vi "MAIN - PECT - Autonics - Pulses - encoder - Multi-sensor - Huy.vi"() -> ()   [LabVIEW 2018]
uses:
  Pulsed Eddy Current - DATN Huy/Control 1.ctl
  <vilib>/DAQmx/read.llb/DAQmx Read (Counter U32 1Chan 1Samp).vi
  <vilib>/DAQmx/write.llb/DAQmx Write (Analog 1D Wfm NChan NSamp).vi
  <vilib>/DAQmx/read.llb/DAQmx Read (Analog 1D Wfm NChan NSamp).vi
  <vilib>/DAQmx/create/channels.llb/DAQmx Create Channel (AI-Voltage-Basic).vi
  <vilib>/NI/Modbus Library/API/Wrapper/Create Serial Master.vi
  <vilib>/DAQmx/create/channels.llb/DAQmx Create Channel (CI-Count Edges).vi
  <vilib>/DAQmx/miscellaneous.llb/DAQmx Fill In Error Info.vi
  <vilib>/DAQmx/configure/timing.llb/DAQmx Timing (Sample Clock).vi
  <vilib>/DAQmx/configure/trigger.llb/DAQmx Start Trigger (Digital Edge).vi
  <vilib>/DAQmx/create/channels.llb/DAQmx Create Channel (AO-Voltage-Basic).vi
  Pulsed Eddy Current - DATN Huy/Global_data.vi
  <vilib>/measure/maspectr.llb/FFT Power Spectrum and PSD for 1 Chan.vi
  <vilib>/NI/Modbus Library/API/Master/Modbus Master.lvclass
  <resource>/objmgr/daqmx.rc
  <vilib>/Platform/NI_3dgraph.lvlib
  <vilib>/measure/NI_MAPro.lvlib
  <vilib>/NI/Modbus Library/API/Wrapper/API Main.lvlib
panel:
  out "Init pulses":i32
  out "Z complete":bool
  out "X complete":bool
  out "Y complete":bool=TRUE
  out "exception status":u8=1
  out "Limit Sensor":bool[](array[boolean])
  out "Y Back Limit":bool
  out "X L Limit":bool
  out "Z UP Limit":bool
  out "Numeric  4":i32=3413
  out "Enum 2":T1(ring)=enum."Wait Y"
  in  "Stop Scan":bool
  out "Step Y Number":i16=20
  out "Count Y step":i32=6
  out "No. Y 2":i32=7
  in  "Open tdms 2":bool
  in  "Backdata 3":bool
  in  "low cutoff freq: fl 4":dbl=40.0 format="%0.2f"
  in  "Filter 4":bool
  out "dy 2":dbl[][](array[numeric])
  in  "DiffX 2":bool caption="Scan"
  in  "DiffY 2":bool caption="Scan"
  in  "Odd 2":bool caption="Scan"
  in  "Abs 2":bool caption="Scan"
  in  "Backdata 2":bool caption="Scan"
  in  "Backindex 2":i32
  in  "low cutoff freq: fl 3":dbl=40.0 format="%0.2f"
  in  "Filter 3":bool caption="Scan"
  in  "Line Row 2":dbl
  in  "Line Col 2":dbl=167.0
  in  "Repair Line Row 2":bool
  in  "Repair Line Col 2":bool
  in  "Trim data 2":bool caption="Scan"
  in  "X-min 2":dbl
  in  "X-max 2":dbl=319.0
  in  "Y-min 2":dbl
  in  "Y-max 2":dbl=55.0
  in  "Inverse  2":bool caption="Scan"
  in  "Return 2":bool caption="Scan"
  in  "ColorMapAutoScale 2":bool=TRUE
  in  "Min 2":dbl=-0.004
  in  "Max 2":dbl=0.004
  in  "Cursor 2":bool=TRUE
  out "Out Hall":dbl[][](array[numeric])=[[0.17776170515535383, 0.1724938890045491, 0.17567422492724655, 0.17281948891164128, 0.17750249452676287, 0.17174255590976084, 0.17689848816282988, 0.0, 0.0, 0.0, 0.0, 0.0, 0.0, 0.0, 0.0, 0.0, 0.0, 0.0, 0.0, 0.0, 0.0], [0.181110419736364, 0.17834435597274723, 0.17901593566948365, 0.17843396121396082, 0.18082391275549609, 0.17677177439859865, 0.1805733450890007, 0.0, 0.0, 0.0, 0.0, 0.0, 0.0, 0.0, 0.0, 0.0, 0.0, 0.0, 0.0, 0.0, 0.0], [0.1901443502075802, 0.1807788163690286, 0.18389219629241077, 0.18292101264388094, 0.18584253413825647, 0.18424340027016872, 0.1844692257000472, 0.0, 0.0, 0.0, 0.0, 0.0, 0.0, 0.0, 0.0, 0.0, 0.0, 0.0, 0.0, 0.0, 0.0], [0.19675174630430725, 0.19133976157012406, 0.19610529224489537, 0.18647717964306243, 0.19791131101721843, 0.19044015693607824, 0.19720754713146932, 0.0, 0.0, 0.0, 0.0, 0.0, 0.0, 0.0, 0.0, 0.0, 0.0, 0.0, 0.0, 0.0, 0.0], [0.20248230005231593, 0.1980001562954143, 0.2026130769874166, 0.19908381606183906, 0.20400329640988507, 0.19691764965481123, 0.2026434189867065, 0.0, 0.0, 0.0, 0.0, 0.0, 0.0, 0.0, 0.0, 0.0, 0.0, 0.0, 0.0, 0.0, 0.0], [0.20756282207197274, 0.20355937318454292, 0.2074345242175782, 0.20456099056442495, 0.2083181459314682, 0.202307939377475, 0.20759286833282414, 0.0, 0.0, 0.0, 0.0, 0.0, 0.0, 0.0, 0.0, 0.0, 0.0, 0.0, 0.0, 0.0, 0.0], [0.2161886923639197, 0.21253974725757924, 0.21125259878099184, 0.20908024033946615, 0.2168660930291072, 0.21166435694559893, 0.21165270992196006, 0.0, 0.0, 0.0, 0.0, 0.0, 0.0, 0.0, 0.0, 0.0, 0.0, 0.0, 0.0, 0.0, 0.0], [0.2201899331796135, 0.21690643861065811, 0.2201028334105652, 0.2176118553302127, 0.2208123356772303, 0.21536349521145187, 0.21956557074351502, 0.0, 0.0, 0.0, 0.0, 0.0, 0.0, 0.0, 0.0, 0.0, 0.0, 0.0, 0.0, 0.0, 0.0], [0.22206492093457092, 0.22076373224143442, 0.22107829951788738, 0.221511549643648, 0.22260408488962002, 0.21964691546696985, 0.22123030620827921, 0.0, 0.0, 0.0, 0.0, 0.0, 0.0, 0.0, 0.0, 0.0, 0.0, 0.0, 0.0, 0.0, 0.0], [0.2236337254628875, 0.22214151901015816, 0.22332887383646616, 0.22254736085515114, 0.2241084117751464, 0.22218723394057438, 0.22207453511184994, 0.0, 0.0, 0.0, 0.0, 0.0, 0.0, 0.0, 0.0, 0.0, 0.0, 0.0, 0.0, 0.0, 0.0], [0.22318899958521138, 0.22380028818012027, 0.22211272800173293, 0.22360354843226388, 0.22304326181333678, 0.22145899165729238, 0.21932588351591875, 0.0, 0.0, 0.0, 0.0, 0.0, 0.0, 0.0, 0.0, 0.0, 0.0, 0.0, 0.0, 0.0, 0.0], [0.22290047278312458, 0.2235340533472822, 0.2222785786896101, 0.22290675514178815, 0.22322972419052123, 0.22156789245679248, 0.22010562695733926, 0.0, 0.0, 0.0, 0.0, 0.0, 0.0, 0.0, 0.0, 0.0, 0.0, 0.0, 0.0, 0.0, 0.0], [0.22356747769441365, 0.2241092575777761, 0.2223606596149607, 0.2229985011040989, 0.2225818108464972, 0.22200716436702206, 0.21966538751675208, 0.0, 0.0, 0.0, 0.0, 0.0, 0.0, 0.0, 0.0, 0.0, 0.0, 0.0, 0.0, 0.0, 0.0], [0.22053633383678345, 0.2227234349622484, 0.22003048978407946, 0.22234284825731204, 0.21996511082210407, 0.22033336393759062, 0.21762783729986052, 0.0, 0.0, 0.0, 0.0, 0.0, 0.0, 0.0, 0.0, 0.0, 0.0, 0.0, 0.0, 0.0, 0.0], [0.21927133576270147, 0.21955591604432806, 0.21646450772183934, 0.21896512302724214, 0.21808932704173967, 0.21754658610019562, 0.21354951646025394, 0.0, 0.0, 0.0, 0.0, 0.0, 0.0, 0.0, 0.0, 0.0, 0.0, 0.0, 0.0, 0.0, 0.0], [0.2185139029939545, 0.21825674506426196, 0.21672810294608302, 0.21719225251047203, 0.2163638216728313, 0.2157054295509772, 0.21285135223872376, 0.0, 0.0, 0.0, 0.0, 0.0, 0.0, 0.0, 0.0, 0.0, 0.0, 0.0, 0.0, 0.0, 0.0], [0.21491616995167662, 0.21811390913005718, 0.21464911868266495, 0.21696465474188015, 0.21574170384074837, 0.21470166777781502, 0.21233935567094664, 0.0, 0.0, 0.0, 0.0, 0.0, 0.0, 0.0, 0.0, 0.0, 0.0, 0.0, 0.0, 0.0, 0.0], [0.2134545034639892, 0.2143867692168009, 0.21070345133335106, 0.21436238496967602, 0.2114824144487502, 0.21274445669186648, 0.20671707318008187, 0.0, 0.0, 0.0, 0.0, 0.0, 0.0, 0.0, 0.0, 0.0, 0.0, 0.0, 0.0, 0.0, 0.0], [0.21091214938658065, 0.21277905859725532, 0.20836885096431412, 0.21055566864121245, 0.20950337819485593, 0.20888585192838677, 0.20574571324326885, 0.0, 0.0, 0.0, 0.0, 0.0, 0.0, 0.0, 0.0, 0.0, 0.0, 0.0, 0.0, 0.0, 0.0], [0.21109980585640742, 0.21000105081453663, 0.2080156676992811, 0.20958712361967385, 0.20811188508169193, 0.20736163569155075, 0.2047283842510788, 0.0, 0.0, 0.0, 0.0, 0.0, 0.0, 0.0, 0.0, 0.0, 0.0, 0.0, 0.0, 0.0, 0.0]]
  in  "Save Scan mode 2":bool caption="Save Process"
  in  "Filter 2":bool
  in  "low cutoff freq: fl 2":dbl=40.0 format="%0.2f"
  in  "Backdata":bool
  out "Init pulses":i32
  out "dy":dbl[][](array[numeric])
  in  "2D Array In":dbl[][](array[numeric])
  out "Output Coil":dbl[][](array[numeric])=[[0.18553710534904855, 0.17973457254507935, 0.18427423395187004, 0.18042918126533436, 0.18645887887248153, 0.1801573678387421, 0.18645082000465146, 0.0, 0.0, 0.0, 0.0, 0.0, 0.0, 0.0, 0.0, 0.0, 0.0, 0.0, 0.0, 0.0, 0.0], [0.18987014602319247, 0.18653261167773033, 0.18990582291953773, 0.18740225957772644, 0.1914559394951999, 0.18644683758905045, 0.191481439134582, 0.0, 0.0, 0.0, 0.0, 0.0, 0.0, 0.0, 0.0, 0.0, 0.0, 0.0, 0.0, 0.0, 0.0], [0.20219420650083397, 0.19081774860606898, 0.1952789240855507, 0.1921933722869305, 0.19679175738266869, 0.19602858652538785, 0.19738356640856358, 0.0, 0.0, 0.0, 0.0, 0.0, 0.0, 0.0, 0.0, 0.0, 0.0, 0.0, 0.0, 0.0, 0.0], [0.20939136336324898, 0.20337450420146508, 0.20975638146138104, 0.19793745902051413, 0.21076173268511106, 0.2028610093026868, 0.21149030184929252, 0.0, 0.0, 0.0, 0.0, 0.0, 0.0, 0.0, 0.0, 0.0, 0.0, 0.0, 0.0, 0.0, 0.0], [0.21622055514910743, 0.2109998977268851, 0.21654153178439584, 0.21186750773282248, 0.21747992176888825, 0.21001144013201994, 0.2178259938557714, 0.0, 0.0, 0.0, 0.0, 0.0, 0.0, 0.0, 0.0, 0.0, 0.0, 0.0, 0.0, 0.0, 0.0], [0.22096639968031884, 0.21613883575961468, 0.22106121776896787, 0.21769696957735463, 0.2229345689672355, 0.2160350775631949, 0.22254631882683024, 0.0, 0.0, 0.0, 0.0, 0.0, 0.0, 0.0, 0.0, 0.0, 0.0, 0.0, 0.0, 0.0, 0.0], [0.22918239447852007, 0.22482125577754608, 0.2251534307015154, 0.22210101570727897, 0.2301739477211303, 0.22526210600970953, 0.22650893519159931, 0.0, 0.0, 0.0, 0.0, 0.0, 0.0, 0.0, 0.0, 0.0, 0.0, 0.0, 0.0, 0.0, 0.0], [0.23072867440456596, 0.2279499722265652, 0.23049599246595942, 0.22892309217776513, 0.23257180417432533, 0.22825736261999474, 0.2320123360222584, 0.0, 0.0, 0.0, 0.0, 0.0, 0.0, 0.0, 0.0, 0.0, 0.0, 0.0, 0.0, 0.0, 0.0], [0.23185337710758436, 0.22989669056911782, 0.2307016748936201, 0.23044598289982565, 0.23299357137415944, 0.23058981164836756, 0.2319131657399408, 0.0, 0.0, 0.0, 0.0, 0.0, 0.0, 0.0, 0.0, 0.0, 0.0, 0.0, 0.0, 0.0, 0.0], [0.22630211132749595, 0.2303770249129905, 0.2282483576289565, 0.23086049593072017, 0.23095666864614767, 0.23114931892992713, 0.22934701981393596, 0.0, 0.0, 0.0, 0.0, 0.0, 0.0, 0.0, 0.0, 0.0, 0.0, 0.0, 0.0, 0.0, 0.0], [0.2215102649364752, 0.22374474076562317, 0.2191382524314066, 0.22801369409819444, 0.22283327835507083, 0.22548194556609513, 0.22129294280866907, 0.0, 0.0, 0.0, 0.0, 0.0, 0.0, 0.0, 0.0, 0.0, 0.0, 0.0, 0.0, 0.0, 0.0], [0.21763039136450935, 0.21929122157454478, 0.21572879699955255, 0.2193674469881774, 0.21916521798106897, 0.22116497510888178, 0.21738430074877346, 0.0, 0.0, 0.0, 0.0, 0.0, 0.0, 0.0, 0.0, 0.0, 0.0, 0.0, 0.0, 0.0, 0.0], [0.21335832760298545, 0.215211494733674, 0.21125095473051608, 0.2160083891793727, 0.21476909785799747, 0.21737423005943346, 0.21311533591657172, 0.0, 0.0, 0.0, 0.0, 0.0, 0.0, 0.0, 0.0, 0.0, 0.0, 0.0, 0.0, 0.0, 0.0], [0.20135894511959307, 0.21145853750149302, 0.2048206322299499, 0.21082245427422058, 0.20181948963267182, 0.20702943348605823, 0.2070025081380047, 0.0, 0.0, 0.0, 0.0, 0.0, 0.0, 0.0, 0.0, 0.0, 0.0, 0.0, 0.0, 0.0, 0.0], [0.19432880055987894, 0.19771187558020858, 0.19098523549555563, 0.1977787364919263, 0.19570997510151694, 0.20082611415153734, 0.19373654419199682, 0.0, 0.0, 0.0, 0.0, 0.0, 0.0, 0.0, 0.0, 0.0, 0.0, 0.0, 0.0, 0.0, 0.0], [0.18896822798166024, 0.19168506258678636, 0.18632412497380157, 0.19159648646157518, 0.1906377348289004, 0.19408935512459574, 0.18912258943210353, 0.0, 0.0, 0.0, 0.0, 0.0, 0.0, 0.0, 0.0, 0.0, 0.0, 0.0, 0.0, 0.0, 0.0], [0.18009702280244988, 0.18712015799094445, 0.1825546829225686, 0.1875327275883079, 0.18680820041773105, 0.18988062347566131, 0.18488384150052983, 0.0, 0.0, 0.0, 0.0, 0.0, 0.0, 0.0, 0.0, 0.0, 0.0, 0.0, 0.0, 0.0, 0.0], [0.17377109719426687, 0.17674354692231936, 0.1701534372729802, 0.18307701834693768, 0.17476744955718027, 0.17999467046652273, 0.17298889884516222, 0.0, 0.0, 0.0, 0.0, 0.0, 0.0, 0.0, 0.0, 0.0, 0.0, 0.0, 0.0, 0.0, 0.0], [0.16752395847442747, 0.17063904093338916, 0.16462749541368465, 0.17056002142642612, 0.16910895941204906, 0.17404342521037897, 0.16819677725831522, 0.0, 0.0, 0.0, 0.0, 0.0, 0.0, 0.0, 0.0, 0.0, 0.0, 0.0, 0.0, 0.0, 0.0], [0.16324428563434706, 0.16559024570855152, 0.16156797333915018, 0.16574386859680224, 0.16542079327972803, 0.1678753304123673, 0.16521948417362342, 0.0, 0.0, 0.0, 0.0, 0.0, 0.0, 0.0, 0.0, 0.0, 0.0, 0.0, 0.0, 0.0, 0.0]]
  in  "Tab Control 3":enum32{"Control", "Data Processing"}(tab)
  in  "Pulser Trigger":tag="/Dev1/PFI0"
  in  "Edge":i32(ring)=10280 items=["Rising"=10280, "Falling"=10171]
  in  "2 Plots":bool
  in  "Offset":bool
  in  "Gate 1":dbl
  in  "Gate 2":dbl=20.0
  in  "Tab Control 4":enum32{"Basic", "Gaussian", "Chirp"}(tab)
  in  "Pulse Basic":T3={"Basic amp"=1.0, "Duty cycle %"=50.0, "Basic freq (Hz)"=50, "Basic Type"=2} {"Basic Type" items=["Sine Wave", "Triangle Wave", "Square Wave", "Sawtooth Wave"]; "Duty cycle %" format="%#.2f"; "Basic amp" format="%0.2p"}
  in  "Pulse Gaussian":T4={"Gauss amp"=2.5, "Gauss Nor. Band"=0.5, "Gauss atten (dB)"=6.0, "Gauss freq (Hz)"=1000.0}
  in  "Pulse chirp":T5={"Chirp amp"=2.1, "Chirp f2"=1500.0, "Chirp f1"=500.0} {"Chirp f1" format="%0.2f"; "Chirp f2" format="%0.2f"; "Chirp amp" format="%0.2f"}
  in  "Gate 3":dbl
  in  "Gate 4":dbl=20.0
  in  "Stop Button":bool
  in  "X Distance":u32=100
  in  "X RIGHT":bool
  in  "X LEFT":bool
  in  "Y Distance":u32=100
  in  "Y FW":bool
  in  "Y BW":bool
  in  "Z Distance":i16=1
  in  "Up Z":bool
  in  "Down Z":bool
  in  "Home 2":bool
  in  "Speed (mm/s) 2":i16=6
  in  "Scan":bool
  in  "Open tdms":bool
  in  "Save Scan mode":bool caption="Save Process"
  in  "Open csv":bool
  in  "Exit":bool
  in  "Cursor":bool=TRUE
  in  "Repair Line Col":bool
  in  "Repair Line Row":bool
  in  "Line Col":dbl=167.0
  in  "Line Row":dbl
  in  "Y-max":dbl=55.0
  in  "Y-min":dbl
  in  "X-max":dbl=319.0
  in  "X-min":dbl
  in  "Inverse":bool caption="Scan"
  in  "ViewMode":i32(ring) items=["cwViewXYPlane", "cwViewXZPlane", "cwViewYZPlane", "cwViewUserDefined"]
  in  "Plot style":i32(ring)=4 items=["cwLine"=1, "cwPoint"=2, "cwLinePoint"=3, "cwHiddenLine"=4, "cwSurface"=5, "cwSurfaceLine"=6, "cwSurfaceNormal"=7, "cwContourLine"=8, "cwSurfaceContour"=9]
  in  "ColorMapAutoScale":bool=TRUE
  in  "Max":dbl=0.029
  in  "Min":dbl=-0.030999999999999996
  in  "low cutoff freq: fl":dbl=40.0 format="%0.2f"
  in  "Filter":bool caption="Scan"
  in  "Backindex":i32
  in  "Backdata":bool caption="Scan"
  in  "Odd":bool caption="Scan"
  in  "DiffX":bool caption="Scan"
  in  "DiffY":bool caption="Scan"
  in  "Abs":bool caption="Scan"
  in  "Trim data":bool caption="Scan"
  in  "Return":bool caption="Scan"
  in  "Tab Control 2":T6(tab)
  in  "Tab plot":enum32{"Raw Signal Plot", "Phase Plot"}(tab)
  out "Hall sensors signal":waveform(dbl)[](graph)=[{"t0"=timestamp(3844381406.018446 s since 1904-01-01), "dt"=3.9999999999999996e-05, "Y"=array[500 elements], "attributes"=variant("NI_ChannelName"=variant(string "Acquisition Task0"), "NI_UnitDescription"=variant(string "Volts"))}, {"t0"=timestamp(3844381406.018446 s since 1904-01-01), "dt"=3.9999999999999996e-05, "Y"=array[500 elements], "attributes"=variant("NI_ChannelName"=variant(string "Acquisition Task0"), "NI_UnitDescription"=variant(string "Volts"))}]
  out "Coil signal":waveform(dbl)[](graph)=[{"t0"=timestamp(3844381406.0184684 s since 1904-01-01), "dt"=3.9999999999999996e-05, "Y"=array[500 elements], "attributes"=variant("NI_ChannelName"=variant(string "Acquisition Task2"), "NI_UnitDescription"=variant(string "Volts"))}, {"t0"=timestamp(3844381406.0184684 s since 1904-01-01), "dt"=3.9999999999999996e-05, "Y"=array[500 elements], "attributes"=variant("NI_ChannelName"=variant(string "Acquisition Task2"), "NI_UnitDescription"=variant(string "Volts"))}]
  out "Phase - Single Hall (0)":cluster{dbl[], "Signal out":dbl[]}[](graph)
  out "Phase - Differential Hall (2)":cluster{dbl[], "Signal out":dbl[]}[](graph)
  out "Feature Extraction Hall":dbl(graph)=0.07041561460174023
  out "Power spectral density Hall":cluster{"f0":dbl, "df":dbl, "magnitude":dbl[]}[](graph)=[{"f0"=0.0, "df"=50.00000000000001, "magnitude"=[0.05344226538018011, 0.49428645675976, 0.17848329749409506, 0.030177691736389706, 0.015779343521924998, 0.006320257971197771, 0.0038168470703960067, 0.0019964659184224885, 0.0013194607149625986, 0.0007909208207930289, 0.0005535851326366026, 0.000358756224441028, 0.0002600365059727909, 0.00017878857903978157, 0.0001359454988281132, 9.993266647353149e-05, 7.753702165794456e-05, 5.8386048558759755e-05, 4.549840057742934e-05, 3.3454980244959085e-05, 2.6622987044468742e-05, 1.9250486167782837e-05, 1.4534022978169584e-05, 1.3228498606348696e-05, 1.2150027857478272e-05, 9.502579643267317e-06, 7.855867434071126e-06, 7.01638103886502e-06, 6.372515227454497e-06, 4.999969117815732e-06, 3.84393580456763e-06, 3.0917208279441807e-06, 2.4082253245390505e-06, 2.0891651026755156e-06, 2.1987810684143896e-06, 1.7457276008966685e-06, 1.3664085555342715e-06, 1.3673912753577668e-06, 1.2138009817051083e-06, 8.606682950932153e-07, 8.041900765492353e-07, 8.749099163659475e-07, 8.132829202518184e-07, 6.822494594419114e-07, 6.049051591521565e-07, 6.132992125073271e-07, 5.773547451807314e-07, 5.506540953194728e-07, 4.3351203976864175e-07, 1.8527694293227517e-07, 1.0481643805680082e-07, 1.195257630817566e-07, 1.1577574640733723e-07, 1.3401572515625924e-07, 1.6216287991758492e-07, 1.186876125279046e-07, 9.060456692020551e-08, 1.3456818799714813e-07, 1.0510266739217573e-07, 3.142357380666471e-08, 1.4252605291150848e-08, 4.94727416899243e-08, 9.493752501187421e-08, 7.628840934796899e-08, 8.59941417276983e-08, 2.117415858805495e-07, 1.81493780415358e-07, 4.825218961205501e-08, 4.191163413423024e-08, 6.441735733140098e-08, 3.4493211155460755e-08, 1.4815146399129527e-08, 2.7635500338646048e-08, 3.31043326742198e-08, 1.2413938930169236e-08, 1.457617162360193e-08, 3.7426355027452554e-08, 8.043740401609367e-08, 1.2269684347819443e-07, 1.246734981592159e-07, 5.2624356236721426e-08, 4.463962736770971e-08, 6.268161110233025e-08, 2.646498245870502e-08, 9.27204135176441e-09, 5.687475791202217e-09, 4.3602539744288816e-08, 5.527470937058986e-08, 1.727347402766435e-08, 2.5880201919013012e-08, 3.474778084083779e-08, 9.148097678816275e-09, 1.3421076340763538e-08, 8.00016733276709e-09, 2.2985544027964692e-08, 2.5069409405287202e-08, 3.0328634642511167e-08, 1.0224838076248899e-08, 9.378180566466623e-10, 2.873099772018073e-08, 1.334279919522608e-07, 1.8727262848664548e-07, 1.3332056211683505e-07, 8.726903720317449e-08, 1.03971846440294e-07, 6.718232618882674e-08, 1.3880802636736537e-08, 3.9650360677896445e-08, 1.2859794341213376e-07, 1.0679933330923813e-07, 5.107625956135357e-08, 5.343601180982578e-08, 5.5313249665534265e-08, 5.1826870346456046e-08, 7.183493774751532e-08, 6.437520957424805e-08, 4.280825959178591e-08, 2.543086465599578e-08, 1.6763998967314607e-08, 3.5619661064757844e-08, 4.890137024737889e-08, 6.082773646809916e-08, 5.888222718893705e-08, 4.1628475463044077e-08, 4.42698534942595e-08, 6.214635675712085e-08, 8.99759237288563e-08, 1.3448108318958237e-07, 6.113750683434083e-08, 2.103047358584125e-08, 2.8362017906722262e-08, 5.481610867729404e-08, 1.0688808193659075e-07, 1.7274313715049422e-07, 1.914756881569332e-07, 1.1306438838635857e-07, 5.2813427257792266e-08, 3.996199556144808e-08, 2.2697571013294733e-08, 5.734483892419069e-10, 2.8081260393893844e-08, 2.8880224924120155e-08, 4.898407391043184e-08, 5.664197632494949e-08, 2.8532162294421515e-08, 2.8853144610438315e-08, 5.559791052549845e-08, 4.446329519051906e-08, 1.6680834898830503e-08, 3.5650802925485585e-08, 3.848002231692065e-08, 1.9680536607976463e-08, 2.7851839333979786e-08, 3.8933105523131193e-08, 2.87184748099256e-08, 2.0485065158311178e-08, 4.136069598939249e-08, 7.319940383893738e-08, 8.004455591882947e-08, 9.602410245361758e-08, 6.666789751788917e-08, 4.995816124195714e-08, 6.683357512271323e-08, 1.0087542956994011e-07, 6.827798428718567e-08, 5.4876548151163396e-08, 5.744632982652637e-08, 4.929962484905926e-08, 2.9032444367342632e-08, 1.522487958403537e-08, 2.026435224314862e-08, 5.0457006209631696e-08, 8.373272899679024e-08, 1.0790271945291921e-07, 7.018845544482759e-08, 2.411772863403995e-08, 2.360453514128649e-08, 4.077274184419568e-08, 7.648209134497276e-08, 1.2781018650491652e-07, 1.6002774083664143e-07, 2.0770049365059966e-07, 1.303222414400018e-07, 4.1368308120012236e-08, 6.4160316739485e-08, 1.0099067934493672e-07, 5.38019209498868e-08, 4.4635898377098715e-08, 5.9315721166343063e-08, 7.226181891616877e-08, 7.063800286754404e-08, 8.760300104088728e-08, 6.872173578943062e-08, 5.8742115186723415e-08, 7.553788068378707e-08, 8.671207764860681e-08, 9.022251590094401e-08, 5.9593987724185115e-08, 3.582920024686291e-08, 5.798093672933093e-08, 9.499750095191987e-08, 6.926474282663654e-08, 3.293710896704422e-08, 2.8245758802593293e-08, 2.47091803072218e-08, 1.2647196881118485e-08, 6.454242521098473e-08, 2.056831730517149e-07, 3.485617433452981e-07, 1.440427212693921e-07, 8.937883626262774e-08, 6.045562377904082e-08, 7.760808515413506e-08, 7.78449152515259e-08, 1.330054212144905e-07, 8.371828606658445e-08, 8.561279979854768e-08, 5.4805119006428505e-08, 1.9338255465860983e-08, 3.683299630853313e-08, 1.2478751634611085e-07, 1.16562391672607e-07, 6.171400516822817e-08, 3.763791730789338e-08, 5.177315424560907e-08, 1.0221161051269428e-08, 1.6685563679185154e-08, 7.024939423457463e-08, 3.8696218795106824e-08, 4.90292594838444e-08, 7.457546634166207e-08, 3.9335458612916186e-08, 4.519700704403511e-08, 5.1748360032004634e-08, 4.5665543598436463e-08, 4.248858006809279e-08, 1.6997037841459297e-08, 3.430110823042511e-08, 1.0024033470712759e-07, 2.5382392312075055e-07, 2.3195388950002645e-07, 9.90307775433233e-08, 4.93160412832673e-08, 5.42909961897056e-08, 8.79319646977936e-08, 1.1705999824246691e-07, 9.089424254070586e-08, 8.65613061805912e-08, 4.3020212897029436e-08, 2.947213234013073e-08]}, ...(2 in all)]
  in  "Add LF":bool
  in  "Save LF":bool caption="Save Process"
  out "Save Status":bool
  out "Power spectral density Coil":cluster{"f0":dbl, "df":dbl, "magnitude":dbl[]}[](graph)=[{"f0"=0.0, "df"=50.00000000000001, "magnitude"=[0.06471500798999083, 0.10490788754209399, 0.024608636483418194, 0.00438296652656786, 0.002353975865329042, 0.0009930276997905318, 0.0006133065242780386, 0.00033234531696222833, 0.00022234291389610391, 0.00013599912790488415, 9.635500158173878e-05, 6.385727017592712e-05, 4.6859522684514546e-05, 3.264012477373104e-05, 2.494329649951874e-05, 1.8795482156107153e-05, 1.4930372858996385e-05, 1.1087730773346793e-05, 8.699885164366403e-06, 6.843723008639812e-06, 5.317177853272812e-06, 3.41854349089057e-06, 2.36216089696049e-06, 2.1094327824092687e-06, 2.0368607532845296e-06, 1.6593921378545388e-06, 1.4388189907875578e-06, 1.2481486541694899e-06, 1.0642889452659768e-06, 8.613808389720096e-07, 7.482731111154614e-07, 6.136253742461639e-07, 4.81930548536851e-07, 3.954701004182598e-07, 3.513657300513881e-07, 3.238765422331869e-07, 3.0808559066308883e-07, 2.574714929256103e-07, 2.006304851630887e-07, 1.7232288780124035e-07, 1.74089583300975e-07, 2.0239764287870447e-07, 1.5608094005219732e-07, 9.48375551237609e-08, 6.48312719107151e-08, 6.950179885773663e-08, 7.350122180875951e-08, 5.508849073841518e-08, 5.071471481648698e-08, 4.917024594063803e-08, 3.927019581297804e-08, 2.865493472218875e-08, 3.042033750079982e-08, 6.356484151502967e-08, 1.131628012005958e-07, 8.770917166116928e-08, 3.849460559005413e-08, 2.2406249338970256e-08, 2.937327972394305e-08, 3.310271947962208e-08, 1.1549285476783957e-08, 1.7582027257628245e-09, 1.4746810230328445e-08, 2.807809650305719e-08, 1.6582601363499622e-08, 9.220284715723395e-09, 7.0570358343042344e-09, 6.103347806248802e-09, 4.221061890242989e-09, 3.29155017051343e-09, 7.897537312045454e-09, 1.4800804144644369e-08, 4.440147699567223e-09, 1.0836774053742844e-09, 5.201310588053047e-09, 5.118692316685894e-09, 3.876120411759733e-09, 8.967137960534486e-09, 9.553480760753523e-09, 1.1845491620801643e-08, 2.3465172488569197e-08, 9.095409630592785e-09, 8.058804655606744e-11, 1.240856877775084e-09, 1.7554291563382184e-09, 1.622786769483243e-09, 4.420811206107678e-09, 1.373011919379434e-09, 9.06932764250493e-10, 6.434932109627647e-09, 5.347572186368814e-09, 5.105133310237453e-10, 1.5238772528762543e-09, 3.293426245111752e-10, 1.9485625928318283e-09, 6.049833707988641e-10, 1.718304607563343e-10, 2.6250789895257948e-09, 5.5550450795021446e-09, 2.7634365616250577e-08, 9.411828662332091e-09, 3.4355126362302166e-09, 1.6483930375292411e-09, 3.867637310330051e-10, 8.189858566467442e-10, 4.2588387800610776e-10, 1.61835031977466e-10, 2.626872780519488e-10, 8.581641561567351e-11, 7.80504543979124e-12, 3.2469404845402755e-10, 1.7766378925106262e-09, 6.077120737227311e-09, 2.821313239672745e-09, 5.32267129177698e-10, 6.266532314362268e-10, 1.3521566313179728e-09, 5.191683970545212e-09, 1.163702854741034e-08, 2.0866295709393846e-09, 1.2920350149377133e-09, 6.107268669825776e-09, 1.6234830727552773e-10, 1.7218304307096456e-09, 8.998944730098978e-10, 5.603077667795519e-10, 2.0224103608600164e-11, 8.075749738337876e-10, 8.721436588670355e-10, 3.719772495742986e-09, 1.0053169486957145e-08, 5.732860604673989e-09, 6.783660147802078e-09, 7.387782843284888e-09, 1.993319164824313e-09, 1.6871109342383448e-09, 3.851787498335101e-09, 7.602739813531432e-09, 2.6373743491907912e-09, 5.2367883185127045e-09, 1.570231387120171e-08, 1.09351649028092e-08, 4.232403685987372e-10, 1.4075809200037895e-09, 2.787101906083711e-09, 1.0243605792229125e-09, 1.5243819649117444e-09, 3.2668878550539542e-09, 7.165093854380813e-10, 7.178026024792953e-10, 7.163021793593579e-10, 4.871253272759402e-10, 3.3689325374539587e-10, 9.053388742882745e-11, 8.47060497268097e-11, 2.1652333307865178e-09, 5.191374000359224e-09, 3.3378619778986655e-09, 9.376805315277407e-10, 6.08880694148336e-09, 1.799287902931768e-08, 1.2384703881624945e-08, 5.638582625124952e-09, 6.089830350784959e-09, 4.625327984411809e-09, 4.797001785380629e-10, 3.671051025949149e-10, 8.53389739031635e-11, 1.5881648376439475e-09, 3.4395750302534926e-09, 2.0484015898175548e-10, 1.0876714876357938e-09, 1.6779654532955758e-09, 5.983518496933457e-10, 1.3703546979604813e-09, 3.2035261954833246e-09, 7.810457738849178e-09, 7.2786525235643386e-09, 1.831757381309426e-09, 6.583986610268209e-09, 4.140399669972484e-10, 9.225786631998565e-09, 1.3840054204595343e-09, 1.3087651452104364e-09, 5.772885567196273e-11, 6.238654484291674e-10, 8.446631955649547e-10, 9.60692639300278e-10, 2.2946669800416606e-09, 4.706636927790736e-09, 1.7195422401010414e-09, 6.01554636790235e-11, 1.642314657027999e-10, 2.8796861842033897e-10, 3.2576579035771345e-09, 1.8622191268493826e-09, 1.9406625842261643e-10, 1.3260249218513399e-11, 2.159251486310598e-09, 1.6170719715144243e-10, 1.1601067375548019e-08, 3.5900131143046976e-09, 9.364895039775729e-09, 3.445950995939315e-09, 3.0458082145416376e-09, 7.482201199742227e-09, 1.1097609412351321e-08, 1.3446550609020134e-08, 1.489395795604217e-08, 1.0079340393933278e-08, 6.315023670817954e-09, 4.357683135105497e-09, 1.49205808331129e-09, 7.839934048851647e-11, 2.4283097582485266e-09, 1.345921525360762e-09, 1.959664996621814e-09, 2.205548803551967e-09, 2.101968548459717e-09, 6.37233042080121e-11, 4.613313544458869e-09, 3.1937453382577165e-09, 2.458251239608534e-10, 6.862155147694832e-10, 2.5231468014641028e-09, 1.1876874679348104e-09, 2.242941481809397e-10, 1.7173319537765193e-09, 1.7737522349175943e-09, 6.66562449000842e-10, 4.2473960553661253e-11, 1.937616215730229e-10, 1.8322341333968375e-10, 1.0073689561157657e-09, 8.497702108980565e-10, 7.862843619019232e-10, 4.355940466970832e-09, 9.144546500898896e-10, 2.5311893509022874e-09, 1.604116612745175e-08, 1.2890611449264356e-08, 3.7170575844336277e-09, 2.0417543694612313e-09, 3.639916957099234e-09, 5.6594996184529875e-09, 2.903222776721938e-09, 3.3605212419772653e-09, 2.0340648284100022e-08, 1.408153004705747e-08, 5.873974395123851e-09]}, ...(2 in all)]
  out "Feature Extraction Coil":dbl(graph)=0.1511557759031275
  out "Save Status 2":bool
  in  "3D Surface(0) (coil)":refnum<k7>(container)
  out "Record path":path=path "C:/Users/ADMIN/Downloads/PECT_default.tdms" caption="selected path"
  out "Feature extraction scan Coil":dbl[](graph)
  in  "3D Surface (2)(Hall)":refnum<k7>(container)
  out "Feature extraction scan Hall":dbl[](graph)
  out "Record path 2":path=path "C:/Users/ADMIN/Downloads/PECT2_default.tdms" caption="selected path"
  in  "View Mode":bool caption="Scan"
  out "Hall sensors signal lf":dbl[][](graph)=[[-0.70660846198, -0.716567731313, -0.71772803455, -0.717921418426, -0.720596562008, -0.722079171705, -0.724657623384, -0.723561781416, -0.729298836376, -0.728847607304, -0.733553281611, -0.731232675116, -0.734068971955, -0.734230125187, -0.734649123582, -0.735197044564, -0.737292036575, -0.735906118769, -0.738162264033, -0.736454039766, -0.735454889741, -0.737968880154, -0.735422659102, -0.737292036581, -0.734552431644, -0.735809426849, -0.731909518652, -0.731264905752, -0.726591462081, -0.727171613726, -0.72340062815, -0.721080021693, -0.715278505501, -0.71253890069, -0.707188613582, -0.701870557272, -0.697068191179, -0.692362517146, -0.687946918849, -0.677826496722, -0.674571201711, -0.663773936246, -0.660776486438, -0.651622983945, -0.644113244288, -0.636120045089, -0.629867300614, -0.618425422989, -0.610399993434, -0.59950603696, -0.59218968167, -0.58322956384, -0.571207535404, -0.564471331877, -0.553126147145, -0.546615558225, -0.534915836753, -0.528792015616, -0.520315358066, -0.514803919133, -0.504103347861, -0.497753912499, -0.490534250062, -0.48415258421, -0.4781254554, -0.472839631231, -0.469197569495, -0.467811652195, -0.46571666097, -0.462429136198, -0.467457115235, -0.467231500771, -0.474354471106, -0.474741238726, -0.482927820085, -0.490469788806, -0.499204291135, -0.509066865834, -0.523216115386, -0.534432377128, -0.554350911396, -0.569177005115, -0.58816085171, -0.612366062487, -0.634250667901, -0.66187232831, -0.688269225307, -0.719081721676, -0.746928999864, -0.781093486223, -0.813130751347, -0.851227380515, -0.888357092222, -0.928000797226, -0.965807357181, -1.008351826422, -1.048994689492, -1.09189370194, -1.13485717869, -1.180109036257, -1.2251352826, -1.266293851833, -1.314639865003, -1.35380013893, -1.401147008934, -1.441370901989, -1.48307740981, -1.522592234217, -1.561881446939, -1.594208832793, -1.628276678402, -1.656575231322, -1.685228323683, -1.708627813295, -1.726709237842, -1.745338585167, -1.754749951221, -1.765386084343, -1.766481928394, -1.766578620469, -1.759068865834, -1.749141808352, -1.726870391409, -1.702697363978, -1.672142659225, -1.635496354594, -1.591855992024, -1.542736415895, -1.486816169566, -1.426544787201, -1.357119898907, -1.281152192711, -1.205055574576, -1.115615471107, -1.027496838527, -0.924487655795, -0.823476790057, -0.71266782326, -0.598377964549, -0.477738687781, -0.356454816131, -0.226146385508, -0.096933813379, 0.039691785785, 0.177477671952, 0.315553620416, 0.456562543074, 0.59605661768, 0.738386978448, 0.878138885599, 1.019921318004, 1.154935322631, 1.292076548544, 1.418613908244, 1.546504957955, 1.665822671713, 1.781143796386, 1.887472587349, 1.990352709737, 2.080759590593, 2.164752584475, 2.235692182322, 2.298122899903, 2.352689348501, 2.387788500997, 2.419503438832, 2.429204857999, 2.432524612792, 2.418181983039, 2.390753718718, 2.346694452024, 2.29477091497, 2.222380935278, 2.137904477937, 2.035346650361, 1.920347813654, 1.791425361517, 1.644195932762, 1.485299034053, 1.310738069287, 1.125154243505, 0.921650202866, 0.71092650171, 0.483765177519, 0.253445229601, 0.008105779367, -0.246129373952, -0.508261099919, -0.779449723152, -1.058244889529, -1.341584711586, -1.635528585329, -1.928441259944, -2.223868134907, -2.526772774422, -2.823650514512, -3.124106146674, -3.41405481644, -3.706227714753, -3.987442417835, -4.263822791101, -4.527407776882, -4.786577416573, -5.02840704592, -5.262275871216, -5.475098028081, -5.677574208879, -5.860454027961, -6.026509320014, -6.174450790588, -6.300217254762, -6.406645020668, -6.487352250666, -6.552781862445, -6.587011551361, -6.605834660103, -6.593973522799, -6.560743004097, -6.502017506172, -6.420568948967, -6.309918874295, -6.178350774499, -6.019772990024, -5.841921080871, -5.636479455639, -5.407702708707, -5.163100759281, -4.889329996495, -4.60340849308, -4.29102572782, -3.966589007543, -3.624329025262, -3.267791211866, -2.894429352616, -2.512784620922, -2.118957082525, -1.720230866355, -1.310095339563, -0.893610688781, -0.473226398891, -0.047749885035, 0.377081857903, 0.806651402224, 1.226326113266, 1.646645459066, 2.057327931374, 2.465367624173, 2.856937640696, 3.240772514315, 3.608041067282, 3.955230157274, 4.293975068757, 4.609804197942, 4.90271751193, 5.177098363499, 5.426887322034, 5.649860408204, 5.851142279943, 6.021772700426, 6.172194436626, 6.288354759714, 6.38169561436, 6.443353457295, 6.479452149573, 6.483029788153, 6.46127387881, 6.407834927929, 6.330674003129, 6.221217696105, 6.086943623705, 5.925176659162, 5.736206928573, 5.524965806055, 5.286167477957, 5.029771319924, 4.744593282131, 4.446168641795, 4.123506733751, 3.788113950506, 3.432351621052, 3.06650133258, 2.685180548865, 2.296898136162, 1.899107838935, 1.494871524426, 1.086445286821, 0.675762909712, 0.265467248353, -0.150952337452, -0.55870204758, -0.972221258056, -1.373654237756, -1.777923829368, -2.168979184481, -2.552460698049, -2.920729689806, -3.280071163481, -3.622008401497, -3.950860315772, -4.258117910152, -4.550936409787, -4.823256343074, -5.072595856712, -5.304498634402, -5.509682053404, -5.698202166799, -5.859132548236, -6.000240858013, -6.111889905191, -6.206424214181, -6.27008099717, -6.315365963394, -6.333898960157, -6.329676659853, -6.305148642671, -6.25857442753, -6.185216035338, -6.09506518857, -5.986381425725, -5.856360663809, -5.709708700472, -5.54117189352, -5.365641079165, -5.166356100054, -4.957401996174, -4.734878834588, -4.502332058483, -4.25769890765, -4.007715673153, -3.745098175872, -3.482835479658, -3.212193012196, -2.937618633024, -2.664784953904, -2.386601188071, -2.116185239442, -1.843835631437, -1.575257184583, -1.307226809354, -1.048865766862, -0.789924683906, -0.543553647601, -0.298858680926, -0.065186650983, 0.160975596988, 0.377855392589, 0.583937909112, 0.777321550784, 0.961906228802, 1.129988834268, 1.286113886493, 1.434406905534, 1.559977352138, 1.681841284773, 1.782239637185, 1.87196966226, 1.947711605492, 2.009916693762, 2.057166778279, 2.095037754511, 2.114505048262, 2.126913836672, 2.123561852274, 2.106834160961, 2.083724807448, 2.04517698859, 1.999828510872, 1.941362174369, 1.876127411384, 1.800417702224, 1.720518017024, 1.626759173182, 1.53477301667, 1.432666452766, 1.3256930704, 1.216753623473, 1.100658983649, 0.982533816097, 0.864892106737, 0.741448886061, 0.618489120633, 0.497011957912, 0.371215886709, 0.252865078568, 0.127455756566, 0.00929831228, -0.108053378055, -0.221569636608, -0.333216531681, -0.440351151746, -0.547066787125, -0.643984321714, -0.742481170629, -0.834016212751, -0.919943133402, -1.004129610016, -1.078743591058, -1.154131117554, -1.220526296559, -1.28176457554, -1.335299729295, -1.389318348703, -1.430928160202, -1.472151206875, -1.504381894686, -1.533711822363, -1.557723687612, -1.576417489536, -1.58798830868, -1.597464132915, -1.601750815379, -1.601621892616, -1.59852774587, -1.588246154234, -1.580027327232, -1.560882295453, -1.54560494743, -1.52268892626, -1.50177120885, -1.474117278751, -1.447236886611, -1.415296278632, -1.385869665753, -1.349996918726, -1.315800169399, -1.280926577982, -1.245472836775, -1.210728172549, -1.170472066246, -1.137048863988, -1.097276222791, -1.065400096546, -1.027077839927, -0.994814949512, -0.958942227201, -0.927646259992, -0.892128078709, -0.861283343899, -0.830664225057, -0.801817793355, -0.772777978979, -0.746928999873, -0.722723784605, -0.697132652466, -0.677504190288, -0.654072512801, -0.640019952773, -0.620713798494, -0.607112468066, -0.589804614323, -0.577589201926, -0.565986171871, -0.555930212629, -0.54590648416, -0.539105819592, -0.533239843546, -0.528050710938, -0.523635113662, -0.51996082103, -0.521346738438, -0.518703826188, -0.521314507795, -0.519896359761, -0.525472259972, -0.524408648935, -0.530177933006, -0.532079540602, -0.538815743842, -0.541813193149, -0.548871702871, -0.55319060837, -0.559572274784, -0.565953941223, -0.570885229012, -0.57865281302, -0.584647711969, -0.594349134521, -0.597120969574, -0.607305851908, -0.611399143265, -0.6213584113, -0.626902081599, -0.634282898507, -0.640019952747, -0.647046232714, -0.651300677507, -0.657295577056, -0.662162404096, -0.668737455294, -0.674216664635, -0.675602582331, -0.683531320648, -0.684949468998, -0.693136052559, -0.694167433224, -0.700516870141, -0.703095321724, -0.708961299059, -0.708219994242, -0.711443058732], [-0.711700903907, -0.720274255531, -0.721080021681, -0.724464239466, -0.722433708801, -0.725141083016, -0.72559231207, -0.726204694336, -0.729202144406, -0.727848457275, -0.731039291205, -0.729975679907, -0.73139382833, -0.73123267509, -0.734165663872, -0.732392978358, -0.735648273607, -0.732908668699, -0.73590611877, -0.734810276807, -0.73352105101, -0.733843357422, -0.732844207425, -0.733230975136, -0.731007060611, -0.73062029283, -0.728106302452, -0.729427758908, -0.724174163692, -0.726043541112, -0.72166017329, -0.721208944256, -0.715181813577, -0.712248824884, -0.70754315068, -0.704739084581, -0.697809495981, -0.693361667074, -0.688849376879, -0.681694173927, -0.676311656471, -0.666481310252, -0.663677244331, -0.654942740122, -0.649270147063, -0.638827419012, -0.632703597094, -0.62161625644, -0.613816441327, -0.601891104324, -0.593382215333, -0.583906407255, -0.574301676729, -0.564729176965, -0.553480684115, -0.54616432927, -0.535624910724, -0.527373867557, -0.517382370077, -0.511258549117, -0.498881984754, -0.493789544277, -0.484603813104, -0.479898140329, -0.472710708686, -0.46910087758, -0.464072898546, -0.462042368558, -0.459721762867, -0.45836807625, -0.458948227649, -0.460366375577, -0.465104278851, -0.467167039506, -0.476352770465, -0.481703055936, -0.495368845435, -0.504619038035, -0.520702125685, -0.534819144789, -0.554447603261, -0.570530691961, -0.592511988075, -0.615621357208, -0.640535643041, -0.667319306976, -0.694973199311, -0.727912918571, -0.7584675715, -0.795017126404, -0.828988231267, -0.870404618505, -0.908050021807, -0.951432484146, -0.989754736086, -1.033685125354, -1.077228749861, -1.121674836208, -1.166572155322, -1.211276093955, -1.257140340429, -1.302521130597, -1.347934155322, -1.389930731637, -1.437535450536, -1.478565113577, -1.521947620419, -1.557949302468, -1.598431053803, -1.629565906268, -1.663762677273, -1.691223234113, -1.718941638241, -1.740310595099, -1.759874633465, -1.772831377568, -1.782081590668, -1.788237655914, -1.788173194541, -1.784176586682, -1.7728636083, -1.758134175287, -1.733090917251, -1.706693971085, -1.669886510205, -1.632917898781, -1.584314009521, -1.53206805716, -1.471442131748, -1.407141915873, -1.333398119264, -1.254561886613, -1.168796071461, -1.07871136044, -0.983147451101, -0.877076363675, -0.77200444347, -0.655490661079, -0.541426425506, -0.414760028952, -0.290317564379, -0.158687687189, -0.026832212351, 0.113370977212, 0.253509690839, 0.395968995891, 0.538202675996, 0.682209031094, 0.82640876359, 0.965999515658, 1.107943100394, 1.2432149505, 1.379195876537, 1.506635696159, 1.632560682823, 1.748236342269, 1.865201233481, 1.969338348306, 2.067416114716, 2.15692054372, 2.236530178481, 2.30560040478, 2.364485757723, 2.409930942223, 2.44470779056, 2.468332842109, 2.474327739345, 2.470137757407, 2.448124237269, 2.417408447956, 2.366355134083, 2.304955792292, 2.22576515062, 2.134197956683, 2.022454403625, 1.899978065497, 1.759420364327, 1.606872887466, 1.438564653815, 1.256074962083, 1.059951729476, 0.851161868759, 0.630478906609, 0.399030903911, 0.159009529445, -0.095741280337, -0.355101129604, -0.628997073303, -0.906148413194, -1.193065765257, -1.484979020361, -1.782984050494, -2.083052046727, -2.385956572993, -2.689473733606, -2.994473784422, -3.295767585382, -3.589680826897, -3.885270392832, -4.167097682705, -4.447442674322, -4.711382413403, -4.969939881134, -5.21305896681, -5.445155293591, -5.65475453306, -5.853298698642, -6.032053093797, -6.193563935177, -6.333222102904, -6.451672172544, -6.551138064005, -6.625721405834, -6.678709764359, -6.705397338156, -6.7118436127, -6.689732892102, -6.647219721964, -6.571991743565, -6.476812606234, -6.354849306761, -6.207552308847, -6.03563076211, -5.840825219647, -5.620911798473, -5.380693017663, -5.114625193963, -4.828993469243, -4.526666463854, -4.200843492433, -3.861516208625, -3.502302924475, -3.13216385381, -2.744427224852, -2.350406050506, -1.943944235937, -1.534034129331, -1.111328792601, -0.688108072092, -0.254348183817, 0.180185043615, 0.614653678333, 1.048574325895, 1.479626447166, 1.903394510606, 2.321264488474, 2.731753822843, 3.124806592014, 3.511768013492, 3.874782309212, 4.221391454251, 4.556655670645, 4.868101642753, 5.155503714809, 5.423470852265, 5.66481553335, 5.882245096744, 6.070795930585, 6.233626609533, 6.371091627426, 6.475326584487, 6.555807348401, 6.601285277357, 6.622976737884, 6.609955415071, 6.570891451368, 6.499628742443, 6.407544849292, 6.28052263845, 6.128070288235, 5.948608528303, 5.743491108137, 5.514426315553, 5.258964657354, 4.982101962969, 4.683548195569, 4.366655388863, 4.026975726542, 3.675113132109, 3.302687625615, 2.924912076204, 2.52876527563, 2.127365065353, 1.717166033533, 1.303228338131, 0.883199090654, 0.465587113791, 0.041722314718, -0.374858506392, -0.792632058415, -1.209664560433, -1.619703313065, -2.022973968836, -2.416640254231, -2.801153418931, -3.170164003204, -3.529376856542, -3.867414465728, -4.195654308351, -4.499141189584, -4.786964188961, -5.051871271029, -5.297149939141, -5.518352233991, -5.717154105289, -5.893104251006, -6.046299304766, -6.173645008773, -6.275238003521, -6.35791128069, -6.408675593623, -6.444194505839, -6.448062264612, -6.433687095446, -6.394268196495, -6.335252674733, -6.248389341404, -6.145345955566, -6.020353152397, -5.879180364564, -5.71757311064, -5.538109933487, -5.346721406584, -5.136058870085, -4.916694164197, -4.681472020658, -4.438804768894, -4.185340402521, -3.926783816261, -3.653465746224, -3.381437188134, -3.103252801735, -2.823908360859, -2.542275774546, -2.258999645662, -1.980912873448, -1.705791511432, -1.431605004604, -1.161544171119, -0.901281584442, -0.641986021923, -0.394615883648, -0.147374738228, 0.083364272888, 0.312008253063, 0.526470734451, 0.730973938979, 0.921811355892, 1.10391427476, 1.267806902505, 1.422997270747, 1.563135951752, 1.687868408833, 1.801094545084, 1.89701284902, 1.981811596561, 2.050430579225, 2.106834160953, 2.147799278231, 2.17816052264, 2.190633772981, 2.194823753727, 2.183317421989, 2.162238596067, 2.128299753321, 2.084208266714, 2.0311889008, 1.967017743996, 1.893370789696, 1.81256864297, 1.725739375948, 1.627307093536, 1.528359125728, 1.41655114942, 1.30799846779, 1.188100615371, 1.068557301022, 0.944695085629, 0.822992319382, 0.695069043221, 0.570272131299, 0.442284382926, 0.317616379586, 0.194624359058, 0.068441497018, -0.050553949051, -0.171128708146, -0.285160663856, -0.399676092901, -0.508132177389, -0.615073436322, -0.712184363585, -0.810874605876, -0.899960127607, -0.986692823527, -1.067462858994, -1.142721461342, -1.214112393046, -1.278251431973, -1.337298031367, -1.389382810045, -1.440339520092, -1.481240260618, -1.520884007654, -1.548602401773, -1.57802902429, -1.595723675412, -1.612902636098, -1.621959461795, -1.628502293261, -1.629275830005, -1.627986602099, -1.618188470277, -1.608358107981, -1.59524021497, -1.575482799408, -1.556627844048, -1.531455674043, -1.507895039751, -1.477243655394, -1.44794596169, -1.414168204733, -1.38277552038, -1.345710238439, -1.31270602436, -1.274061444278, -1.238059782054, -1.200704434038, -1.16164086315, -1.124865672142, -1.086188874377, -1.050283915983, -1.013218656049, -0.978731850936, -0.941376519413, -0.91175654708, -0.874530142074, -0.846586166678, -0.814258824097, -0.786379312543, -0.757500652045, -0.731554981564, -0.705641542641, -0.684433778674, -0.659003801079, -0.639955491476, -0.622712098238, -0.603212560587, -0.590352535192, -0.573463680108, -0.562601954829, -0.551933613494, -0.542554497827, -0.532853075905, -0.529694473448, -0.52025089677, -0.519058363199, -0.513837000046, -0.511451932947, -0.512870080968, -0.511838700566, -0.511677547393, -0.514352690234, -0.517285678205, -0.520508741861, -0.526568101624, -0.527825096497, -0.538493437484, -0.540427275726, -0.547389093516, -0.553061685838, -0.559540044149, -0.566147325069, -0.57620328444, -0.578652813016, -0.588676541915, -0.596540818049, -0.602116718805, -0.61207598672, -0.616749429656, -0.626450852631, -0.6339605921, -0.639955491487, -0.645563623199, -0.654459280486, -0.657263346399, -0.666739155394, -0.66922091493, -0.67573150487, -0.681823096537, -0.68501393027, -0.690783215552, -0.69532773638, -0.698035110534, -0.70357878138, -0.706382847481, -0.706995229747, -0.714827276494, -0.711829826488, -0.717115652296], [-0.710927368415, -0.721563481368, -0.721595712031, -0.723303936229, -0.725108852432, -0.725527850816, -0.729427758978, -0.727300536363, -0.732876438089, -0.733166513892, -0.737034191399, -0.735003660722, -0.738549031766, -0.738452339841, -0.737968880135, -0.738903568875, -0.741095252863, -0.738645723707, -0.741030791566, -0.739677104411, -0.739354797941, -0.742094402897, -0.73774326562, -0.742932399702, -0.737743265618, -0.738968030203, -0.735519351038, -0.735035891386, -0.730845907349, -0.72978229604, -0.724464239482, -0.723819626589, -0.716019810351, -0.714408278121, -0.708574531326, -0.703063091172, -0.698679723421, -0.692878207473, -0.688398147883, -0.678213264461, -0.674829046864, -0.664257395879, -0.659519491377, -0.650656064667, -0.642179405778, -0.633799438886, -0.625226088263, -0.614525515429, -0.606081087604, -0.593478907265, -0.587516238926, -0.577041281088, -0.564471331913, -0.558605355655, -0.545197410173, -0.540781812775, -0.528276325465, -0.521250046516, -0.512773389061, -0.505295881372, -0.496013458178, -0.490598711337, -0.480768367493, -0.477255228246, -0.470325641713, -0.466393504254, -0.46226798305, -0.458819305132, -0.460559759439, -0.456659852641, -0.462429136215, -0.463879514767, -0.471389252665, -0.472517324904, -0.483153434512, -0.490502019438, -0.50084805357, -0.513160156676, -0.528147402851, -0.542361113995, -0.561699496934, -0.579780885408, -0.602664639692, -0.627611155718, -0.650108143758, -0.682467709413, -0.707704303918, -0.742610093227, -0.773390361308, -0.810391146154, -0.844877942157, -0.884070415338, -0.922714969748, -0.965130513384, -1.004194071312, -1.050251685316, -1.092699468449, -1.135695176079, -1.183235411066, -1.227133584269, -1.276382052832, -1.317637317973, -1.366466795995, -1.408012144306, -1.454714405619, -1.494777149486, -1.537934042904, -1.57635302815, -1.614095171865, -1.647905173327, -1.679620181747, -1.706984047416, -1.734025607719, -1.755845795159, -1.771058688734, -1.787077350425, -1.793910260671, -1.803063782041, -1.796939947333, -1.794844951197, -1.782500589886, -1.765353853546, -1.740826286392, -1.711657499304, -1.673367425821, -1.633207975063, -1.581703323307, -1.527845836705, -1.464705918282, -1.396151253222, -1.324856989698, -1.238930010223, -1.155291421567, -1.061242341096, -0.964228054985, -0.855095058719, -0.747960380555, -0.628481383047, -0.509260249656, -0.382271551645, -0.252317654314, -0.117787026094, 0.01909642047, 0.16013760098, 0.300663077532, 0.445829750017, 0.592833556893, 0.73248877748, 0.882199941889, 1.021210542207, 1.165829267176, 1.303453952372, 1.438274578348, 1.570484530423, 1.696796287823, 1.813857867449, 1.930307073514, 2.031124439534, 2.130330282341, 2.219673563048, 2.293578381865, 2.362261844503, 2.416119222821, 2.462434636828, 2.491828971774, 2.511876424447, 2.513326802871, 2.507525289189, 2.480902787945, 2.44390202482, 2.389980183652, 2.321103335349, 2.237626019648, 2.138613551575, 2.020552797226, 1.892371640636, 1.746141352558, 1.583860232908, 1.41087856266, 1.216528009233, 1.019792395584, 0.801139968617, 0.572592735082, 0.334891987588, 0.086426181539, -0.174448462454, -0.439416463364, -0.719307336175, -1.001099928024, -1.292304006338, -1.591630377162, -1.893019701465, -2.201209923647, -2.506660775153, -2.815625046101, -3.122430143612, -3.429364475269, -3.72505055753, -4.023057597177, -4.307076750992, -4.584972354295, -4.851974206402, -5.106148417387, -5.347559415797, -5.576948483823, -5.784839614889, -5.981159965478, -6.156111198496, -6.30959656147, -6.45041515099, -6.55987275788, -6.655793263995, -6.722995668099, -6.76869976497, -6.787490663209, -6.783590665282, -6.752519610718, -6.698564287283, -6.615794148269, -6.511880294189, -6.378281466584, -6.220025813415, -6.041238998862, -5.833121960323, -5.605054062077, -5.350234599383, -5.079590001991, -4.780034515432, -4.468360588381, -4.130322168267, -3.780036472621, -3.411089577322, -3.030185528628, -2.634907020607, -2.231700205315, -1.816117219547, -1.398761938448, -0.967870119262, -0.533948917579, -0.10031802868, 0.342014952778, 0.778997542299, 1.221878289721, 1.653542809478, 2.083595884971, 2.502368388148, 2.912342123176, 3.308199069955, 3.69280778213, 4.05759490835, 4.402173670004, 4.736986818805, 5.045499953056, 5.330420413114, 5.590007684748, 5.831030201483, 6.037340233968, 6.223796171648, 6.375088266782, 6.505817090897, 6.600028268508, 6.67061415748, 6.707615353626, 6.71873505223, 6.697236968676, 6.649148309384, 6.567990662195, 6.460919338063, 6.323744347412, 6.159398755148, 5.970042083259, 5.748390202495, 5.509785072288, 5.239207160015, 4.951933935452, 4.638650733591, 4.311863128522, 3.962482067337, 3.598823090781, 3.219435814265, 2.828187905105, 2.423532267353, 2.013268677874, 1.593787260336, 1.170857241583, 0.745058713974, 0.317455226524, -0.10628069381, -0.536559599228, -0.956170390698, -1.37877891595, -1.790010344895, -2.197890157421, -2.592974779821, -2.979196378686, -3.349786489195, -3.70845164637, -4.045715944667, -4.3717965508, -4.673607650656, -4.956273909006, -5.2199564235, -5.459272535097, -5.679089074392, -5.868286213282, -6.041658005013, -6.18408794079, -6.30775937747, -6.402938419599, -6.474846495158, -6.520550523301, -6.54420832557, -6.539824863307, -6.514362106984, -6.463887844289, -6.3946872037, -6.301667662811, -6.18431355981, -6.054260422905, -5.897584390787, -5.732012684015, -5.54088181332, -5.340758648073, -5.123682130552, -4.894293578911, -4.649466615545, -4.398161494277, -4.134189881976, -3.865738458211, -3.588165975379, -3.308531000887, -3.0243839815, -2.736756297111, -2.452932090653, -2.16456357347, -1.884962022521, -1.602911120461, -1.331432047928, -1.056794509731, -0.793631208497, -0.533046459727, -0.280068224611, -0.036372475961, 0.196300351006, 0.424912084094, 0.636344877161, 0.841073689194, 1.031073107354, 1.206472060374, 1.373845595888, 1.519656861632, 1.659795547723, 1.778468655645, 1.889341962949, 1.981070292399, 2.061356758571, 2.12433538713, 2.176226685399, 2.211293601344, 2.236240102863, 2.244781217885, 2.243040764236, 2.228472522925, 2.201495492363, 2.160498142613, 2.110605143374, 2.055104018764, 1.981038061762, 1.907165492431, 1.816758622552, 1.72515922494, 1.623342728618, 1.517207335446, 1.405012592267, 1.290142712201, 1.168246562564, 1.047156179274, 0.919039523837, 0.792727780462, 0.665803652141, 0.534979615125, 0.407733168748, 0.276586809842, 0.152950173688, 0.024575625662, -0.097675117694, -0.219539107163, -0.33276530288, -0.44750635248, -0.555833520716, -0.659648413935, -0.759434490888, -0.85722228175, -0.945888811272, -1.032557052242, -1.113939476566, -1.187393167446, -1.260202254478, -1.321988459376, -1.383935824916, -1.431895080745, -1.481530336808, -1.52059393143, -1.554532849089, -1.584926392742, -1.610227488406, -1.62624614447, -1.64239372398, -1.647872942625, -1.65280423958, -1.652836470222, -1.645584563108, -1.639911960213, -1.625472607776, -1.610549795346, -1.5874726176, -1.567940817251, -1.540705882338, -1.514212254869, -1.483045179111, -1.452554949714, -1.416521044576, -1.38277552039, -1.345001163501, -1.307291270799, -1.268163230894, -1.23274172125, -1.193581455997, -1.150585744158, -1.117291465704, -1.074875911501, -1.041484945369, -1.003001536946, -0.967515582024, -0.932223013107, -0.898219672272, -0.863507258885, -0.833178215835, -0.799142649494, -0.772745748364, -0.743351398115, -0.716471039411, -0.693587281637, -0.668092842444, -0.650688295345, -0.627256618724, -0.612881752772, -0.595863974652, -0.583519639569, -0.56724316682, -0.556800439871, -0.545551947147, -0.535721602628, -0.528276325388, -0.523796266856, -0.516060913979, -0.514094845139, -0.511065165314, -0.508841251385, -0.512032084435, -0.509002404553, -0.516350989715, -0.514513843417, -0.520831048233, -0.522764886451, -0.526729254832, -0.53195061806, -0.538590129407, -0.541652039967, -0.550966694366, -0.553802990491, -0.563053183779, -0.569853848527, -0.575590902357, -0.584905557093, -0.590932686735, -0.601020877055, -0.60350263635, -0.614944513774, -0.618908882582, -0.629125995866, -0.634927511342, -0.643146325024, -0.647884229412, -0.655651814247, -0.659551722015, -0.665675544213, -0.668963069777, -0.677633112898, -0.681629712678, -0.682854477157, -0.691717904228, -0.692169133285, -0.701097021755, -0.701580481458, -0.70715638295, -0.710379447476, -0.713634742606, -0.714279355512, -0.718340416815], [-0.711765365224, -0.724560931444, -0.722369247503, -0.726784845983, -0.72494769918, -0.728621992799, -0.727880687945, -0.730072371842, -0.730169063782, -0.730845907354, -0.730104602467, -0.732618592899, -0.730749215401, -0.73229628649, -0.731135983188, -0.734230125256, -0.735744965582, -0.730781446088, -0.737066422059, -0.732747515477, -0.736228425243, -0.735197044577, -0.734326817112, -0.734584662293, -0.73342435903, -0.730555831519, -0.730684754112, -0.725270005612, -0.726108002436, -0.721885787838, -0.717824726532, -0.717147883005, -0.710476139452, -0.711249674934, -0.703578781432, -0.702676323345, -0.696004579975, -0.692813746133, -0.684240394829, -0.67934133696, -0.672121672803, -0.663354937875, -0.655812967451, -0.650043682499, -0.638440651315, -0.632123445558, -0.622744328924, -0.611689219083, -0.607595927736, -0.593865674939, -0.589933536879, -0.575333057211, -0.567501011901, -0.558411971797, -0.547131248426, -0.538364514917, -0.530081241095, -0.517382370075, -0.51100070404, -0.498624139668, -0.492371396341, -0.485183964551, -0.476449462421, -0.473194168256, -0.465555507761, -0.464234051759, -0.457014389609, -0.457755694206, -0.454371477587, -0.456530930071, -0.456982158954, -0.458819305118, -0.462396905535, -0.46897195505, -0.47374208902, -0.483926969825, -0.492210243146, -0.508003254901, -0.522893809026, -0.535270373741, -0.558895431386, -0.574559521866, -0.601278722161, -0.624001323916, -0.650913909799, -0.679824796629, -0.710411678102, -0.740547331832, -0.775582045369, -0.808135000648, -0.848326621873, -0.884908412339, -0.925744651385, -0.968127964584, -1.008577441074, -1.056762279125, -1.097276222847, -1.147588292081, -1.191615385176, -1.241476233341, -1.284697567014, -1.33227004555, -1.378778915937, -1.420968878904, -1.465318301289, -1.510505725619, -1.547055328546, -1.589825458321, -1.625085839421, -1.659056995213, -1.6933182298, -1.717781332923, -1.748690578516, -1.765740622068, -1.785755891413, -1.798164714248, -1.806254622338, -1.809703308258, -1.809252078319, -1.799163866215, -1.788269886665, -1.76541831494, -1.743694819196, -1.711302961563, -1.672851734771, -1.630113828191, -1.577964562881, -1.525267381534, -1.456487093395, -1.391864572571, -1.311513489345, -1.230872342166, -1.140529775998, -1.045288163425, -0.943826049219, -0.836916971325, -0.721821326526, -0.606467855284, -0.479189066374, -0.355326744083, -0.223052245422, -0.083783719617, 0.049554354938, 0.196719348996, 0.334666373306, 0.48295941228, 0.627545921343, 0.774259643201, 0.919458521707, 1.065463162938, 1.206891058243, 1.34793218853, 1.481882589672, 1.615349537597, 1.739276232442, 1.860205488455, 1.972754793568, 2.073636624006, 2.174131695086, 2.255288400978, 2.334833581771, 2.396265156012, 2.453506752411, 2.495084265497, 2.524027372682, 2.541045146617, 2.543430213434, 2.529861117134, 2.506655062122, 2.462015638659, 2.408770639614, 2.335897192413, 2.24555475284, 2.146123286002, 2.021197409573, 1.891179107926, 1.737793624341, 1.575093507418, 1.394763259411, 1.202088698055, 0.994652523619, 0.776225710175, 0.544100877349, 0.304208444897, 0.047813901563, -0.211159144441, -0.483798047303, -0.7653326994, -1.052572293041, -1.351124992534, -1.647808481302, -1.959221597519, -2.263576411537, -2.577342854314, -2.887370806551, -3.196786672335, -3.502560771377, -3.804693114694, -4.097801143999, -4.386429416404, -4.661940020556, -4.932841925659, -5.185952608819, -5.425397603927, -5.655914855497, -5.862258976218, -6.060545516593, -6.229662966251, -6.387080614154, -6.520099284844, -6.631684206844, -6.718579969795, -6.784170830334, -6.823106351241, -6.840704694108, -6.828811308327, -6.796128675609, -6.733793179361, -6.64683294574, -6.537890983214, -6.395138442166, -6.238010868241, -6.046911698304, -5.838214491566, -5.598736752886, -5.34024295002, -5.058736491301, -4.756151316888, -4.432584187887, -4.093063195321, -3.731174427893, -3.358005356716, -2.96743213227, -2.568350468634, -2.160405808323, -1.73857013707, -1.318604238285, -0.881105195248, -0.447989812003, -0.002143557587, 0.439770395346, 0.884520545481, 1.326466604942, 1.764770645786, 2.195178290564, 2.620235815048, 3.02843692896, 3.430288857773, 3.814124125672, 4.179072505695, 4.52316791251, 4.853211018603, 5.164689498048, 5.44345397781, 5.704814050875, 5.9364897071, 6.144959296661, 6.322745187771, 6.475552201279, 6.596772938093, 6.691693235321, 6.755704025392, 6.790030060846, 6.791222608696, 6.766114644038, 6.710580606664, 6.62197757689, 6.508234414488, 6.359295095206, 6.193789165152, 5.98938063049, 5.765923803883, 5.515522164724, 5.241753395342, 4.94510100651, 4.628981503492, 4.290397456829, 3.93847018769, 3.564207334467, 3.179985482758, 2.78126008812, 2.368385663559, 1.953803191747, 1.525587293446, 1.098338380085, 0.665416884865, 0.236459696272, -0.197138822371, -0.624291399669, -1.052507831657, -1.472989204735, -1.890312321264, -2.296774081073, -2.696242198286, -3.081722610934, -3.457050786674, -3.813749999477, -4.153560682818, -4.479544743602, -4.778809735956, -5.065569480639, -5.322515831455, -5.562960158558, -5.776523965273, -5.966945991103, -6.133227000213, -6.275431391187, -6.390561595666, -6.484773744206, -6.547657079024, -6.589880141444, -6.607413996422, -6.599259464388, -6.570734721027, -6.512073682302, -6.438199480229, -6.338024566655, -6.220122507215, -6.078304936196, -5.921564420508, -5.743229139087, -5.550132156053, -5.341113190445, -5.117300374375, -4.880176376789, -4.633899033522, -4.373504792794, -4.106825808411, -3.833475315589, -3.551261620261, -3.269950678431, -2.976327836394, -2.691053042014, -2.398881106403, -2.110996091378, -1.823433590916, -1.540995958539, -1.262200556184, -0.990302657263, -0.720725484573, -0.461558909037, -0.206614626238, 0.037919101747, 0.272267907717, 0.499590406638, 0.709766199878, 0.914688392123, 1.100852367279, 1.279925610207, 1.440724104466, 1.590016279132, 1.724740227003, 1.845605020756, 1.949516519928, 2.042534077976, 2.117470265228, 2.181157970384, 2.227731218564, 2.261766756197, 2.283038967805, 2.28664879767, 2.282748892171, 2.259220536969, 2.232630273161, 2.185960332916, 2.134133495452, 2.069672257958, 1.998023596367, 1.916286756241, 1.827588108294, 1.729381434927, 1.628402934234, 1.516723876331, 1.403529984368, 1.285275890746, 1.159995527641, 1.038131609861, 0.904245675988, 0.777353781392, 0.643338918953, 0.515641249901, 0.383495749512, 0.254637762314, 0.12616653192, 0.001015043127, -0.123491846328, -0.242132776215, -0.360709259352, -0.471582636471, -0.580715573951, -0.687463459203, -0.785315701171, -0.884682797774, -0.971737798179, -1.062015877006, -1.138015783997, -1.214273546373, -1.282054651605, -1.345678007751, -1.402500697588, -1.453940869169, -1.497774603487, -1.539384423977, -1.570196965704, -1.599140129151, -1.621701616217, -1.638977270006, -1.65506038846, -1.657896689984, -1.66540644294, -1.659475994245, -1.6561884629, -1.644843256998, -1.631628670883, -1.614481940201, -1.594917908013, -1.569326736977, -1.543928951467, -1.513599871748, -1.483303024612, -1.44929965047, -1.4141037433800001, -1.380390449999, -1.340682252615, -1.307678038826, -1.264521164743, -1.230131036731, -1.189617083625, -1.151584894783, -1.112360173922, -1.07342553161, -1.034780967818, -0.998328091321, -0.959328995068, -0.926228111175, -0.88954962641, -0.857383435016, -0.825056091908, -0.790665988836, -0.767621075384, -0.735583812304, -0.713473589391, -0.685658543145, -0.665159853888, -0.642662865403, -0.622808790165, -0.604050557231, -0.587870775927, -0.571852148146, -0.55921773777, -0.545165179484, -0.536269523486, -0.526535870989, -0.517736907139, -0.515287378725, -0.507165258283, -0.507906562927, -0.501395974404, -0.503748810838, -0.50236289347, -0.504393423551, -0.505682649001, -0.508293330553, -0.510388321916, -0.515867530145, -0.518059213454, -0.524569802165, -0.52875978496, -0.535786063969, -0.544327182925, -0.5475180161, -0.558959892661, -0.561989572689, -0.574462829917, -0.58013542245, -0.588805464462, -0.597636659824, -0.605597627963, -0.612591676972, -0.619392342204, -0.625580625296, -0.63495974198, -0.639891030191, -0.646466081183, -0.654330357939, -0.658165804432, -0.668737455312, -0.669672143973, -0.680662793387, -0.683982549693, -0.691427828421, -0.694360817091, -0.698679723403, -0.703030860409, -0.706511770053, -0.708606761965, -0.712861207147, -0.712990129697, -0.717695803943, -0.718082571675], [-0.71427935551, -0.722143632976, -0.72404524108, -0.724464239483, -0.726011310473, -0.728170763755, -0.726236924985, -0.730974829944, -0.729911218611, -0.734423509066, -0.732006210595, -0.73532596716, -0.734326817122, -0.73645403979, -0.734487970348, -0.737324267224, -0.735809426843, -0.737130883336, -0.735616042946, -0.735841657505, -0.735809426825, -0.734004510669, -0.735325967138, -0.73245743967, -0.733005360631, -0.72833191696, -0.728944299233, -0.724367547531, -0.724883237855, -0.721015560384, -0.718179263577, -0.713151282924, -0.711636442602, -0.704996929745, -0.70048463953, -0.69590788798, -0.690009680114, -0.685787465724, -0.676247195206, -0.67276628568, -0.662742555697, -0.659003801098, -0.648496611662, -0.643371939515, -0.635346509704, -0.629125995852, -0.617587426319, -0.609626458033, -0.598313503252, -0.590062459426, -0.5810056497, -0.569982771092, -0.560764808435, -0.550934463727, -0.54278011233, -0.530435778128, -0.525568951902, -0.515126225547, -0.509163557759, -0.49820514143, -0.491275554701, -0.483862508508, -0.476868460633, -0.470647948067, -0.466232351115, -0.461107680184, -0.458625921328, -0.455628472316, -0.453501250461, -0.455789625498, -0.455499549774, -0.462267983033, -0.463879514753, -0.471679328402, -0.477351920158, -0.487569031621, -0.495787843706, -0.511451932955, -0.524118573203, -0.541361964245, -0.557606205819, -0.579490809668, -0.601020877026, -0.62522608831, -0.651203985583, -0.68021156439, -0.710701753907, -0.739967180224, -0.77648450352, -0.809585379893, -0.849261310757, -0.886810020881, -0.928903255565, -0.969288268192, -1.013669885247, -1.056182127116, -1.102239745154, -1.14662137207, -1.194193838741, -1.239993622437, -1.283891800131, -1.333108043207, -1.377167381948, -1.425126637116, -1.467606680147, -1.512761873853, -1.55398492737, -1.595369137754, -1.630146058852, -1.665793211348, -1.697089221818, -1.725935700923, -1.7511078814, -1.771961148467, -1.789784729985, -1.802322475745, -1.811443766655, -1.812088380825, -1.814022223456, -1.80486870181, -1.794780489812, -1.772154532753, -1.749109577661, -1.716040874956, -1.677847493227, -1.632305515562, -1.582380167971, -1.52243108076, -1.459226701699, -1.386159741905, -1.308967265931, -1.22658566283, -1.13463156401, -1.040292410915, -0.936348537068, -0.829181615174, -0.712764515191, -0.595606129522, -0.467747190914, -0.342724567549, -0.20651793436, -0.070891470967, 0.071600097559, 0.213414807264, 0.359129407496, 0.506584448778, 0.654297325408, 0.800882123762, 0.94737022586, 1.096952464068, 1.236027525487, 1.379518182597, 1.512469436124, 1.645259542865, 1.769379623202, 1.890341111973, 2.001085504894, 2.107930002, 2.202365719158, 2.290387550084, 2.363937837082, 2.429043704874, 2.484931616791, 2.523350529433, 2.553260556559, 2.564992507132, 2.567732111023, 2.551584563608, 2.522383610465, 2.476454960925, 2.420470357663, 2.343825926324, 2.255417323432, 2.149281886744, 2.02712784304, 1.88930973233, 1.737761393734, 1.570162224343, 1.387124605696, 1.192451747079, 0.979407447398, 0.758434415577, 0.519895690267, 0.278069418051, 0.018709653029, -0.244840148886, -0.519219516403, -0.800979796488, -1.094955614997, -1.389286118006, -1.694833072763, -2.000702537671, -2.312986148011, -2.625850171815, -2.93652278559, -3.249355170025, -3.556031789992, -3.859840201111, -4.153141680389, -4.444058420266, -4.719923636027, -4.989923143988, -5.243775212777, -5.485573151627, -5.709837625206, -5.920081784168, -6.110826273553, -6.282651200402, -6.433461476219, -6.566415720895, -6.675067619843, -6.758450185193, -6.824588995507, -6.859173286962, -6.875772460093, -6.859624526589, -6.824137755937, -6.759191506871, -6.670909773554, -6.553490951991, -6.413091283668, -6.242394322554, -6.052036466714, -5.835281451458, -5.593354147693, -5.330863692688, -5.043555652639, -4.739294486152, -4.410602654685, -4.067600751817, -3.704519477413, -3.328385203867, -2.933009627492, -2.530962774319, -2.115669547686, -1.693124845495, -1.263489783148, -0.828827078002, -0.386300380611, 0.058256621803, 0.505617530523, 0.952494892089, 1.394537645167, 1.835839145116, 2.264699742945, 2.692754748947, 3.102277361797, 3.50377480462, 3.887610130214, 4.256039492337, 4.596750738449, 4.933014458055, 5.236660924787, 5.523160877875, 5.777881462885, 6.010846419604, 6.2183169114, 6.393878919235, 6.543752959125, 6.662072941399, 6.755220560184, 6.813171935692, 6.845145114857, 6.842824480732, 6.813043011561, 6.751642917357, 6.662395251416, 6.541206711077, 6.393330992815, 6.217124366535, 6.015197593409, 5.783360713855, 5.527576505504, 5.25171272113, 4.94664808477, 4.627563349858, 4.28085715874, 3.924030829939, 3.544707770738, 3.153072880645, 2.747514606141, 2.33567157803, 1.91096870489, 1.484364346433, 1.050250317358, 0.616329669921, 0.182570109135, -0.253639110055, -0.683982549674, -1.11674354445, -1.538546426072, -1.960156288454, -2.37003457972, -2.77282255144, -3.157593978725, -3.533856947913, -3.889943875657, -4.232300908653, -4.554030586337, -4.856518784492, -5.137799349038, -5.398001136619, -5.634513353977, -5.846497912768, -6.037081168104, -6.199268870824, -6.342891493272, -6.452542418278, -6.544337250969, -6.604609868697, -6.644834601269, -6.655342024898, -6.646123855617, -6.609670191078, -6.552620705694, -6.468625849124, -6.367838522832, -6.242458785089, -6.09641890151, -5.935520541452, -5.752995191112, -5.558125484081, -5.340597492477, -5.116043361895, -4.87360124189, -4.623746263204, -4.360483476925, -4.091000415003, -3.811332681458, -3.529409087399, -3.23955699438, -2.947416799028, -2.655115719545, -2.362782659945, -2.072834905165, -1.782017129298, -1.498902677582, -1.216852000067, -0.94714580684, -0.674474509818, -0.416436021814, -0.161008292115, 0.081430435869, 0.318454375505, 0.544294261008, 0.759046797099, 0.958908782521, 1.150551960331, 1.3256930704, 1.486878333803, 1.635815974349, 1.76644663758, 1.890308881358, 1.990932860833, 2.080437284391, 2.153504097989, 2.215451351557, 2.258769308244, 2.293352767506, 2.308662314137, 2.315462975972, 2.305793788522, 2.284328192747, 2.252226491756, 2.205878856903, 2.151119032095, 2.086722254951, 2.012656296172, 1.924892330287, 1.837353983908, 1.733055724553, 1.631819378809, 1.517948639422, 1.40256306617, 1.282407366842, 1.158480689198, 1.028752503791, 0.90166722756, 0.766975526221, 0.637891946316, 0.507035677319, 0.372086113208, 0.24358266189, 0.112178444411, -0.013037507026, -0.137544398039, -0.257474554668, -0.376889036173, -0.487536800959, -0.600956415756, -0.703159783003, -0.806040008442, -0.902216273391, -0.990496041248, -1.076519675291, -1.157612029636, -1.230034344694, -1.299201370965, -1.362437961015, -1.417391273061, -1.472054514814, -1.511633799747, -1.553630389705, -1.586860234387, -1.614417478835, -1.637397965769, -1.654061236775, -1.663472600955, -1.673560810025, -1.673045118824, -1.670337740007, -1.664310599148, -1.651837318588, -1.640621035564, -1.618220700996, -1.597947593358, -1.574483647939, -1.548860247294, -1.515694866593, -1.488202089125, -1.451394645029, -1.4187771924249999, -1.379552452264, -1.342003710407, -1.304745047244, -1.26558477698, -1.224361746464, -1.185652711274, -1.144719762673, -1.105301658294, -1.069815697357, -1.028044759736, -0.99458933488, -0.955622469533, -0.920974514364, -0.885778639949, -0.851807532229, -0.818900037683, -0.789795761301, -0.758145264994, -0.731458289609, -0.704674623302, -0.678825646667, -0.658520341464, -0.634411821073, -0.617297350552, -0.598152350062, -0.584067560455, -0.566953091032, -0.556284749658, -0.54139419487, -0.533626611202, -0.523312807272, -0.517317908815, -0.510646167026, -0.506133877904, -0.501943895193, -0.500235671484, -0.499494366853, -0.498591909034, -0.50139597438, -0.500976976118, -0.506456184285, -0.50623056982, -0.513804769405, -0.516931141161, -0.524021881292, -0.529114321967, -0.535786063895, -0.540975196562, -0.549806391361, -0.55557567561, -0.562118495244, -0.571110843455, -0.578523890504, -0.588128621042, -0.591673991433, -0.603309252486, -0.608208309861, -0.619456803495, -0.623614556202, -0.634895280692, -0.639504262485, -0.648754456759, -0.653363438624, -0.659712875235, -0.664805316804, -0.671477059967, -0.676956269335, -0.68040494819, -0.686593231814, -0.690654292999, -0.697777265362, -0.699163183093, -0.706028310381, -0.708445608764, -0.714053740998, -0.714376047447, -0.717309036158, -0.71921064424], [-0.710024910386, -0.716793345845, -0.719113952322, -0.719951949094, -0.719790795876, -0.722401478154, -0.721176713661, -0.722304786221, -0.722079171739, -0.725366697573, -0.723755165329, -0.727171613748, -0.725914618561, -0.729556681513, -0.729653373454, -0.733424359014, -0.730878137988, -0.732457439676, -0.733649973565, -0.732876438082, -0.73352105098, -0.731683904154, -0.733230975168, -0.731554981578, -0.731232675104, -0.729621142786, -0.729878987971, -0.727171613711, -0.728202994377, -0.722240324934, -0.722111402363, -0.716471039402, -0.713538050689, -0.709219144247, -0.704191163629, -0.700291255632, -0.695811196034, -0.689042760769, -0.681533020716, -0.677826496737, -0.670155603587, -0.663999550742, -0.655007201422, -0.648077613287, -0.636410120856, -0.629448302266, -0.617232889248, -0.61023884021, -0.598990346709, -0.591126070533, -0.580328806276, -0.569015851931, -0.560635885853, -0.550225389661, -0.54010496934, -0.529082091324, -0.5206376644, -0.509904862377, -0.501331513109, -0.490469788818, -0.485377348365, -0.475321390163, -0.471195868845, -0.464266282357, -0.459753993514, -0.455177243418, -0.45137402858, -0.450632723992, -0.448312118361, -0.44860219404, -0.449698035625, -0.454371477572, -0.456917697711, -0.464653049979, -0.471131407592, -0.483282357051, -0.492693702657, -0.508035485456, -0.522088043056, -0.539911585558, -0.558025204138, -0.578266045382, -0.601858873674, -0.626483083273, -0.654362588553, -0.681565251366, -0.71224882486, -0.744092702944, -0.780448873256, -0.816418277644, -0.855481826546, -0.892966075707, -0.936284075784, -0.975573246475, -1.019503634723, -1.062531567617, -1.107880111461, -1.154646808241, -1.200317665994, -1.247277754457, -1.292368467699, -1.34100455941, -1.386707663505, -1.432475233028, -1.474568508417, -1.519852625568, -1.559464144987, -1.598946744905, -1.634271588084, -1.669725356739, -1.700763521852, -1.729900077529, -1.753138415857, -1.775119757793, -1.792524340144, -1.80361170409, -1.81241068786, -1.814731299025, -1.812475149306, -1.804320779705, -1.791235111838, -1.769543845466, -1.745403046532, -1.71143188441, -1.674688884542, -1.627180834679, -1.577126564795, -1.518047706938, -1.453070640671, -1.38135737042, -1.30219882384, -1.218366841609, -1.127992046752, -1.030462059294, -0.926485956427, -0.819544650698, -0.701709403981, -0.584067560439, -0.458142461785, -0.329703393025, -0.19533390736, -0.059546292283, 0.082784121787, 0.226564897832, 0.371989421375, 0.519605614793, 0.666512725505, 0.816094969741, 0.962421918486, 1.109973628512, 1.251949444581, 1.393183959693, 1.527488899303, 1.660311237483, 1.784528010615, 1.906166343397, 2.016201663976, 2.121337939531, 2.217481880751, 2.303376491683, 2.379182923551, 2.442870644673, 2.496792488978, 2.535984937287, 2.564380125067, 2.57672445783, 2.578207067045, 2.561189292331, 2.532246183905, 2.485157231178, 2.427528865298, 2.350014206541, 2.259156075714, 2.150990109623, 2.029126141282, 1.8904055732, 1.734570563254, 1.566971394115, 1.382322245342, 1.184426326374, 0.970608492196, 0.747250395204, 0.509066205683, 0.264049101386, 0.004528180618, -0.260375311122, -0.538171131096, -0.820576031503, -1.115260933764, -1.414200435406, -1.71903833033, -2.028453192339, -2.340478978614, -2.655502488952, -2.968205671777, -3.281134781401, -3.587940359215, -3.891748806981, -4.186242869138, -4.475709255059, -4.752992675415, -5.02395915739, -5.276296406007, -5.519641480332, -5.744002687703, -5.952603092839, -6.14325092322, -6.315011419137, -6.465531641869, -6.595907403787, -6.7039791576, -6.785750168332, -6.847183205524, -6.8814774191, -6.895981552919, -6.878512129785, -6.840446842986, -6.77298653917, -6.683028767301, -6.562547959387, -6.417603667947, -6.247873640808, -6.051714154371, -5.832767417038, -5.588068236284, -5.322451369195, -5.03250039276, -4.723984745866, -4.39335907776, -4.046972951256, -3.68041076967, -3.302245985531, -2.904259747987, -2.499151006579, -2.082471893594, -1.657896690003, -1.226972430874, -0.788248690179, -0.34659224316, 0.101574571531, 0.549128852274, 0.99794004534, 1.440691873864, 1.883089223901, 2.315688590355, 2.742357703593, 3.153814185862, 3.556665354349, 3.938824725544, 4.307802055414, 4.648771194708, 4.982230886135, 5.286554247973, 5.568638621824, 5.826260029219, 6.055357318603, 6.260217140354, 6.435875871716, 6.582752456123, 6.700492300534, 6.79202838416, 6.848400448848, 6.877279453822, 6.870994402281, 6.840890618981, 6.775010405327, 6.682636322387, 6.559062678139, 6.407061384714, 6.228050656109, 6.020709080125, 5.788163116111, 5.529671511214, 5.249134254804, 4.943296081938, 4.619827965986, 4.270704476852, 3.909623703226, 3.527496586161, 3.134572481773, 2.724792004513, 2.311595300989, 1.885699903608, 1.453745269663, 1.018728785616, 0.581842919588, 0.146955279198, -0.290897715685, -0.723207244305, -1.155549266911, -1.581928938196, -2.002571919715, -2.413965101174, -2.817139893542, -3.202717146175, -3.57859340424, -3.93616301468, -4.277714337744, -4.599701926599, -4.90177118411, -5.183180734068, -5.440900782798, -5.678218832441, -5.889429891994, -6.078433861212, -6.241459615534, -6.379570719093, -6.490027451168, -6.577728923312, -6.635326350273, -6.672746961474, -6.681320504889, -6.670265146349, -6.631200736434, -6.571862818298, -6.486739855383, -6.380505427068, -6.254932292263, -6.10769984155, -5.942031249561, -5.758281107182, -5.558351102183, -5.339018167199, -5.109693837164, -4.865027781983, -4.613367876412, -4.346785311362, -4.07462709678, -3.794346993999, -3.510038333336, -3.217672254619, -2.925467618447, -2.630136865355, -2.335579904363, -2.043440480452, -1.75117234287, -1.467348834592, -1.185137020595, -0.912046622996, -0.642050483247, -0.38243270481, -0.12684383114, 0.114821354973, 0.354552660666, 0.579490085203, 0.792888933492, 0.993685605466, 1.181880108564, 1.358729441583, 1.517690794561, 1.66604828599, 1.79745248593, 1.91548099088, 2.016201663979, 2.103965635885, 2.175485381126, 2.236465717242, 2.279106831693, 2.310370537258, 2.325615622902, 2.329870065433, 2.319749649111, 2.297059289292, 2.261508911229, 2.215483582179, 2.159885760796, 2.090622159789, 2.014847978107, 1.928631081568, 1.837128369633, 1.73650439991, 1.632560682816, 1.518238714889, 1.402144068285, 1.277379392366, 1.154741939, 1.024562525132, 0.895253337089, 0.763333467718, 0.630382214794, 0.498140029227, 0.366220141981, 0.235944006455, 0.106634778363, -0.017582024409, -0.142443452805, -0.262051303755, -0.38333516252, -0.494305234496, -0.607112468088, -0.710218294224, -0.814581130586, -0.906986410225, -0.997683478167, -1.082933577324, -1.162446629846, -1.237157323255, -1.303036821458, -1.367562639148, -1.422934950654, -1.475503198335, -1.519562549385, -1.56052775785, -1.593177450511, -1.624086687772, -1.641459033707, -1.659766070563, -1.670950123395, -1.677976416022, -1.679749104576, -1.675945881909, -1.670273278632, -1.657606613718, -1.643715182568, -1.624344533351, -1.60468380868, -1.580091788639, -1.554403926346, -1.522463311488, -1.491167312477, -1.45545571143, -1.420968878936, -1.38248544425, -1.345903622526, -1.305615275514, -1.267679770787, -1.227520352303, -1.186426247372, -1.148136213419, -1.10778341951, -1.068171933565, -1.029688523456, -0.991205115721, -0.951239100204, -0.917203527712, -0.879010202787, -0.848133237989, -0.812679522248, -0.784026475241, -0.752343748533, -0.724947699177, -0.697519420203, -0.672411748598, -0.648980071258, -0.626805389693, -0.606790161664, -0.585743553728, -0.570885229008, -0.554640987151, -0.544262721671, -0.530758084501, -0.52411857322, -0.513837000056, -0.510388321919, -0.501105898678, -0.497657220622, -0.495175461647, -0.492758163962, -0.492790394595, -0.491340015991, -0.494530848929, -0.496110150111, -0.500461285963, -0.503974425287, -0.511032934651, -0.516125375253, -0.524537571479, -0.527309406293, -0.536205062214, -0.543360263805, -0.551353462011, -0.558379741184, -0.565631634866, -0.574204984823, -0.582230413998, -0.589450077279, -0.597894504944, -0.608272771146, -0.615846971723, -0.625032704438, -0.63031852964, -0.638956341598, -0.642888479894, -0.652074212929, -0.65616750453, -0.664354087814, -0.669253145555, -0.676279425834, -0.680243794981, -0.684788315789, -0.691041060696, -0.694844276739, -0.698196263731, -0.702128402385, -0.704610162007, -0.704384547489, -0.707962149067, -0.709509220038, -0.7142471249, -0.713699203924]]
  in  "Open":bool
  in  "Filter lf":bool caption="Scan"
  in  "Low cutoff freq: fl":dbl=40.0
  in  "Tab Control":T7(tab)=enum."          DAQ        "
  out "No. data scan":i32=140
  out "No. X":i32=19
  out "No. Y":i32=7
  in  "Motor counter Y":tag="Dev1/ctr1"
  in  "Motor Counter Y":tag="/Dev1/PFI10"
  in  "Motor Counter X":tag="/Dev1/PFI8"
  in  "Motor counter X":tag="Dev1/ctr0"
  out "Motor Pulses Y":u32=35
  out "Motor Pulses X":i32=700
  out "PLC Connceted":bool=TRUE
  in  "COM":refnum<visa-resource-name>="COM12"
  in  "Encoder":bool=TRUE
  out "Completed":bool
  in  "X Auto Distance":u16=20
  in  "Y Auto Distance":i16=20
  out "Get data":bool
  in  "X Step":dbl=1.0
  in  "Y Step":dbl=1.0
  out "Get data Count":u32=140
  in  "DAQ Pulser":bool=TRUE
  in  "No. Samples":dbl=500.0
  out "Sample per Channel AO":dbl=40000.0
  in  "Pulser Cycles":i32=5
  out "Actual Sample Rate":dbl=25000.0 format="%0.2f"
  in  "Sensor Physical Channel":tag="Dev1/ai1:3"
  in  "Min Voltage":dbl=-10.0
  in  "Max Voltage":dbl=10.0
  in  "Terminal Configuration":i32(ring)=10083 items=["default"=-1, "RSE"=10083, "NRSE"=10078, "Differential"=10106, "Pseudodifferential"=12529]
  in  "Sample Clock Source 2":tag="OnboardClock"
  in  "Sample Rate (Hz)":dbl=25000.0
  out "Actual Sample Rate 2":dbl=400000.0 format="%0.2f"
  in  "Physical Channel(s)":tag="Dev1/ao0:1"
  in  "Min Voltage 2":dbl=-10.0
  in  "Max Voltage 2":dbl=10.0
  in  "Sample Clock Source":tag="OnboardClock"
  in  "Sample Rate 2":dbl=400000.0 format="%#_6p"
  # "Process(Hall)"
  # "Pulse Shape"
  # "Trigger Settings"
  # "Data Processing"
  # "Time gate = %T/2"
  # "3D Surface"
  # "Process(coil)"
  # "Repair line"
  # "Single Hall (0)"
  # "Feature Differential Hall (2)"
  # "PSD Single Hall (0)"
  # "PSD Differential Hall (2)"
  # "Single Hall (0)"
  # "Differential Hall (2)"
  # "Step > S*P/f"
  # "Pulser Channel"
  # "Pulser Timming"
  # "Sensor Channel"
  # "DAQ Timming"
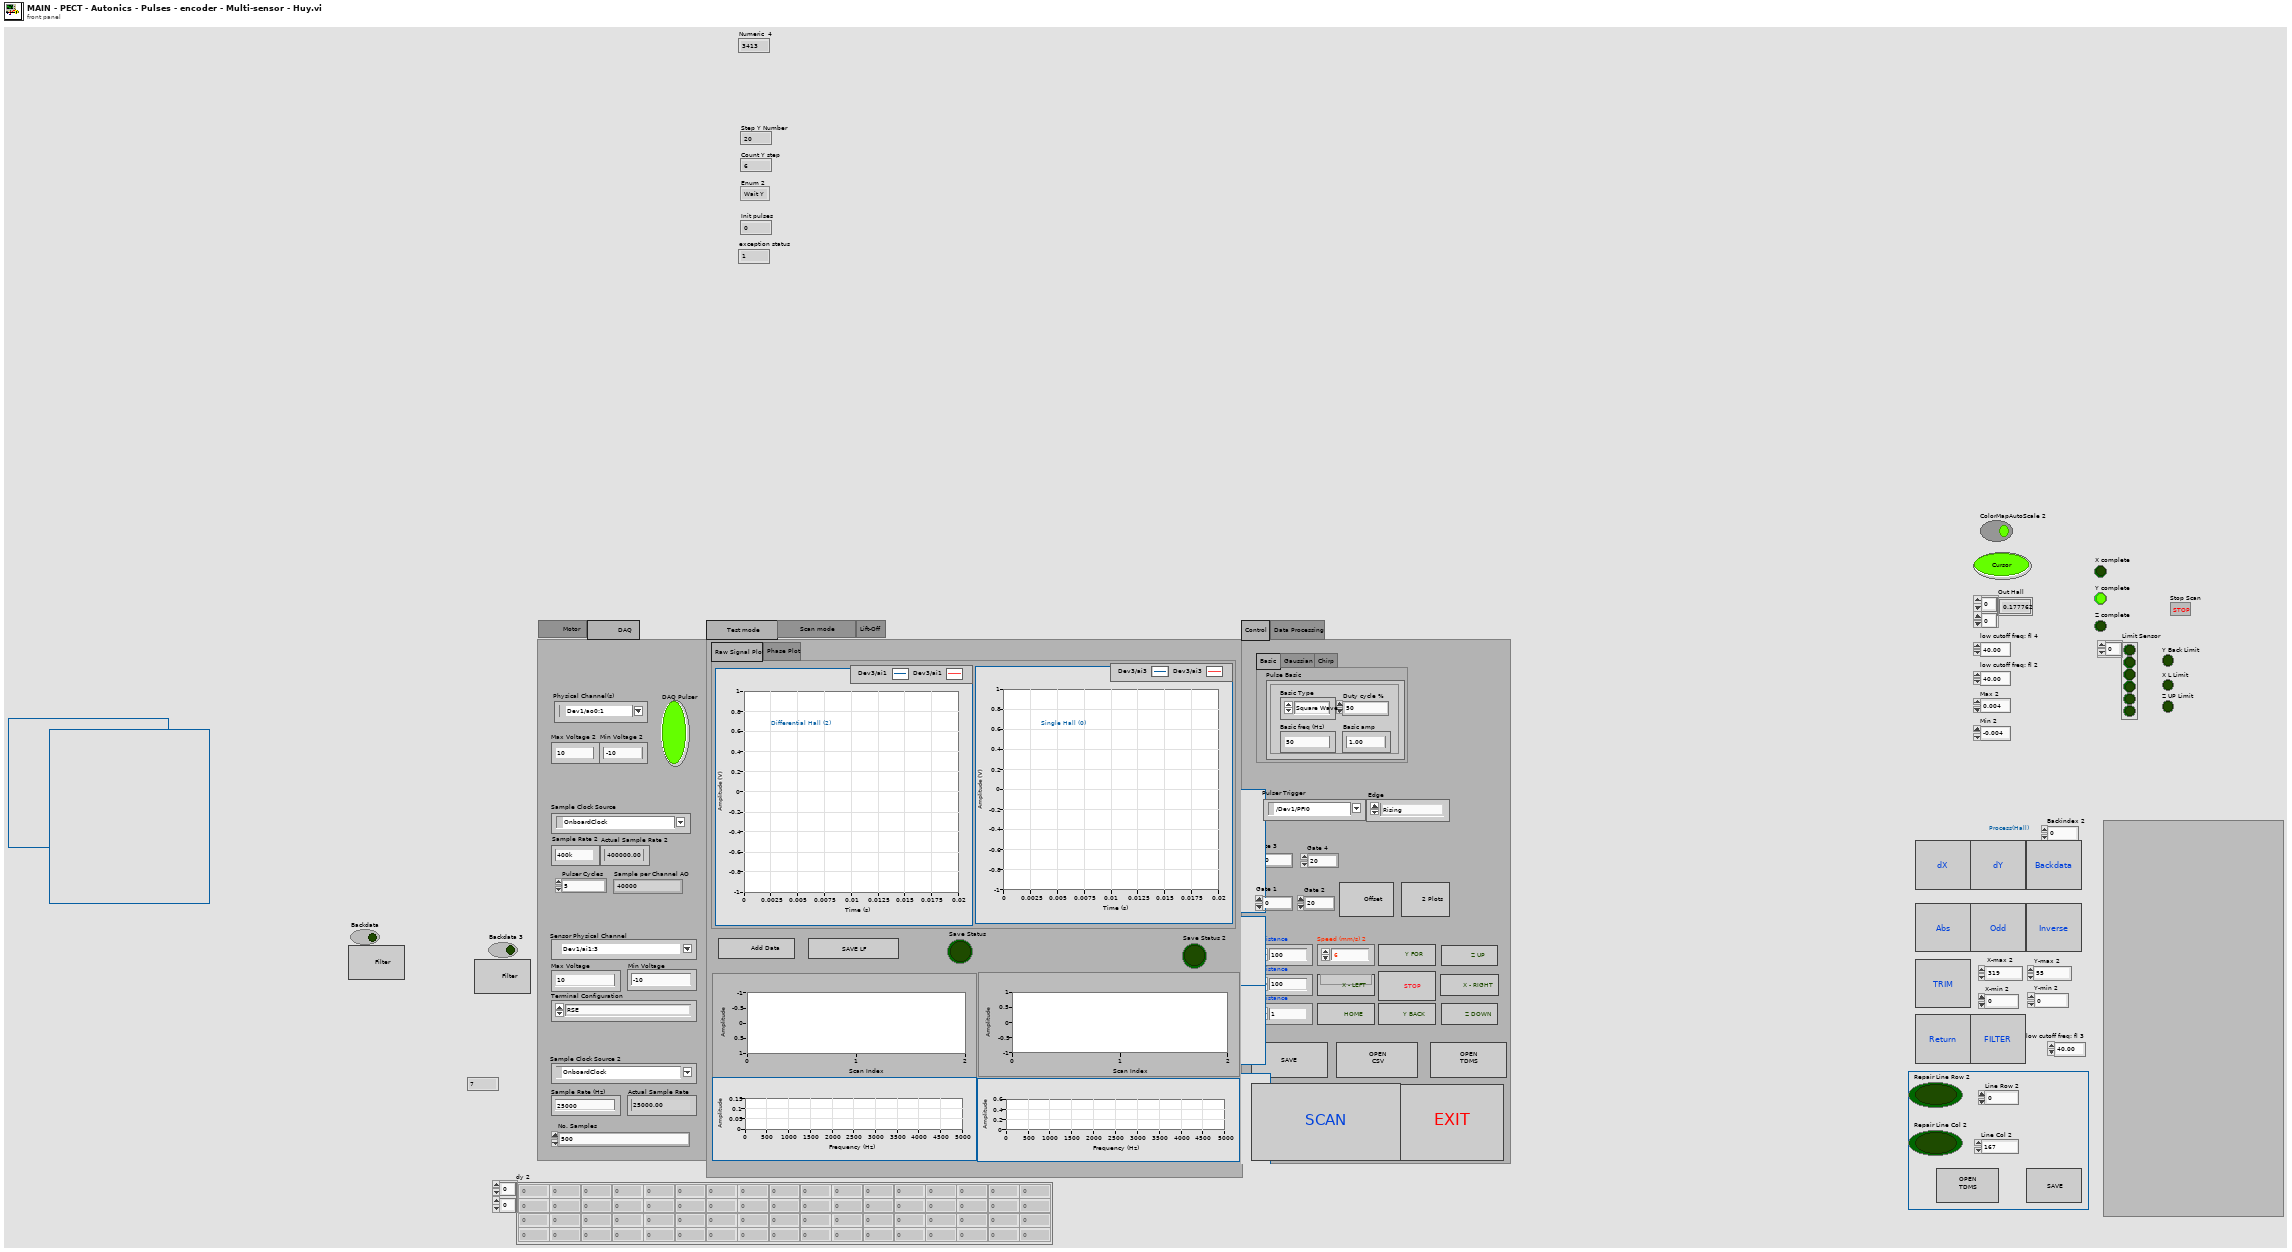
[diagram p1: front panel]
types:
  T1 = enum16{"No Scan", "Move X", "Wait X", "Move Y", "Wait Y"}
  T2 = typedef "Control 1.ctl" = dbl
  T3 = cluster{"Basic amp":T2, "Duty cycle %":dbl, "Basic freq (Hz)":u16, "Basic Type":u16}
  T4 = cluster{"Gauss amp":dbl, "Gauss Nor. Band":dbl, "Gauss atten (dB)":dbl, "Gauss freq (Hz)":dbl}
  T5 = cluster{"Chirp amp":dbl, "Chirp f2":dbl, "Chirp f1":dbl}
  T6 = enum32{"Test mode                   ", "Scan mode                      ", "Lift-Off"}
  T7 = enum32{"        Motor      ", "          DAQ        "}
  T8 = enum16{"open", "open or create", "create or replace", "create", "open (read-only)"}
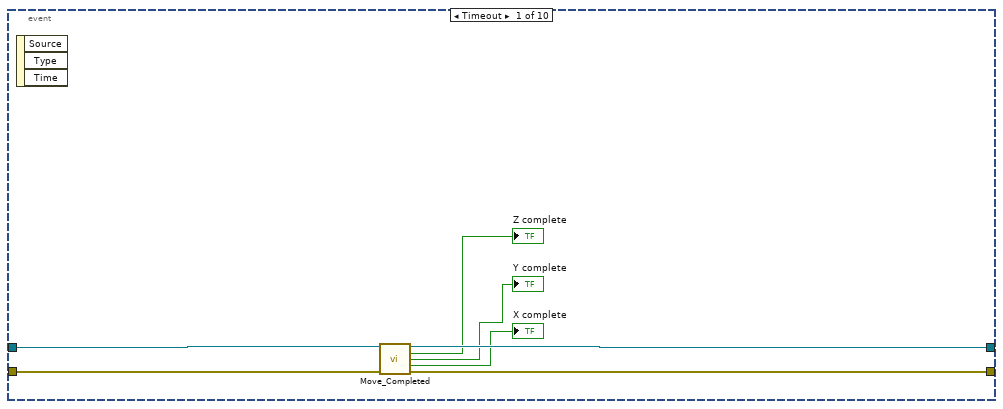
[diagram p2: hidden frame]
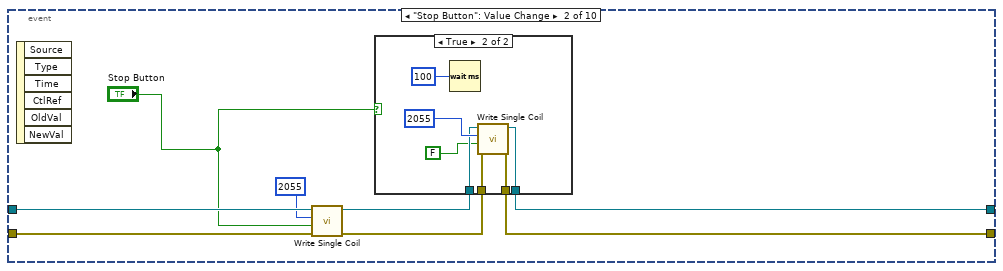
[diagram p3: hidden frame]
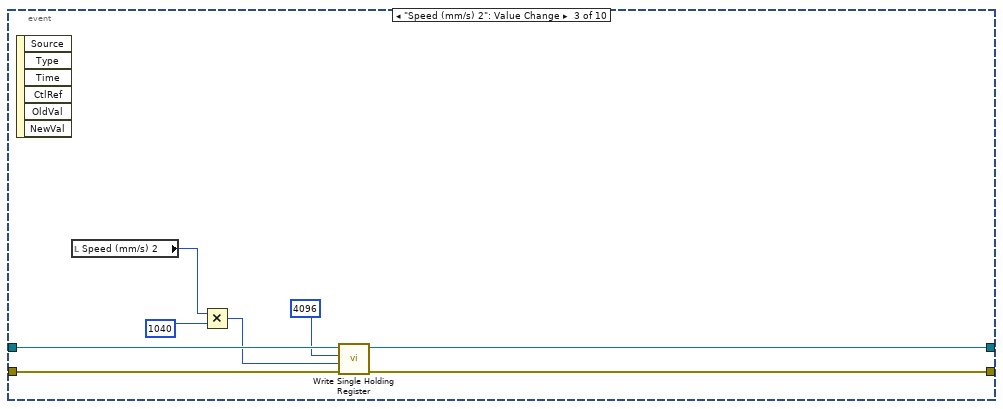
[diagram p5: hidden frame]
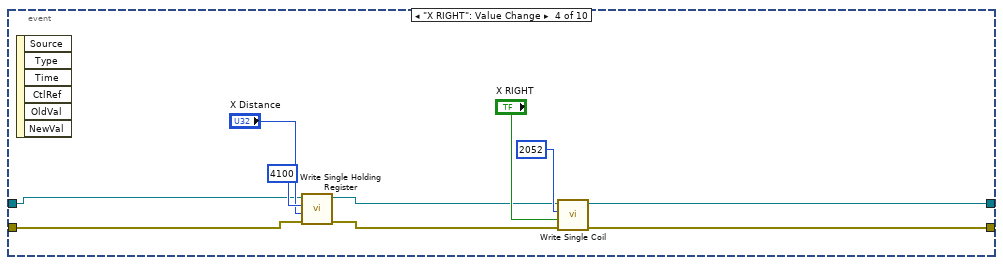
[diagram p6: hidden frame]
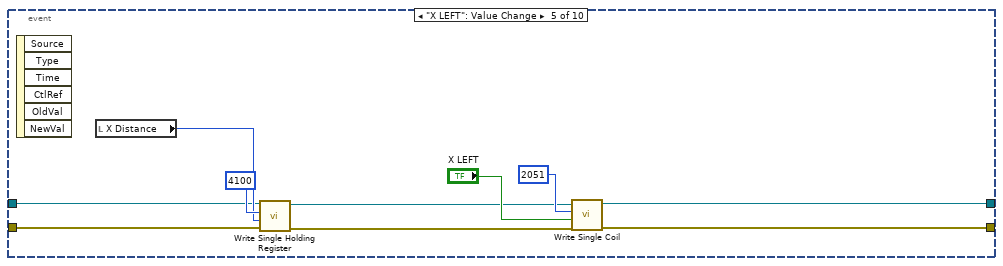
[diagram p7: hidden frame]
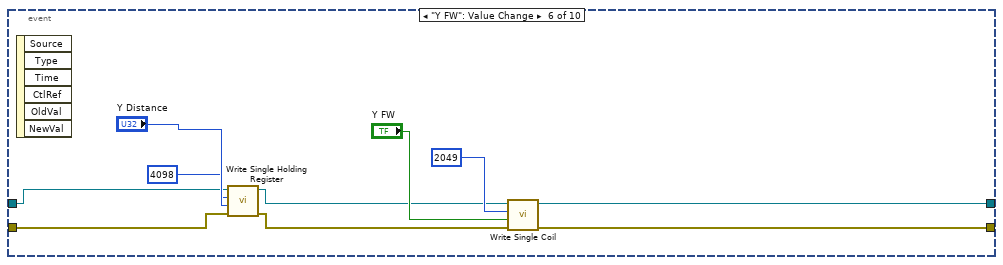
[diagram p8: hidden frame]
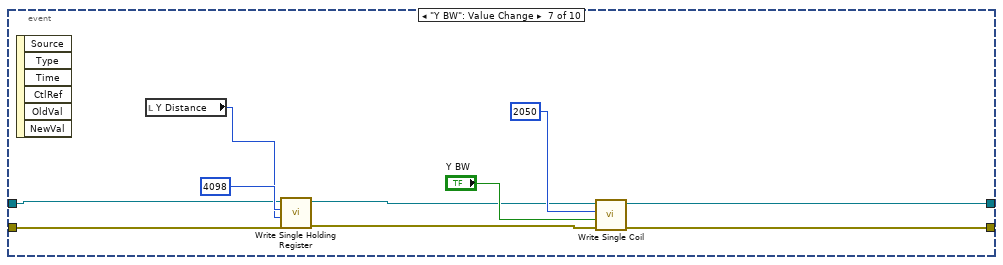
[diagram p9: hidden frame]
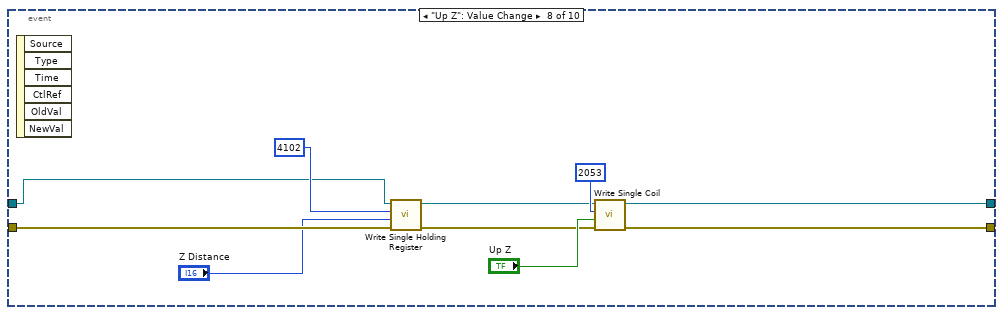
[diagram p10: hidden frame]
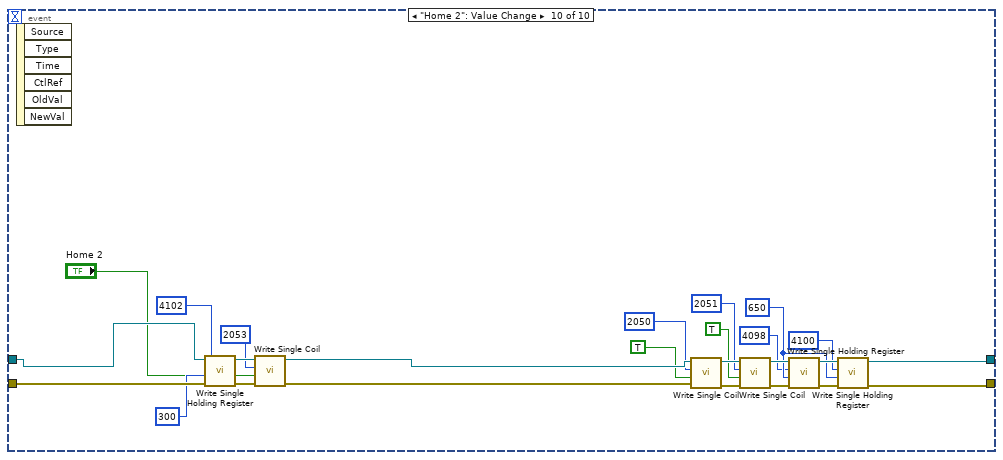
[diagram p11: hidden frame]
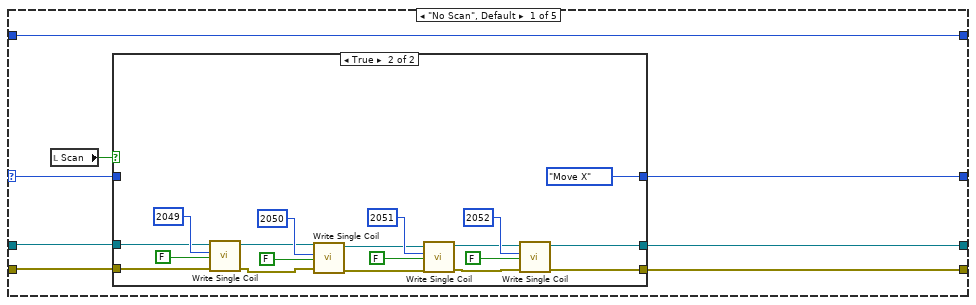
[diagram p16: hidden frame]
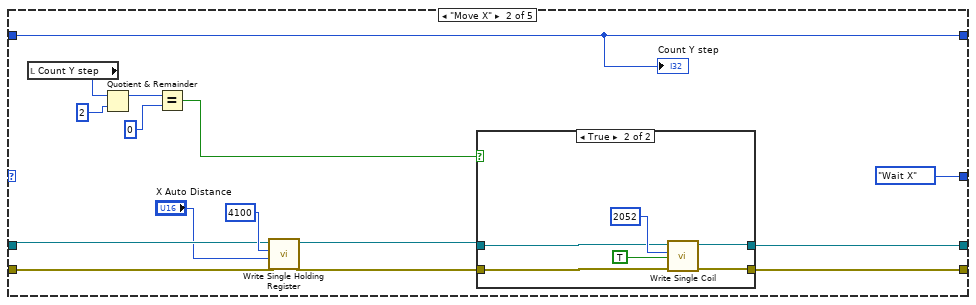
[diagram p18: hidden frame]
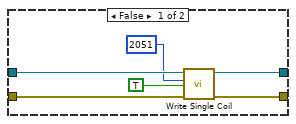
[diagram p19: hidden frame]
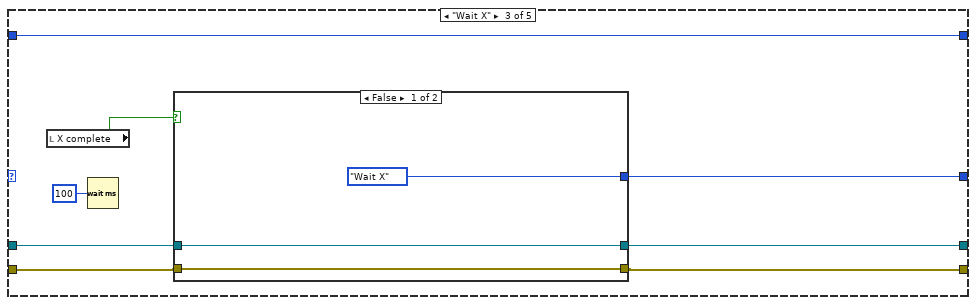
[diagram p20: hidden frame]
diagram:
  w18 = u16 0 items=["None", "XON/XOFF", "RTS/CTS", "XON/XOFF & RTS/CTS", "DTR/DSR", "XON/XOFF & DTR/DSR"] ("flow control (none)")
  w17 = u16 2 items=["None", "Odd", "Even", "Mark", "Space"] ("parity (even)")
  w90 = 10123 items=["Finite Samples"=10178, "Continuous Samples"=10123, "Hardware Timed Single Point"=12522]  # Sample Mode
  # "Count Y step"
  # "1/2"
  # "start1"
  # "start2"
  # "Length"
  n1 = flat-sequence {
    tunnel: [w155] -> w74
    tunnel: [w149] -> w48
    frame #0 {
      w103 = FALSE ("Exit")
      n2 = local write "Scan"(w103) -> ()
      n3 = local write "Exit"(w103) -> ()
    }
    frame #1 {
      n4 = disable-structure shown="Enabled" {
        frame Enabled {
          n5 = flat-sequence {
            tunnel: [w116] -> w108
            tunnel: [w115] -> w106
            tunnel: [w114] -> w105
            tunnel: w104 -> [_]
            frame #0 {
              n6 = call "File Dialog2"("prompt"="Choose New File For Recording\n" ("button label"), "default name"="PECT2_default", "pattern (all files)"="*.tdms") -> ("selected path"=w116:path, "exists"=w115:bool, "cancelled"=w114:bool)  [unwired: 9 in, 1 out]
            }
          }
          n7 = call "File Dialog"("prompt"="Choose New File For Recording\n" ("button label"), "default name"="PECT_default", "pattern (all files)"="*.tdms") -> ("selected path"=w113:path, "exists"=w107:bool, "cancelled"=w109:bool)  [unwired: 9 in, 1 out]
          n8 = case shown="False" w109 {
            tunnel: w113 -> [w135 _]
            tunnel: w107 -> [w136 _]
            tunnel: [w134 _] -> w104
            frame False {
              n9 = case shown="False" w136 {
                tunnel: w135 -> [w137 w139]
                tunnel: [_ w138] -> w134
                frame False {
                  n10 = local write "Record path"(w137) -> ()
                }
                frame True {
                  n11 = Two Button Dialog(message="Existing File\nDo you want to Replace?", 1:"No" ("F button name (\"Cancel\")"), 2:"Replace" ("T button name (\"OK\")")) -> (T button?=w140:bool)
                  n12 = case shown="False" w140 {
                    tunnel: w139 -> [_ w147]
                    tunnel: [path "" ("deleted path") w146] -> w138
                    frame False {
                      n13 = local write "Exit"(TRUE ("Exit")) -> ()
                    }
                    frame True {
                      n14 = Delete(path (use dialog)=w147) -> (deleted path=w146:path)  [unwired: 4 in, 2 out]
                    }
                  }
                  "Record path" <- w138
                }
              }
            }
            frame True {
              n15 = local write "Exit"(TRUE ("Exit")) -> ()
            }
          }
          n16 = case shown="False" w105 {
            tunnel: w108 -> [w121 _]
            tunnel: w106 -> [w120 _]
            frame False {
              n17 = case shown="True" w120 {
                tunnel: w121 -> [w122 w125]
                frame False {
                  n18 = local write "Record path 2"(w122) -> ()
                }
                frame True {
                  n19 = Two Button Dialog(message="Existing File\nDo you want to Replace?", 1:"No" ("F button name (\"Cancel\")"), 2:"Replace" ("T button name (\"OK\")")) -> (T button?=w123:bool)
                  n20 = case shown="False" w123 {
                    tunnel: w125 -> [_ w132]
                    tunnel: [path "" ("deleted path") w131] -> w124
                    frame False {
                      n21 = local write "Exit"(TRUE ("Exit")) -> ()
                    }
                    frame True {
                      n22 = Delete(path (use dialog)=w132) -> (deleted path=w131:path)  [unwired: 4 in, 2 out]
                    }
                  }
                  "Record path 2" <- w124
                }
              }
            }
            frame True {
              n23 = local write "Exit"(TRUE ("Exit")) -> ()
            }
          }
        }
        frame Disabled {
        }
      }
    }
    frame #2 {
      n24 = local read "Record path"() -> (w154:path)
      n25 = local read "Record path 2"() -> (w151:path)
      n26 = local write "Completed"(FALSE ("Completed")) -> ()
      n27 = TDMS Open(6:FALSE ("disable buffering (T)"), 10:T8."create or replace" ("operation"), 11:w151) -> (3:w149:refnum<k34>)  [unwired: 4 in, 1 out]
      n28 = TDMS Open(6:FALSE ("disable buffering (T)"), 10:T8."create or replace" ("operation"), 11:w154) -> (3:w155:refnum<k34>)  [unwired: 4 in, 1 out]
    }
  }
  n29 = local read "DAQ Pulser"() -> (w51:bool)
  n30 = call-poly <vilib>:"DAQmx Create Virtual Channel.vi"("maximum value"="Max Voltage", "minimum value"="Min Voltage", "input terminal configuration"="Terminal Configuration", "physical channels"="Sensor Physical Channel", "name to assign"="Acquisition Task") -> ("task out"=w100:refnum<k21>, "error out"=w101:errorcluster)  [unwired: 9 in]
  n31 = case shown="True" w51 {
    tunnel: ["No. Samples" w161] -> w39
    tunnel: "Sample Rate (Hz)" -> [_ w162]
    frame False {
    }
    frame True {
      n32 = local read "Pulse Basic"() -> (w160:T3)
      n33 = Unbundle By Name(w160) -> ("Basic freq (Hz)"=w159:u16)
      n34 = Divide(x=w162, y=w159) -> (x/y=w163:dbl)
      n35 = Round Toward -Infinity(1:w163) -> (0:w161:dbl)
      n36 = local write "No. Samples"(w161) -> ()
    }
  }
  n37 = call-poly <vilib>:"Create Modbus Instance.vi"("flow control (none)"=w18, "serial type"=enum16{"RTU", "ASCII"}."ASCII", "parity (even)"=w17, "unit ID"=u8 1, "baud rate"=u32 9600, "VISA resource name"="COM") -> ("error out"=w6:errorcluster, "serial master instance"=w7:refnum<class "Modbus Master.lvclass">)  [unwired: 4 in]
  n38 = local read "Pulse Basic"() -> (w52:T3)
  n39 = call-poly <vilib>:"DAQmx Timing.vi"("task/channels in"=w100, "sample mode"=w90, "samples per channel"=w39, "rate"="Sample Rate (Hz)", "source"="Sample Clock Source 2", "error in"=w101) -> ("task out"=w58:refnum<k21>, "error out"=w102:errorcluster)  [unwired: 8 in]
  n40 = Unbundle By Name(w52) -> ("Basic freq (Hz)"=w50:u16)
  n41 = Multiply(x="Speed (mm/s) 2", y=i16 1040 ("Speed (mm/s)")) -> (x*y=w11:i16)
  n42 = property class="DAQmx Timing"(reference=w58, error in=w102) -> (reference out=w56:refnum<k21>, error out=w55:errorcluster, "SampClk.Rate"=w49:dbl)
  "Actual Sample Rate" <- w49
  n43 = call-dynamic "Write Single Holding Register.vi"("error in"=w6, "register to write"=w11, "address"=u16 4096, "Modbus master in"=w7) -> ("error out"=w8:errorcluster, "Modbus master out"=w9:refnum<class "Modbus Master.lvclass">)  [unwired: 6 in]
  n44 = local write "Init pulses"(0 ("Init pulses")) -> ()
  n45 = case shown="True" "Encoder" {
    frame False {
    }
    frame True {
      # "Counter pulses from Motor\nto pick up signal"
      n46 = call-poly <vilib>:"DAQmx Create Virtual Channel.vi"("counter"="Motor counter X") -> ("task out"=w169:refnum<k21>, "error out"=w168:errorcluster)  [unwired: 13 in]
      n47 = call-poly <vilib>:"DAQmx Create Virtual Channel.vi"("counter"="Motor counter Y") -> ("task out"=w166:refnum<k21>, "error out"=w165:errorcluster)  [unwired: 13 in]
      n48 = property class="DAQmx Channel"(reference=w169, error in=w168, "CI.CountEdges.Term"="Motor Counter X") -> (reference out=w182:refnum<k21>, error out=w183:errorcluster)
      n49 = property class="DAQmx Channel"(reference=w166, error in=w165, "CI.CountEdges.Term"="Motor Counter Y") -> (reference out=w178:refnum<k21>, error out=w177:errorcluster)
      n50 = call <vilib>:"DAQmx Start Task.vi"("task/channels in"=w178, "error in"=w177) -> ("task out"=w176:refnum<k21>, "error out"=w175:errorcluster)  [unwired: 12 in]
      n51 = call <vilib>:"DAQmx Start Task.vi"("task/channels in"=w182, "error in"=w183) -> ("task out"=w184:refnum<k21>, "error out"=w181:errorcluster)  [unwired: 12 in]
      n52 = while {
        tunnel: w184 -> [w211]
        tunnel: w181 -> [w210]
        tunnel: [w204] -> w189
        tunnel: [w209] -> w188
        shift-right: [w203] -> _
        shift-left: u32 0 ("data") -> [w202]
        tunnel: w176 -> [w198]
        tunnel: w175 -> [w197]
        tunnel: [w196] -> w171
        tunnel: [w195] -> w170
        shift-right: [w192] -> _
        shift-left: u32 0 ("data") -> [w193]
        i -> [w199]
        stop <- w205 stop-if-true
        n53 = local read "Scan"() -> (w200:bool)
        n54 = call-poly <vilib>:"DAQmx Read.vi"("task/channels in"=w198, "error in"=w197) -> ("task out"=w196:refnum<k21>, "data"=→"Motor Pulses Y":u32, "error out"=w195:errorcluster)  [unwired: 11 in]
        n55 = call-poly <vilib>:"DAQmx Read.vi"("task/channels in"=w211, "error in"=w210) -> ("task out"=w209:refnum<k21>, "data"=w201:u32, "error out"=w204:errorcluster)  [unwired: 11 in]
        "Motor Pulses X" <- w201
        n56 = case shown="True" w200 {
          tunnel: [w213 w226] -> w203
          tunnel: w202 -> [w213 w225]
          tunnel: w201 -> [_ w218]
          tunnel: w193 -> [w212 w216]
          tunnel: [w212 w215] -> w192
          frame False {
          }
          frame True {
            n57 = local read "Init pulses"() -> (w214:i32)
            n58 = Subtract(x=w218, y=w214) -> (x-y=w217:u32)
            n59 = local read "X Step"() -> (w224:dbl)
            n60 = Multiply(x=w224, y=5.0) -> (x*y=w222:dbl)
            n61 = To Long Integer(number=w222) -> (32bit integer=w221:i32)
            n62 = Add(x=w221, y=w225) -> (x+y=w220:u32)
            n63 = Greater Or Equal?(x=w217, y=w220) -> (x >= y?=w219:bool)
            n64 = case shown="True" w219 {
              selector: w219 -> [_ w230]
              tunnel: w216 -> [w227 w229]
              tunnel: [w227 w228] -> w215
              frame False {
              }
              frame True {
                n65 = Increment(x=w229) -> (x+1=w228:u32)
                "Get data" <- w230
              }
            }
            n66 = Select(t=w217, s=w219, f=w225) -> (s? t:f=w226:u32)
          }
        }
        "Get data Count" <- w192
        n67 = Wait Until Next ms Multiple(millisecond multiple=u32 10 ("milliseconds to wait")) -> ()  [unwired: 1 out]
        n68 = local read "Completed"() -> (w206:bool)
        n69 = Unbundle By Name(w204) -> ("status"=w207:bool)
        n70 = Compound Arithmetic op=OR(w207, w206) -> (w205:bool)
        "Numeric  4" <- w199
      }
      n71 = call <vilib>:"DAQmx Stop Task.vi"("task/channels in"=w188, "error in"=w189) -> ("task out"=w191:refnum<k21>, "error out"=w190:errorcluster)  [unwired: 12 in]
      n72 = call <vilib>:"DAQmx Stop Task.vi"("task/channels in"=w171, "error in"=w170) -> ("task out"=w172:refnum<k21>, "error out"=w173:errorcluster)  [unwired: 12 in]
      n73 = call <vilib>:"DAQmx Clear Task.vi"("task in"=w191, "error in"=w190) -> ("error out"=w185:errorcluster)  [unwired: 13 in]
      n74 = call <vilib>:"DAQmx Clear Task.vi"("task in"=w172, "error in"=w173) -> ("error out"=w174:errorcluster)  [unwired: 13 in]
      n75 = call <vilib>:"Simple Error Handler.vi"("error in (no error)"=w185) -> ()  [unwired: 4 in, 5 out]
      n76 = call <vilib>:"Simple Error Handler.vi"("error in (no error)"=w174) -> ()  [unwired: 4 in, 5 out]
    }
  }
  n77 = while {
    shift-right: [w243] -> _
    shift-left: w9 -> [w245]
    shift-right: [w240] -> _
    shift-left: w8 -> [w244]
    tunnel: [w238] -> _
    tunnel: [w239] -> _
    stop <- w250 stop-if-true
    n78 = call-dynamic "Read Exception Status.vi"("error in"=w244, "Modbus master in"=w245) -> ("error out"=w246:errorcluster, "exception status"=w248:u8)  [unwired: 7 in, 1 out]
    "exception status" <- w248
    n79 = call <vilib>:"Clear Errors.vi"("error in (no error)"=w246) -> ()  [unwired: 5 in, 2 out]
    n80 = Not Equal To 0?(x=w248) -> (x != 0?=→"PLC Connceted":bool)
    n81 = event shown="[8] \"Down Z\": Value Change" {
      selector: _ -> [_ _ _ _ _ _ _ _ _ _]
      dyn-events: _ -> [_ _ _ _ _ _ _ _ _ _]
      timeout: 100 -> [_ _ _ _ _ _ _ _ _ _]
      tunnel: w245 -> [w255 w265 w282 w284 w294 w304 w315 w325 w338 w366]
      tunnel: [w256 w260 w281 w291 w302 w311 w322 w332 w334 w344] -> w243
      tunnel: w244 -> [w254 w264 w280 w283 w293 w305 w314 w324 w337 w365]
      tunnel: [w257 w259 w279 w290 w301 w310 w321 w331 w333 w343] -> w240
      event Timeout {
        n82 = event-data() -> ()  [unwired: 1 in, 3 out]
        n83 = call "Move_Completed.vi"("serial master instance"=w255, "error in"=w254) -> ("Modbus master out"=w256:refnum<class "Modbus Master.lvclass">, "Z completed"=→"Z complete":bool, "Y completed"=→"Y complete":bool, "X completed"=→"X complete":bool, "error out"=w257:errorcluster)  [unwired: 9 in]
      }
      event "Stop Button": Value Change {
        n84 = event-data() -> ()  [unwired: 1 in, 6 out]
        n85 = call-dynamic "Write Single Coil.vi"("error in"=w264, "coil to write"="Stop Button", "address"=u16 2055, "Modbus master in"=w265) -> ("error out"=w262:errorcluster, "Modbus master out"=w261:refnum<class "Modbus Master.lvclass">)  [unwired: 6 in]
        n86 = case shown="True" "Stop Button" {
          tunnel: w261 -> [w266 w272]
          tunnel: w262 -> [w267 w271]
          tunnel: [w266 w270] -> w260
          tunnel: [w267 w269] -> w259
          frame False {
          }
          frame True {
            n87 = Wait (ms)(milliseconds to wait=u32 100 ("millisecond timer value")) -> ()  [unwired: 1 out]
            n88 = call-dynamic "Write Single Coil.vi"("error in"=w271, "coil to write"=FALSE, "address"=u16 2055, "Modbus master in"=w272) -> ("error out"=w269:errorcluster, "Modbus master out"=w270:refnum<class "Modbus Master.lvclass">)  [unwired: 6 in]
          }
        }
      }
      event "Speed (mm/s) 2": Value Change {
        n89 = event-data() -> ()  [unwired: 1 in, 6 out]
        n90 = local read "Speed (mm/s) 2"() -> (w275:i16)
        n91 = Multiply(x=w275, y=i16 1040 ("Speed (mm/s)")) -> (x*y=w277:i16)
        n92 = call-dynamic "Write Single Holding Register.vi"("error in"=w280, "register to write"=w277, "address"=u16 4096, "Modbus master in"=w282) -> ("error out"=w279:errorcluster, "Modbus master out"=w281:refnum<class "Modbus Master.lvclass">)  [unwired: 6 in]
      }
      event "X RIGHT": Value Change {
        n93 = event-data() -> ()  [unwired: 1 in, 6 out]
        n94 = call-dynamic "Write Single Holding Register.vi"("error in"=w283, "register to write"="X Distance", "address"=u16 4100, "Modbus master in"=w284) -> ("error out"=w285:errorcluster, "Modbus master out"=w286:refnum<class "Modbus Master.lvclass">)  [unwired: 6 in]
        n95 = call-dynamic "Write Single Coil.vi"("error in"=w285, "coil to write"="X RIGHT", "address"=u16 2052, "Modbus master in"=w286) -> ("error out"=w290:errorcluster, "Modbus master out"=w291:refnum<class "Modbus Master.lvclass">)  [unwired: 6 in]
      }
      event "X LEFT": Value Change {
        n96 = event-data() -> ()  [unwired: 1 in, 6 out]
        n97 = local read "X Distance"() -> (w295:u32)
        n98 = call-dynamic "Write Single Holding Register.vi"("error in"=w293, "register to write"=w295, "address"=u16 4100, "Modbus master in"=w294) -> ("error out"=w296:errorcluster, "Modbus master out"=w297:refnum<class "Modbus Master.lvclass">)  [unwired: 6 in]
        n99 = call-dynamic "Write Single Coil.vi"("error in"=w296, "coil to write"="X LEFT", "address"=u16 2051, "Modbus master in"=w297) -> ("error out"=w301:errorcluster, "Modbus master out"=w302:refnum<class "Modbus Master.lvclass">)  [unwired: 6 in]
      }
      event "Y FW": Value Change {
        n100 = event-data() -> ()  [unwired: 1 in, 6 out]
        n101 = call-dynamic "Write Single Holding Register.vi"("error in"=w305, "register to write"="Y Distance", "address"=u16 4098, "Modbus master in"=w304) -> ("error out"=w306:errorcluster, "Modbus master out"=w307:refnum<class "Modbus Master.lvclass">)  [unwired: 6 in]
        n102 = call-dynamic "Write Single Coil.vi"("error in"=w306, "coil to write"="Y FW", "address"=u16 2049, "Modbus master in"=w307) -> ("error out"=w310:errorcluster, "Modbus master out"=w311:refnum<class "Modbus Master.lvclass">)  [unwired: 6 in]
      }
      event "Y BW": Value Change {
        n103 = event-data() -> ()  [unwired: 1 in, 6 out]
        n104 = local read "Y Distance"() -> (w313:u32)
        n105 = call-dynamic "Write Single Holding Register.vi"("error in"=w314, "register to write"=w313, "address"=u16 4098, "Modbus master in"=w315) -> ("error out"=w316:errorcluster, "Modbus master out"=w317:refnum<class "Modbus Master.lvclass">)  [unwired: 6 in]
        n106 = call-dynamic "Write Single Coil.vi"("error in"=w316, "coil to write"="Y BW", "address"=u16 2050, "Modbus master in"=w317) -> ("error out"=w321:errorcluster, "Modbus master out"=w322:refnum<class "Modbus Master.lvclass">)  [unwired: 6 in]
      }
      event "Up Z": Value Change {
        n107 = event-data() -> ()  [unwired: 1 in, 6 out]
        n108 = call-dynamic "Write Single Holding Register.vi"("error in"=w324, "register to write"="Z Distance", "address"=u16 4102, "Modbus master in"=w325) -> ("error out"=w327:errorcluster, "Modbus master out"=w326:refnum<class "Modbus Master.lvclass">)  [unwired: 6 in]
        n109 = call-dynamic "Write Single Coil.vi"("error in"=w327, "coil to write"="Up Z", "address"=u16 2053, "Modbus master in"=w326) -> ("error out"=w331:errorcluster, "Modbus master out"=w332:refnum<class "Modbus Master.lvclass">)  [unwired: 6 in]
      }
      event "Down Z": Value Change {
        n110 = event-data() -> ()  [unwired: 1 in, 6 out]
        n111 = local read "Z Distance"() -> (w339:i16)
        n112 = call-dynamic "Write Single Holding Register.vi"("error in"=w337, "register to write"=w339, "address"=u16 4102, "Modbus master in"=w338) -> ("error out"=w335:errorcluster, "Modbus master out"=w336:refnum<class "Modbus Master.lvclass">)  [unwired: 6 in]
        n113 = call-dynamic "Write Single Coil.vi"("error in"=w335, "coil to write"="Down Z", "address"=u16 2054, "Modbus master in"=w336) -> ("error out"=w333:errorcluster, "Modbus master out"=w334:refnum<class "Modbus Master.lvclass">)  [unwired: 6 in]
      }
      event "Home 2": Value Change {
        w349 = u16 650 ("register to write")
        n114 = event-data() -> ()  [unwired: 1 in, 6 out]
        n115 = call-dynamic "Write Single Holding Register.vi"("error in"=w365, "register to write"=u16 300, "address"=u16 4102, "Modbus master in"=w366) -> ("error out"=w362:errorcluster, "Modbus master out"=w361:refnum<class "Modbus Master.lvclass">)  [unwired: 6 in]
        n116 = call-dynamic "Write Single Coil.vi"("error in"=w362, "coil to write"="Home 2", "address"=u16 2053, "Modbus master in"=w361) -> ("error out"=w364:errorcluster, "Modbus master out"=w367:refnum<class "Modbus Master.lvclass">)  [unwired: 6 in]
        n117 = call-dynamic "Write Single Coil.vi"("error in"=w364, "coil to write"=TRUE, "address"=u16 2050, "Modbus master in"=w367) -> ("error out"=w356:errorcluster, "Modbus master out"=w357:refnum<class "Modbus Master.lvclass">)  [unwired: 6 in]
        n118 = call-dynamic "Write Single Coil.vi"("error in"=w356, "coil to write"=TRUE, "address"=u16 2051, "Modbus master in"=w357) -> ("error out"=w354:errorcluster, "Modbus master out"=w355:refnum<class "Modbus Master.lvclass">)  [unwired: 6 in]
        n119 = call-dynamic "Write Single Holding Register.vi"("error in"=w354, "register to write"=w349, "address"=u16 4098, "Modbus master in"=w355) -> ("error out"=w352:errorcluster, "Modbus master out"=w353:refnum<class "Modbus Master.lvclass">)  [unwired: 6 in]
        n120 = call-dynamic "Write Single Holding Register.vi"("error in"=w352, "register to write"=w349, "address"=u16 4100, "Modbus master in"=w353) -> ("error out"=w343:errorcluster, "Modbus master out"=w344:refnum<class "Modbus Master.lvclass">)  [unwired: 6 in]
      }
    }
    n121 = call-dynamic "Read Discrete Inputs.vi"("error in"=w240, "number of inputs"=u16 6, "starting address"=u16 1024, "Modbus master in"=w243) -> ("error out"=w239:errorcluster, "discrete inputs"=w237:bool[], "Modbus master out"=w238:refnum<class "Modbus Master.lvclass">)  [unwired: 5 in]
    "Limit Sensor" <- w237
    n122 = Index Array(array=w237, index #1=4 ("index"), index #2=3 ("index"), index #3=0 ("index")) -> (element #1=→"Z UP Limit":bool, element #2=→"X L Limit":bool, element #3=→"Y Back Limit":bool)
    n123 = Unbundle By Name(w240) -> ("status"=w250:bool)
  }
  n124 = while {
    shift-right: [w378] -> _
    shift-left: T1."No Scan" -> [w379]
    shift-right: [w376] -> _
    shift-left: 0 -> [w377]
    tunnel: w7 -> [w371]
    tunnel: [w370] -> _
    tunnel: w6 -> [w369]
    tunnel: [w368] -> _
    stop <- w373 stop-if-true
    # "AUTO SCAN"
    n125 = local read "Scan"() -> (w372:bool)
    n126 = case shown="True" w372 {
      tunnel: w379 -> [w382 w392]
      tunnel: [w382 w391] -> w378
      tunnel: w377 -> [w383 w389]
      tunnel: [w383 w388] -> w376
      tunnel: w371 -> [w381 w387]
      tunnel: [w381 w386] -> w370
      tunnel: w369 -> [w380 w385]
      tunnel: [w380 w384] -> w368
      frame False {
      }
      frame True {
        n127 = case shown="\"Move Y\"" w392 {
          selector: w392 -> [w400 _ _ _ _]
          tunnel: [w399 T1."Wait X" w457 w484 w503] -> w391
          tunnel: w389 -> [w398 w436 w455 w483 w502]
          tunnel: [w398 w436 w455 w483 w501] -> w388
          tunnel: w387 -> [w396 w425 w451 w478 w499]
          tunnel: [w394 w430 w453 w481 w497] -> w386
          tunnel: w385 -> [w395 w424 w450 w477 w498]
          tunnel: [w393 w429 w452 w480 w496] -> w384
          frame "No Scan", Default {
            n128 = local read "Scan"() -> (w397:bool)
            n129 = case shown="True" w397 {
              tunnel: w400 -> [w403 _]
              tunnel: [w403 T1."Move X"] -> w399
              tunnel: w396 -> [w402 w419]
              tunnel: w395 -> [w401 w418]
              tunnel: [w402 w408] -> w394
              tunnel: [w401 w407] -> w393
              frame False {
              }
              frame True {
                n130 = call-dynamic "Write Single Coil.vi"("error in"=w418, "coil to write"=FALSE ("X LEFT"), "address"=u16 2049, "Modbus master in"=w419) -> ("error out"=w406:errorcluster, "Modbus master out"=w411:refnum<class "Modbus Master.lvclass">)  [unwired: 6 in]
                n131 = call-dynamic "Write Single Coil.vi"("error in"=w406, "coil to write"=FALSE ("X LEFT"), "address"=u16 2050, "Modbus master in"=w411) -> ("error out"=w405:errorcluster, "Modbus master out"=w410:refnum<class "Modbus Master.lvclass">)  [unwired: 6 in]
                n132 = call-dynamic "Write Single Coil.vi"("error in"=w405, "coil to write"=FALSE ("X LEFT"), "address"=u16 2051, "Modbus master in"=w410) -> ("error out"=w404:errorcluster, "Modbus master out"=w409:refnum<class "Modbus Master.lvclass">)  [unwired: 6 in]
                n133 = call-dynamic "Write Single Coil.vi"("error in"=w404, "coil to write"=FALSE ("X LEFT"), "address"=u16 2052, "Modbus master in"=w409) -> ("error out"=w407:errorcluster, "Modbus master out"=w408:refnum<class "Modbus Master.lvclass">)  [unwired: 6 in]
              }
            }
          }
          frame "Move X" {
            n134 = local read "Count Y step"() -> (w432:i32)
            n135 = Quotient & Remainder(x=w432, y=2) -> (x-y*floor(x/y)=w431:i32)  [unwired: 1 out]
            n136 = Equal?(x=w431, y=0) -> (x = y?=w433:bool)
            n137 = call-dynamic "Write Single Holding Register.vi"("error in"=w424, "register to write"="X Auto Distance", "address"=u16 4100, "Modbus master in"=w425) -> ("error out"=w426:errorcluster, "Modbus master out"=w427:refnum<class "Modbus Master.lvclass">)  [unwired: 6 in]
            n138 = case shown="True" w433 {
              tunnel: w427 -> [w443 w447]
              tunnel: [w442 w445] -> w430
              tunnel: w426 -> [w441 w446]
              tunnel: [w440 w444] -> w429
              frame False {
                n139 = call-dynamic "Write Single Coil.vi"("error in"=w441, "coil to write"=TRUE ("X LEFT"), "address"=u16 2051, "Modbus master in"=w443) -> ("error out"=w440:errorcluster, "Modbus master out"=w442:refnum<class "Modbus Master.lvclass">)  [unwired: 6 in]
              }
              frame True {
                n140 = call-dynamic "Write Single Coil.vi"("error in"=w446, "coil to write"=TRUE ("X LEFT"), "address"=u16 2052, "Modbus master in"=w447) -> ("error out"=w444:errorcluster, "Modbus master out"=w445:refnum<class "Modbus Master.lvclass">)  [unwired: 6 in]
              }
            }
            "Count Y step" <- w436
          }
          frame "Wait X" {
            n141 = local read "X complete"() -> (w454:bool)
            n142 = Wait (ms)(milliseconds to wait=u32 100) -> ()  [unwired: 1 out]
            n143 = case shown="False" w454 {
              tunnel: [T1."Wait X" T1."Move Y"] -> w457
              tunnel: [w459 w464] -> w453
              tunnel: [w458 w463] -> w452
              tunnel: w451 -> [w459 w462]
              tunnel: w450 -> [w458 w461]
              frame False {
              }
              frame True {
                n144 = call-dynamic "Write Single Coil.vi"("error in"=w461, "coil to write"=FALSE ("X LEFT"), "address"=u16 2051, "Modbus master in"=w462) -> ("error out"=w465:errorcluster, "Modbus master out"=w466:refnum<class "Modbus Master.lvclass">)  [unwired: 6 in]
                n145 = call-dynamic "Write Single Coil.vi"("error in"=w465, "coil to write"=FALSE ("X LEFT"), "address"=u16 2052, "Modbus master in"=w466) -> ("error out"=w463:errorcluster, "Modbus master out"=w464:refnum<class "Modbus Master.lvclass">)  [unwired: 6 in]
              }
            }
          }
          frame "Move Y" {
            n146 = local read "Y Step"() -> (w472:dbl)
            n147 = Divide(x="Y Auto Distance", y=w472) -> (x/y=w473:dbl)
            "Step Y Number" <- w473
            n148 = call-dynamic "Write Single Holding Register.vi"("error in"=w477, "register to write"=w472, "address"=u16 4098, "Modbus master in"=w478) -> ("error out"=w475:errorcluster, "Modbus master out"=w476:refnum<class "Modbus Master.lvclass">)  [unwired: 6 in]
            n149 = Greater Or Equal?(x=w483, y=w473) -> (x >= y?=w482:bool)
            n150 = case shown="False" w482 {
              tunnel: [T1."Wait Y" T1."No Scan"] -> w484
              tunnel: w476 -> [w488 w493]
              tunnel: w475 -> [w487 w492]
              tunnel: [w486 w493] -> w481
              tunnel: [w485 w492] -> w480
              frame False {
                n151 = call-dynamic "Write Single Coil.vi"("error in"=w487, "coil to write"=TRUE ("X LEFT"), "address"=u16 2050, "Modbus master in"=w488) -> ("error out"=w485:errorcluster, "Modbus master out"=w486:refnum<class "Modbus Master.lvclass">)  [unwired: 6 in]
              }
              frame True {
                n152 = local write "Scan"(FALSE ("X LEFT")) -> ()
              }
            }
          }
          frame "Wait Y" {
            n153 = local read "Y complete"() -> (w500:bool)
            n154 = case shown="False" w500 {
              tunnel: [T1."Wait Y" T1."Move X"] -> w503
              tunnel: w502 -> [w506 w515]
              tunnel: [w506 w514] -> w501
              tunnel: w499 -> [w505 w511]
              tunnel: w498 -> [w504 w510]
              tunnel: [w505 w509] -> w497
              tunnel: [w504 w508] -> w496
              frame False {
              }
              frame True {
                n155 = Increment(x=w515) -> (x+1=w514:i32)
                n156 = Wait (ms)(milliseconds to wait=u32 100) -> ()  [unwired: 1 out]
                n157 = call-dynamic "Write Single Coil.vi"("error in"=w510, "coil to write"=FALSE ("X LEFT"), "address"=u16 2050, "Modbus master in"=w511) -> ("error out"=w508:errorcluster, "Modbus master out"=w509:refnum<class "Modbus Master.lvclass">)  [unwired: 6 in]
              }
            }
          }
        }
        n158 = Wait Until Next ms Multiple(millisecond multiple=u32 100 ("milliseconds to wait")) -> ()  [unwired: 1 out]
      }
    }
    n159 = local read "Exit"() -> (w375:bool)
    n160 = Compound Arithmetic op=OR(w375, "Stop Scan") -> (w373:bool)
    "Enum 2" <- w379
  }
  n161 = call-poly <vilib>:"DAQmx Trigger.vi"("task/channels in"=w56, "source"="Pulser Trigger", "edge"="Edge", "error in"=w55) -> ("task out"=w5:refnum<k21>, "error out"=w4:errorcluster)  [unwired: 10 in]
  n162 = case shown="True" "DAQ Pulser" {
    tunnel: w4 -> [_ w548]
    frame False {
    }
    frame True {
      (unwired) 1 ("x")
      w545 = 10123 items=["Finite Samples"=10178, "Continuous Samples"=10123, "Hardware Timed Single Point"=12522]  # Sample Mode
      n163 = local read "Pulse Basic"() -> (w519:T3)
      n164 = Unbundle By Name(w519) -> ("Basic freq (Hz)"=w518:u16)
      n165 = call-poly <vilib>:"DAQmx Create Virtual Channel.vi"("maximum value"="Max Voltage 2", "minimum value"="Min Voltage 2", "physical channels"="Physical Channel(s)", "name to assign"="Pulser Task", "error in"=w548) -> ("task out"=w539:refnum<k21>, "error out"=w538:errorcluster)  [unwired: 9 in]
      n166 = Divide(x="Sample Rate 2", y=w518) -> (x/y=w536:dbl)
      n167 = Multiply(x="Pulser Cycles", y=w536) -> (x*y=w535:dbl)
      n168 = Round Toward -Infinity(1:w535) -> (0:w527:dbl)
      "Sample per Channel AO" <- w527
      n169 = call-poly <vilib>:"DAQmx Timing.vi"("task/channels in"=w539, "sample mode"=w545, "samples per channel"=w527, "rate"="Sample Rate 2", "source"="Sample Clock Source", "error in"=w538) -> ("task out"=w547:refnum<k21>, "error out"=w546:errorcluster)  [unwired: 8 in]
      n170 = property class="DAQmx Timing"(reference=w547, error in=w546) -> (reference out=w534:refnum<k21>, error out=w520:errorcluster, "SampClk.Rate"=w522:dbl)
      "Actual Sample Rate 2" <- w522
      n171 = call "waveform_generator.vi"("Sampling rate"=w522, "Pulse chirp"="Pulse chirp", "Pulse Gaussian"="Pulse Gaussian", "Cluster Basic"="Pulse Basic", "Tab Control"="Tab Control 4") -> ("Waveform Graph"=w521:waveform(dbl)[])  [unwired: 6 in]
      n172 = disable-structure shown="Enabled" {
        disable-tunnel: w521 -> [w553 w574]
        disable-tunnel: [w552 w577] -> w531
        disable-tunnel: [w551 w576] -> w528
        disable-tunnel: w534 -> [w550 w578]
        disable-tunnel: w520 -> [w549 w573]
        frame Disabled {
          n173 = while {
            tunnel: w553 -> [w564]
            shift-right: [w560] -> w552
            shift-left: w550 -> [w558]
            shift-right: [w559] -> w551
            shift-left: w549 -> [w557]
            stop <- FALSE stop-if-true
            n174 = call-poly <vilib>:"DAQmx Write.vi"("task/channels in"=w558, "data"=w564, "timeout"=-1.0, "error in"=w557) -> ("task out"=w563:refnum<k21>, "error out"=w562:errorcluster)  [unwired: 9 in, 1 out]
            n175 = call <vilib>:"DAQmx Start Task.vi"("task/channels in"=w563, "error in"=w562) -> ("task out"=w556:refnum<k21>, "error out"=w555:errorcluster)  [unwired: 12 in]
            n176 = disable-structure shown="Enabled" {
              disable-tunnel: [w570 w572] -> w560
              disable-tunnel: [w569 w571] -> w559
              disable-tunnel: w556 -> [w568 w572]
              disable-tunnel: w555 -> [w567 w571]
              frame Disabled {
                n177 = call <vilib>:"DAQmx Wait Until Done.vi"("task/channels in"=w568, "error in"=w567) -> ("task out"=w566:refnum<k21>, "error out"=w565:errorcluster)  [unwired: 12 in]
                n178 = call <vilib>:"DAQmx Stop Task.vi"("task/channels in"=w566, "error in"=w565) -> ("task out"=w570:refnum<k21>, "error out"=w569:errorcluster)  [unwired: 12 in]
              }
              frame Enabled {
              }
            }
          }
        }
        frame Enabled {
          n179 = call-poly <vilib>:"DAQmx Write.vi"("task/channels in"=w578, "data"=w574, "timeout"=-1.0, "error in"=w573) -> ("task out"=w580:refnum<k21>, "error out"=w582:errorcluster)  [unwired: 9 in, 1 out]
          n180 = call <vilib>:"DAQmx Start Task.vi"("task/channels in"=w580, "error in"=w582) -> ("task out"=w579:refnum<k21>, "error out"=w581:errorcluster)  [unwired: 12 in]
          n181 = while {
            tunnel: w579 -> [w590]
            tunnel: w581 -> [w589]
            tunnel: [w587] -> w576
            tunnel: [w588] -> w577
            stop <- w584 stop-if-true
            n182 = call <vilib>:"DAQmx Is Task Done.vi"("task/channels in"=w590, "error in"=w589) -> ("task out"=w588:refnum<k21>, "error out"=w587:errorcluster)  [unwired: 11 in, 1 out]
            n183 = Unbundle By Name(w587) -> ("status"=w585:bool)
            n184 = local read "Exit"() -> (w583:bool)
            n185 = Wait Until Next ms Multiple(millisecond multiple=u32 100) -> ()  [unwired: 1 out]
            n186 = Compound Arithmetic op=OR(w585, w583) -> (w584:bool)
          }
        }
      }
      n187 = call <vilib>:"DAQmx Stop Task.vi"("task/channels in"=w531, "error in"=w528) -> ("task out"=w530:refnum<k21>, "error out"=w529:errorcluster)  [unwired: 12 in]
      n188 = call <vilib>:"DAQmx Clear Task.vi"("task in"=w530, "error in"=w529) -> ("error out"=w544:errorcluster)  [unwired: 13 in]
      n189 = call <vilib>:"Simple Error Handler.vi"("error in (no error)"=w544) -> ()  [unwired: 4 in, 5 out]
    }
  }
  n190 = local read "Y Auto Distance"() -> (w54:i16)
  n191 = local read "X Auto Distance"() -> (w79:u16)
  n192 = local read "Y Step"() -> (w77:dbl)
  n193 = local read "X Step"() -> (w78:dbl)
  n194 = Obtain Queue(name (unnamed)="data Extraction1", element data type=0.0) -> (queue out=w31:refnum<queue>)  [unwired: 3 in, 2 out]
  n195 = Obtain Queue(max queue size (-1, unlimited)=10000, name (unnamed)="data DAQ1", element data type=dbl[] [] ("data")) -> (queue out=w41:refnum<queue>)  [unwired: 2 in, 2 out]
  n196 = Quotient & Remainder(x=w54, y=w77) -> (floor(x/y)=w59:dbl)  [unwired: 1 out]
  n197 = Quotient & Remainder(x=w79, y=w78) -> (floor(x/y)=w23:dbl)  [unwired: 1 out]
  n198 = Obtain Queue(max queue size (-1, unlimited)=10000, name (unnamed)="data DAQ", element data type=dbl[] [] ("data")) -> (queue out=w84:refnum<queue>)  [unwired: 2 in, 2 out]
  n199 = Initialize Array(0.0 ("element"), w39) -> (w38:dbl[])
  n200 = Increment(x=w59) -> (x+1=w22:dbl)
  n201 = Build Array(w50, w49, w23, w22) -> (w64:dbl[])
  n202 = Build Array(w50, w49, w23, w22) -> (w45:dbl[])
  n203 = TDMS Write(0:w74, 5:"Freq_Sampling_SizeX_SizeY" ("group name in (Untitled)"), 9:w64) -> (4:w73:refnum<k34>)  [unwired: 3 in, 3 out]
  n204 = TDMS Write(0:w48, 5:"Freq_Sampling_SizeX_SizeY" ("group name in (Untitled)"), 9:w45) -> (4:w30:refnum<k34>)  [unwired: 3 in, 3 out]
  n205 = call "PECT_GateConverse.vi"("Gate 2"="Gate 2", "Gate 1"="Gate 1", "Freq_Sampling_SizeX_SizeY"=w64) -> ("Length T/2"=w65:i32, "Length"=w66:i32, "Start 2"=w67:i32, "Start 1"=w68:i32)  [unwired: 4 in, 1 out]
  n206 = call "PECT_GateConverse.vi"("Gate 2"="Gate 4", "Gate 1"="Gate 3", "Freq_Sampling_SizeX_SizeY"=w45) -> ("Length T/2"=w34:i32, "Length"=w35:i32, "Start 2"=w36:i32, "Start 1"=w37:i32)  [unwired: 4 in, 1 out]
  n207 = Initialize Array(0.0 ("element"), w39) -> (w85:dbl[])
  n208 = Obtain Queue(max queue size (-1, unlimited)=2 ("최대 큐 크기(-1,제한없음)"), name (unnamed)="2D data1", element data type=dbl[][] [] ("initialized array")) -> (queue out=w26:refnum<queue>)  [unwired: 2 in, 2 out]
  n209 = Obtain Queue(name (unnamed)="data Extraction", element data type=0.0) -> (queue out=w82:refnum<queue>)  [unwired: 3 in, 2 out]
  n210 = Obtain Queue(max queue size (-1, unlimited)=2 ("최대 큐 크기(-1,제한없음)"), name (unnamed)="2D data", element data type=dbl[][] [] ("initialized array")) -> (queue out=w61:refnum<queue>)  [unwired: 2 in, 2 out]
  n211 = case shown="\"Test mode                   \"" "Tab Control 2" {
    tunnel: w5 -> [w653 w1058 w1092]
    tunnel: [w652 w1058 w1091] -> w93
    tunnel: [w651 w1057 w1090] -> w92
    tunnel: w85 -> [w648 _ w1089]
    tunnel: w4 -> [w650 w1057 w1088]
    tunnel: w65 -> [w649 _ w1087]
    tunnel: w84 -> [w647 _ _]
    tunnel: w82 -> [w627 _ _]
    tunnel: w23 -> [w596 _ _]
    tunnel: w22 -> [w607 _ _]
    tunnel: w66 -> [w635 _ w1085]
    tunnel: w68 -> [w634 _ w1084]
    tunnel: w67 -> [w633 _ w1080]
    tunnel: w73 -> [w632 _ _]
    tunnel: "Waveform" ("group name in (Untitled)") -> [w629 _ _]
    tunnel: w61 -> [w625 _ _]
    tunnel: w39 -> [w622 _ w1083]
    tunnel: w41 -> [w620 _ _]
    tunnel: w38 -> [w611 _ w1077]
    tunnel: w37 -> [w619 _ w1076]
    tunnel: w36 -> [w618 _ w1075]
    tunnel: w35 -> [w617 _ w1074]
    tunnel: w34 -> [w616 _ w1073]
    tunnel: w31 -> [w610 _ _]
    tunnel: w30 -> [w612 _ _]
    tunnel: w26 -> [w594 _ _]
    tunnel: "Waveform" ("group name in (Untitled)") -> [w592 _ _]
    frame "Scan mode                      ", Default {
      # "Column"
      # "Row"
      n212 = Initialize Array(0.0 ("element"), w596, w607) -> (w640:dbl[][])
      n213 = local read "3D Surface(0) (coil)"() -> (w636:refnum<k7>)
      n214 = Initialize Array(0.0 ("element"), w596, w607) -> (w598:dbl[][])
      n215 = local read "3D Surface (2)(Hall)"() -> (w601:refnum<k7>)
      n216 = Matrix Size(0:w598) -> (1:w606:i32, 2:w605:i32)
      n217 = Matrix Size(0:w640) -> (1:w641:i32, 2:w642:i32)
      n218 = Decrement(x=w606) -> (x-1=w602:i32)
      n219 = Decrement(x=w605) -> (x-1=w603:i32)
      n220 = Decrement(x=w641) -> (x-1=w645:i32)
      n221 = Decrement(x=w642) -> (x-1=w644:i32)
      n222 = call "Surface_AxesScale.vi"("Y-axis Max"=w603, "X-axis max"=w602, "3D Surface"=w601, "Auto Scale"=FALSE) -> ()  [unwired: 8 in]
      n223 = call "Surface_AxesScale.vi"("Y-axis Max"=w644, "X-axis max"=w645, "3D Surface"=w636, "Auto Scale"=FALSE) -> ()  [unwired: 8 in]
      n224 = while {
        tunnel: w653 -> [w884]
        tunnel: [w883] -> w652
        tunnel: [w882] -> w651
        tunnel: w650 -> [w881]
        tunnel: w647 -> [w880]
        tunnel: w622 -> [w876]
        tunnel: w620 -> [w875]
        stop <- w877 stop-if-true
        n225 = case shown="True" "Scan" {
          tunnel: w884 -> [w886 w893]
          tunnel: [w886 w892] -> w883
          tunnel: [w885 w891] -> w882
          tunnel: w881 -> [w885 w890]
          tunnel: w880 -> [_ w889]
          tunnel: w876 -> [_ w888]
          tunnel: w875 -> [_ w887]
          frame False {
          }
          frame True {
            n226 = while {
              tunnel: w893 -> [w911]
              tunnel: [w914] -> w892
              tunnel: [w913] -> w891
              tunnel: w890 -> [w910]
              tunnel: w889 -> [w912]
              tunnel: w888 -> [w894]
              tunnel: w887 -> [w902]
              stop <- w903 stop-if-true
              # "Coil"
              # "Hall"
              n227 = First Call?() -> (First Call?: T/F=w907:bool)
              n228 = case shown="True" w907 {
                tunnel: w911 -> [w915 w921]
                tunnel: w910 -> [w916 w920]
                tunnel: [w915 w919] -> w909
                tunnel: [w916 w918] -> w908
                frame False {
                }
                frame True {
                  n229 = local read "Motor Pulses X"() -> (→"Init pulses":i32)
                  n230 = call <vilib>:"DAQmx Start Task.vi"("task/channels in"=w921, "error in"=w920) -> ("task out"=w919:refnum<k21>, "error out"=w918:errorcluster)  [unwired: 12 in]
                }
              }
              n231 = call-poly <vilib>:"DAQmx Read.vi"("task/channels in"=w909, "number of samples per channel"=w894, "error in"=w908) -> ("task out"=w914:refnum<k21>, "data"=w898:waveform(dbl)[], "error out"=w913:errorcluster)  [unwired: 10 in]
              n232 = Index Array(array=w898, index=0 ("index (row)")) -> (element=w896:waveform(dbl))
              n233 = Index Array(array=w898, index=2 ("index (row)")) -> (element=w900:waveform(dbl))
              n234 = Unbundle By Name(w896) -> ("Y"=w895:dbl[])
              n235 = Unbundle By Name(w900) -> ("Y"=w899:dbl[])
              n236 = Enqueue Element(queue=w912, element=w895) -> ()  [unwired: 2 in, 3 out]
              n237 = Enqueue Element(queue=w902, element=w899) -> ()  [unwired: 2 in, 3 out]
              n238 = Unbundle By Name(w913) -> ("status"=w904:bool)
              n239 = local read "Completed"() -> (w906:bool)
              n240 = local read "Exit"() -> (w905:bool)
              n241 = Compound Arithmetic op=OR(w904, w906, w905) -> (w903:bool)
            }
          }
        }
        n242 = local read "Completed"() -> (w878:bool)
        n243 = local read "Exit"() -> (w879:bool)
        n244 = Compound Arithmetic op=OR(w878, w879) -> (w877:bool)
      }
      n245 = while {
        shift-right: [w951] -> _
        shift-left: w648 -> [w955]
        tunnel: w648 -> [w954]
        tunnel: w649 -> [w953]
        tunnel: w647 -> [w952]
        tunnel: w627 -> [w950]
        shift-right: [w947] -> _
        shift-left: 0 -> [w948]
        tunnel: w635 -> [w946]
        tunnel: w634 -> [w945]
        tunnel: w633 -> [w944]
        tunnel: w632 -> [w943]
        tunnel: [w942] -> w631
        tunnel: [w941] -> w630
        tunnel: w629 -> [w940]
        tunnel: w620 -> [w936]
        shift-right: [w934] -> _
        shift-left: w611 -> [w935]
        tunnel: w592 -> [w933]
        tunnel: w619 -> [w932]
        tunnel: w618 -> [w931]
        tunnel: w617 -> [w930]
        tunnel: w616 -> [w929]
        tunnel: w610 -> [w928]
        tunnel: [w927] -> w614
        tunnel: [w926] -> w613
        tunnel: w612 -> [w925]
        tunnel: w611 -> [w924]
        shift-right: [w923] -> _
        shift-left: 0 -> [w922]
        stop <- w937 stop-if-true
        n246 = local read "Scan"() -> (w949:bool)
        n247 = case shown="True" w949 {
          tunnel: w955 -> [w961 w978]
          tunnel: w954 -> [_ w995]
          tunnel: w953 -> [_ w994]
          tunnel: w952 -> [_ w993]
          tunnel: [w961 w964] -> w951
          tunnel: w950 -> [_ w992]
          tunnel: w948 -> [w960 w989]
          tunnel: [w960 w988] -> w947
          tunnel: w946 -> [_ w987]
          tunnel: w945 -> [_ w986]
          tunnel: w944 -> [_ w985]
          tunnel: w943 -> [w958 w984]
          tunnel: [w958 w983] -> w942
          tunnel: [_ w982] -> w941
          tunnel: w940 -> [_ w981]
          tunnel: w936 -> [_ w980]
          tunnel: w935 -> [w957 w977]
          tunnel: [w957 w971] -> w934
          tunnel: w933 -> [_ w965]
          tunnel: w932 -> [_ w975]
          tunnel: w931 -> [_ w974]
          tunnel: w930 -> [_ w973]
          tunnel: w929 -> [_ w972]
          tunnel: w928 -> [_ w967]
          tunnel: [_ w970] -> w927
          tunnel: [_ w969] -> w926
          tunnel: w925 -> [_ w966]
          tunnel: w924 -> [_ w968]
          tunnel: w922 -> [w956 w962]
          tunnel: [w956 w963] -> w923
          frame False {
            n248 = Wait Until Next ms Multiple(millisecond multiple=u32 100 ("ms 배수")) -> ()  [unwired: 1 out]
          }
          frame True {
            n249 = local read "Pulser Cycles"() -> (w990:i32)
            n250 = Increment(x=w989) -> (x+1=w988:i32)
            n251 = Dequeue Element(queue=w980) -> (element=w979:dbl[])  [unwired: 2 in, 3 out]
            n252 = Dequeue Element(queue=w993) -> (element=w991:dbl[])  [unwired: 2 in, 3 out]
            n253 = Quotient & Remainder(x=w988, y=w990) -> (x-y*floor(x/y)=w996:i32)  [unwired: 1 out]
            n254 = Add(x=w979, y=w977) -> (x+y=w976:dbl[])
            n255 = Add(x=w991, y=w978) -> (x+y=w998:dbl[])
            n256 = Equal To 0?(x=w996) -> (x = 0?=w997:bool)
            n257 = case shown="True" w997 {
              tunnel: w990 -> [_ w1024]
              tunnel: w998 -> [w1003 w1033]
              tunnel: [w1003 w1035] -> w964
              tunnel: w995 -> [_ w1035]
              tunnel: w994 -> [_ w1029]
              tunnel: w992 -> [_ w1034]
              tunnel: w987 -> [_ w1030]
              tunnel: w986 -> [_ w1032]
              tunnel: w985 -> [_ w1031]
              tunnel: w984 -> [w1002 w1028]
              tunnel: [w1002 w1026] -> w983
              tunnel: [_ w1025] -> w982
              tunnel: w981 -> [_ w1027]
              tunnel: w976 -> [w1001 w1010]
              tunnel: w975 -> [_ w1023]
              tunnel: w974 -> [_ w1022]
              tunnel: w973 -> [_ w1011]
              tunnel: w972 -> [_ w1012]
              tunnel: [w1001 w1020] -> w971
              tunnel: [w1000 w1016] -> w970
              tunnel: [_ w1015] -> w969
              tunnel: w968 -> [_ w1020]
              tunnel: w967 -> [_ w1019]
              tunnel: w966 -> [w1000 w1018]
              tunnel: w965 -> [_ w1017]
              tunnel: w962 -> [w999 _]
              tunnel: [w999 w1005] -> w963
              tunnel: w962 -> [_ w1006]
              frame False {
                n258 = disable-structure shown="Enabled" {
                  frame Disabled {
                    n259 = Wait Until Next ms Multiple(millisecond multiple=u32 100 ("ms 배수")) -> ()  [unwired: 1 out]
                  }
                  frame Enabled {
                  }
                }
              }
              frame True {
                n260 = Divide(x=w1010, y=w1024) -> (x/y=w1008:dbl[])
                n261 = Divide(x=w1033, y=w1024) -> (x/y=w1009:dbl[])
                n262 = local read "Offset"() -> (w1021:bool)
                n263 = call "PECT_Feature extraction.vi"("Length T/2"=w1029, "Offset"=w1021, "Length"=w1030, "Start 2"=w1031, "Start 1"=w1032, "Pulse signal in"=w1009) -> ("Feature extraction out"=w1014:dbl)  [unwired: 5 in]
                n264 = local read "Get data"() -> (w1007:bool)
                n265 = call "PECT_Feature extraction.vi"("Length T/2"=w1012, "Length"=w1011, "Start 2"=w1022, "Start 1"=w1023, "Pulse signal in"=w1008) -> ("Feature extraction out"=w1013:dbl)  [unwired: 6 in]
                n266 = case shown="True" w1007 {
                  tunnel: w1034 -> [_ w1055]
                  tunnel: w1014 -> [_ w1054]
                  tunnel: w1028 -> [w1038 w1053]
                  tunnel: w1027 -> [_ w1052]
                  tunnel: w1009 -> [_ w1049]
                  tunnel: [w1038 w1051] -> w1026
                  tunnel: [_ w1050] -> w1025
                  tunnel: w1019 -> [_ w1048]
                  tunnel: w1013 -> [_ w1047]
                  tunnel: w1018 -> [w1037 w1046]
                  tunnel: w1017 -> [_ w1045]
                  tunnel: w1008 -> [_ w1044]
                  tunnel: [w1037 w1043] -> w1016
                  tunnel: [_ w1042] -> w1015
                  tunnel: w1006 -> [w1036 w1040]
                  tunnel: [w1036 w1039] -> w1005
                  frame False {
                  }
                  frame True {
                    n267 = Increment(x=w1040) -> (x+1=w1039:i32)
                    n268 = TDMS Write(0:w1053, 5:w1052, 9:w1049) -> (4:w1051:refnum<k34>, 15:w1050:errorcluster)  [unwired: 3 in, 2 out]
                    n269 = Enqueue Element(queue=w1055, element=w1054) -> ()  [unwired: 2 in, 3 out]
                    n270 = TDMS Write(0:w1046, 5:w1045, 9:w1044) -> (4:w1043:refnum<k34>, 15:w1042:errorcluster)  [unwired: 3 in, 2 out]
                    n271 = Enqueue Element(queue=w1048, element=w1047) -> ()  [unwired: 2 in, 3 out]
                    n272 = local write "Get data"(FALSE ("Acquire")) -> ()
                  }
                }
              }
            }
          }
        }
        n273 = local read "Completed"() -> (w939:bool)
        n274 = local read "Exit"() -> (w938:bool)
        n275 = Compound Arithmetic op=OR(w939, w938) -> (w937:bool)
        "No. data scan" <- w922
      }
      n276 = while {
        shift-right: [w732] -> _
        shift-left: 0 -> [w734]
        shift-right: [w731] -> _
        shift-left: 0 -> [w733]
        tunnel: w627 -> [w730]
        shift-right: [w722] -> w623
        shift-left: w640 -> [w729]
        shift-right: [w725] -> _
        shift-left: TRUE ("Output Direction") -> [w726]
        tunnel: w625 -> [w724]
        tunnel: [w723] -> w626
        tunnel: w610 -> [w717]
        tunnel: [w716] -> w609
        shift-right: [w714] -> _
        shift-left: 0 ("Out Row") -> [w715]
        shift-right: [w713] -> _
        shift-left: 0 ("Out Column") -> [w709]
        tunnel: w594 -> [w712]
        shift-right: [w710] -> w597
        shift-left: w598 -> [w711]
        shift-right: [w707] -> _
        shift-left: TRUE ("Output Direction") -> [w708]
        stop <- w727 stop-if-true
        n277 = local read "Scan"() -> (w721:bool)
        n278 = local read "Completed"() -> (w720:bool)
        n279 = Compound Arithmetic op=AND(invert w721, invert w720) -> (w719:bool)
        n280 = case shown="False" w719 {
          tunnel: w734 -> [w764 w853]
          tunnel: w733 -> [w763 w852]
          tunnel: [w762 w853] -> w732
          tunnel: [w757 w852] -> w731
          tunnel: w730 -> [w761 w847]
          tunnel: w729 -> [w760 w769]
          tunnel: [w755 w834] -> w722
          tunnel: [w742 _] -> w718
          tunnel: w726 -> [w759 w851]
          tunnel: [w758 w851] -> w725
          tunnel: w724 -> [w756 w836]
          tunnel: [w754 w847] -> w723
          tunnel: w717 -> [w753 w808]
          tunnel: [w752 w808] -> w716
          tunnel: w711 -> [w751 w768]
          tunnel: w715 -> [w750 w810]
          tunnel: w709 -> [w749 w809]
          tunnel: [w748 w810] -> w714
          tunnel: [w747 w809] -> w713
          tunnel: w712 -> [w746 w805]
          tunnel: [w745 w806] -> w710
          tunnel: w708 -> [w744 w807]
          tunnel: [w743 w807] -> w707
          frame False {
            n281 = Dequeue Element(queue=w761, timeout in ms (-1)=5000) -> (queue out=w754:refnum<queue>, element=w741:dbl)  [unwired: 1 in, 2 out]
            n282 = Dequeue Element(queue=w753, timeout in ms (-1)=5000) -> (queue out=w752:refnum<queue>, element=w739:dbl)  [unwired: 1 in, 2 out]
            n283 = call "EletoMatr_1channel.vi"("Input Array X"=w760, "Input data"=w741, "In Row"=w764, "In Column"=w763, "Input Direction"=w759) -> ("Out Array X"=w755:dbl[][], "Out Row"=w762:i32, "Output Direction"=w758:bool, "Out Column"=w757:i32)  [unwired: 6 in, 1 out]
            n284 = call "EletoMatr_1channel.vi"("Input Array X"=w751, "Input data"=w739, "In Row"=w750, "In Column"=w749, "Input Direction"=w744) -> ("Completed"=w742:bool, "Out Array X"=w745:dbl[][], "Out Row"=w748:i32, "Output Direction"=w743:bool, "Out Column"=w747:i32)  [unwired: 6 in]
            n285 = Lossy Enqueue Element(queue=w746, element=w745) -> ()  [unwired: 1 in, 4 out]
            n286 = Lossy Enqueue Element(queue=w756, element=w755) -> ()  [unwired: 1 in, 4 out]
          }
          frame True {
            n287 = local read "Offset"() -> (w841:bool)
            n288 = local read "Gate 1"() -> (w849:dbl)
            n289 = local read "Gate 2"() -> (w848:dbl)
            n290 = local read "Gate 3"() -> (w773:dbl)
            n291 = local read "Gate 4"() -> (w774:dbl)
            n292 = call "TDMS_Open.vi"("Offset"=w841, "Gate 2"=w848, "Gate 1"=w849, "Input 2D"=w769, "Open"="Open tdms") -> ("Output 2D"=w815:dbl[][])  [unwired: 5 in, 1 out]
            n293 = case shown="True" "Open tdms" {
              tunnel: w815 -> [_ w864]
              frame False {
              }
              frame True {
                n294 = global write "Global_data.vi" "global 2d graph"(w864) -> ()
              }
            }
            n295 = call "TDMS_Open.vi"("Gate 2"=w774, "Gate 1"=w773, "Input 2D"=w768, "Open"="Open tdms 2") -> ("Output 2D"=w772:dbl[][])  [unwired: 6 in, 1 out]
            n296 = case shown="True" "Open tdms 2" {
              tunnel: w772 -> [_ w854]
              frame False {
              }
              frame True {
                n297 = global write "Global_data.vi" "global 2d graph"(w854) -> ()
              }
            }
            n298 = call "RepairLine.vi"("Repair Line Col"="Repair Line Col", "Repair Line Row"="Repair Line Row", "Line Col"="Line Col", "Line Row"="Line Row", "Array In"=w815) -> ("Array Repaired"=w828:dbl[][])  [unwired: 6 in]
            n299 = call "RepairLine.vi"("Repair Line Col"="Repair Line Col 2", "Repair Line Row"="Repair Line Row 2", "Line Col"="Line Col 2", "Line Row"="Line Row 2", "Array In"=w772) -> ("Array Repaired"=w788:dbl[][])  [unwired: 6 in]
            n300 = call "CSV Open.vi"("2D Array In"=w828, "Open"="Open csv") -> ("2D Array Out"=w835:dbl[][])  [unwired: 9 in]
            n301 = call "CSV Open.vi"("2D Array In"=w788, "Open"="Open csv") -> ("2D Array Out"=w784:dbl[][])  [unwired: 9 in]
            n302 = call "Backdata.vi"("Backindex"="Backindex", "Array in"=w835, "Backdata"="Backdata") -> ("Array out"=w817:dbl[][])
            n303 = global read "Global_data.vi" "global 2d graph"() -> (w812:dbl[][])
            n304 = call "TrimXY.vi"("X-max"="Y-max", "X-min"="Y-min", "Y-max"="X-max", "Y-min"="X-min", "Array In"=w817, "Trim data"="Trim data") -> ("Array Trim Out"=w816:dbl[][])  [unwired: 5 in]
            n305 = call "Backdata.vi"("Backindex"="Backindex 2", "Array in"=w784, "Backdata"="Backdata 2") -> ("Array out"=w799:dbl[][])
            n306 = call "Inverse.vi"(10:"Inverse"=w816, 11:"Inverse"="Inverse") -> ("Array out"=w813:dbl[][])  [unwired: 9 in]
            n307 = call "TrimXY.vi"("X-max"="Y-max 2", "X-min"="Y-min 2", "Y-max"="X-max 2", "Y-min"="X-min 2", "Array In"=w799, "Trim data"="Trim data 2") -> ("Array Trim Out"=w800:dbl[][])  [unwired: 5 in]
            n308 = global read "Global_data.vi" "global 2d graph"() -> (w771:dbl[][])
            n309 = call "Return data.vi"("Array Return"=w812, "Array Input"=w813, "Return"="Return") -> ("Array out"=w811:dbl[][])  [unwired: 8 in]
            n310 = call "Abs.vi"("Input"=w811, "Abs"="Abs") -> ("Array out"=w840:dbl[][])  [unwired: 9 in]
            n311 = call "DiffX.vi"("Array in"=w840, "DiffX"="DiffX") -> ("Array out"=w845:dbl[][])  [unwired: 1 in]
            n312 = call "Inverse.vi"(10:"Inverse"=w800, 11:"Inverse"="Inverse  2") -> ("Array out"=w802:dbl[][])  [unwired: 9 in]
            n313 = call "DiffY.vi"("Array in"=w845, "DiffY"="DiffY") -> ("Array out"=w843:dbl[][])  [unwired: 1 in]
            n314 = call "Return data.vi"("Array Return"=w771, "Array Input"=w802, "Return"="Return 2") -> ("Array out"=w803:dbl[][])  [unwired: 8 in]
            n315 = call "Abs.vi"("Input"=w803, "Abs"="Abs 2") -> ("Array out"=w780:dbl[][])  [unwired: 9 in]
            n316 = call "DiffX.vi"("Array in"=w780, "DiffX"="DiffX 2") -> ("Array out"=w776:dbl[][])  [unwired: 1 in]
            n317 = call "DiffY.vi"("Array in"=w776, "DiffY"="DiffY 2") -> ("Array out"=w778:dbl[][])  [unwired: 1 in]
            n318 = call "Odd.vi"("Odd"="Odd", "Array In"=w843) -> ("Array Out"=w832:dbl[][])  [unwired: 9 in]
            n319 = call "Odd.vi"("Odd"="Odd 2", "Array In"=w778) -> ("Array Out"=w785:dbl[][])  [unwired: 9 in]
            n320 = call "Filter_Lowpass - 2D.vi"("Filter"="Filter", "Input 2D"=w832, "low cutoff freq: fl"="low cutoff freq: fl") -> ("Output"=w831:dbl[][])  [unwired: 6 in]
            n321 = call "Filter_Lowpass - 2D.vi"("Filter"="Filter 3", "Input 2D"=w785, "low cutoff freq: fl"="low cutoff freq: fl 3") -> ("Output"=w770:dbl[][])  [unwired: 6 in]
            n322 = case shown="True" TRUE {
              tunnel: w831 -> [w865 w866]
              tunnel: [w865 w866] -> w834
              tunnel: w836 -> [_ w867]
              frame False {
              }
              frame True {
                n323 = local read "3D Surface(0) (coil)"() -> (w871:refnum<k7>)
                n324 = Matrix Size(0:w866) -> (1:w872:i32, 2:w869:i32)
                n325 = Decrement(x=w872) -> (x-1=w870:i32)
                n326 = Decrement(x=w869) -> (x-1=w868:i32)
                n327 = call "Surface_AxesScale.vi"("Y-axis Max"=w868, "X-axis max"=w870, "3D Surface"=w871, "Auto Scale"=FALSE) -> ()  [unwired: 8 in]
                n328 = Lossy Enqueue Element(queue=w867, element=w866) -> ()  [unwired: 1 in, 4 out]
              }
            }
            n329 = case shown="True" TRUE {
              tunnel: w770 -> [w855 w857]
              tunnel: [w855 w857] -> w806
              tunnel: w805 -> [_ w856]
              frame False {
              }
              frame True {
                n330 = local read "3D Surface (2)(Hall)"() -> (w861:refnum<k7>)
                n331 = Matrix Size(0:w857) -> (1:w862:i32, 2:w859:i32)
                n332 = Decrement(x=w862) -> (x-1=w860:i32)
                n333 = Decrement(x=w859) -> (x-1=w858:i32)
                n334 = call "Surface_AxesScale.vi"("Y-axis Max"=w858, "X-axis max"=w860, "3D Surface"=w861, "Auto Scale"=FALSE) -> ()  [unwired: 8 in]
                n335 = Lossy Enqueue Element(queue=w856, element=w857) -> ()  [unwired: 1 in, 4 out]
              }
            }
            n336 = Wait Until Next ms Multiple(millisecond multiple=u32 100 ("ms 배수")) -> ()  [unwired: 1 out]
          }
        }
        "Output Coil" <- w722
        "Out Hall" <- w710
        n337 = case shown="True" w718 {
          selector: w718 -> [w735 w736]
          tunnel: [w735 w736] -> w706
          frame False {
          }
          frame True {
            n338 = Wait (ms)(milliseconds to wait=u32 200) -> ()  [unwired: 1 out]
          }
        }
        "Completed" <- w706
        n339 = local read "Exit"() -> (w728:bool)
        n340 = Compound Arithmetic op=OR(w706, w728) -> (w727:bool)
        "No. Y" <- w733
        "No. X" <- w734
        "No. Y 2" <- w709
      }
      n341 = while {
        tunnel: w625 -> [w703]
        tunnel: [w700] -> w624
        tunnel: w594 -> [w681]
        tunnel: [w680] -> w593
        stop <- w701 stop-if-true
        n342 = local read "Out Hall"() -> (w689:dbl[][])
        n343 = local read "Output Coil"() -> (w691:dbl[][])
        n344 = local read "No. Y 2"() -> (w685:i32)
        n345 = call "CursorPosition.vi"("Cursor No."=1.0, "Cursor"="Cursor 2", "3D Surface Analysis"="3D Surface (2)(Hall)") -> ("Cursor Y"=w688:dbl)  [unwired: 6 in, 2 out]
        n346 = local read "No. Y"() -> (w698:i32)
        n347 = call "CursorPosition.vi"("Cursor No."=1.0, "Cursor"="Cursor", "3D Surface Analysis"="3D Surface(0) (coil)") -> ("Cursor Y"=w693:dbl)  [unwired: 6 in, 2 out]
        n348 = Dequeue Element(queue=w681, timeout in ms (-1)=3000) -> (queue out=w680:refnum<queue>)  [unwired: 1 in, 3 out]
        n349 = Add(x=w685, y=w688) -> (x+y=w686:dbl)
        n350 = Dequeue Element(queue=w703, timeout in ms (-1)=3000) -> (queue out=w700:refnum<queue>)  [unwired: 1 in, 3 out]
        n351 = Add(x=w698, y=w693) -> (x+y=w697:dbl)
        n352 = Index Array(array=w689, index (col)=w686) -> (element=→"Feature extraction scan Hall":dbl[])  [unwired: 1 in]
        n353 = Index Array(array=w691, index (col)=w697) -> (element=→"Feature extraction scan Coil":dbl[])  [unwired: 1 in]
        n354 = call <vilib>:"3D Surface.vi"("z matrix"=w689, "3D graph"="3D Surface (2)(Hall)") -> ()  [unwired: 8 in, 2 out]
        n355 = call <vilib>:"3D Surface.vi"("z matrix"=w691, "3D graph"="3D Surface(0) (coil)") -> ()  [unwired: 8 in, 2 out]
        n356 = local read "Completed"() -> (w699:bool)
        n357 = local read "Exit"() -> (w702:bool)
        n358 = Compound Arithmetic op=OR(w699, w702) -> (w701:bool)
        n359 = Wait Until Next ms Multiple(millisecond multiple=u32 100 ("ms 배수")) -> ()  [unwired: 1 out]
      }
      n360 = Release Queue(queue=w624) -> ()  [unwired: 2 in, 3 out]
      n361 = Release Queue(queue=w593) -> ()  [unwired: 2 in, 3 out]
      n362 = TDMS Close(8:w613, 11:w614) -> (0:w615:errorcluster)  [unwired: 1 out]
      n363 = call <vilib>:"Simple Error Handler.vi"("error in (no error)"=w615) -> ()  [unwired: 2 in, 7 out]
      n364 = TDMS Close(8:w630, 11:w631) -> (0:w628:errorcluster)  [unwired: 1 out]
      n365 = while {
        stop <- w658 stop-if-true
        n366 = event shown="[2] \"Max\", \"Min\", \"ColorMapAutoScale\": Value Change" {
          selector: _ -> [_ _ _]
          dyn-events: _ -> [_ _ _]
          timeout: _ -> [_ _ _]
          tunnel: [_ w663 _] -> w658
          event "Plot style", "ViewMode": Value Change {
            n367 = event-data() -> ()  [unwired: 1 in, 2 out]
            n368 = local read "3D Surface (2)(Hall)"() -> (w661:refnum<k7>)
            n369 = local read "3D Surface(0) (coil)"() -> (w662:refnum<k7>)
            n370 = property class="CWGraph3D"(reference=w661, "ViewMode"="ViewMode") -> ()  [unwired: 1 in, 2 out]
            n371 = call <vilib>:"Basic Properties.vi"("3D graph"=w661, "plot style"="Plot style") -> ()  [unwired: 12 in, 2 out]
            n372 = property class="CWGraph3D"(reference=w662, "ViewMode"="ViewMode") -> ()  [unwired: 1 in, 2 out]
            n373 = call <vilib>:"Basic Properties.vi"("3D graph"=w662, "plot style"="Plot style") -> ()  [unwired: 12 in, 2 out]
          }
          event "Exit": Value Change {
            n374 = event-data() -> ()  [unwired: 1 in, 1 out]
            n375 = local read "Exit"() -> (w663:bool)
          }
          event "Max", "Min", "ColorMapAutoScale": Value Change {
            n376 = event-data() -> ()  [unwired: 1 in, 5 out]
            n377 = local read "3D Surface (2)(Hall)"() -> (w664:refnum<k7>)
            n378 = local read "3D Surface(0) (coil)"() -> (w670:refnum<k7>)
            n379 = call "Surface_ColorScale.vi"("ColorMapAutoScale"="ColorMapAutoScale 2", "Min"="Min 2", "Max"="Max 2", "3D Surface_"=w664) -> ("Min 2"=w668:dbl, "Max 2"=w667:dbl)  [unwired: 1 in, 2 out]
            n380 = call "Surface_ColorScale.vi"("ColorMapAutoScale"="ColorMapAutoScale", "Min"="Min", "Max"="Max", "3D Surface_"=w670) -> ("Min 2"=w674:dbl, "Max 2"=w673:dbl)  [unwired: 1 in, 2 out]
            n381 = local write "Min 2"(w668) -> ()
            n382 = local write "Max 2"(w667) -> ()
            n383 = local write "Max"(w673) -> ()
            n384 = local write "Min"(w674) -> ()
          }
        }
      }
      n385 = Release Queue(queue=w609) -> ()  [unwired: 2 in, 3 out]
      n386 = call <vilib>:"Simple Error Handler.vi"("error in (no error)"=w628) -> ()  [unwired: 2 in, 7 out]
      n387 = while {
        tunnel: w597 -> [w656]
        stop <- w655 stop-if-true
        n388 = call "CSV Save.vi"("Array"=w656, "Save Button"="Save Scan mode 2") -> ()  [unwired: 9 in, 1 out]
        n389 = Wait Until Next ms Multiple(millisecond multiple=u32 100 ("ms 배수")) -> ()  [unwired: 1 out]
        n390 = local read "Exit"() -> (w655:bool)
      }
      n391 = Release Queue(queue=w626) -> ()  [unwired: 2 in, 3 out]
      n392 = while {
        tunnel: w623 -> [w678]
        stop <- w677 stop-if-true
        n393 = call "CSV Save.vi"("Array"=w678, "Save Button"="Save Scan mode") -> ()  [unwired: 9 in, 1 out]
        n394 = Wait Until Next ms Multiple(millisecond multiple=u32 100 ("ms 배수")) -> ()  [unwired: 1 out]
        n395 = local read "Exit"() -> (w677:bool)
      }
    }
    frame "Lift-Off" {
      n396 = while {
        shift-right: [w1067] -> _
        shift-left: "2D Array In" -> [w1068]
        stop <- w1072 stop-if-true
        n397 = call "CSV Open.vi"("2D Array In"=w1068, "Open"="Open") -> ("2D Array Out"=w1067:dbl[][])  [unwired: 9 in]
        n398 = Delete From Array(array=w1067, index (col)=0 ("disabled index (col)")) -> (array with subset deleted=w1069:dbl[][])  [unwired: 2 in, 1 out]
        n399 = Subtract(x=w1069, y=w1067) -> (x-y=w1065:dbl[][])
        n400 = Transpose 2D Array(2D array=w1065) -> (transposed array=w1062:dbl[][])
        n401 = call "Filter_Lowpass - 2D.vi"("Filter"="Filter lf", "Input 2D"=w1062, "low cutoff freq: fl"="Low cutoff freq: fl") -> ("Output"=w1064:dbl[][])  [unwired: 6 in]
        n402 = Transpose 2D Array(2D array=w1064) -> (transposed array=w1061:dbl[][])
        n403 = Select(t=w1061, s="View Mode", f=w1067) -> (s? t:f=→"Hall sensors signal lf":dbl[][])
        n404 = local read "Exit"() -> (w1072:bool)
      }
    }
    frame "Test mode                   " {
      n405 = while {
        tunnel: w1092 -> [w1128]
        tunnel: w1088 -> [w1127]
        tunnel: [w1145] -> w1090
        tunnel: [w1146] -> w1091
        shift-right: [w1141] -> _
        shift-left: w1089 -> [w1142]
        tunnel: w1089 -> [w1140]
        shift-right: [w1138] -> _
        shift-left: _ -> [w1137]
        tunnel: w1087 -> [w1136]
        shift-right: [w1135] -> _
        shift-left: _ -> [w1134]
        shift-right: [w1132] -> _
        shift-left: 1 ("Average") -> [w1131]
        tunnel: w1085 -> [w1124]
        tunnel: w1084 -> [w1123]
        tunnel: w1080 -> [w1122]
        tunnel: w1083 -> [w1120]
        shift-right: [w1118] -> _
        shift-left: dbl[][] [] -> [w1119]
        shift-right: [w1117] -> _
        shift-left: dbl[] [] -> [w1116]
        shift-right: [w1113] -> _
        shift-left: _ -> [w1114]
        shift-right: [w1111] -> _
        shift-left: _ -> [w1112]
        shift-right: [w1108] -> _
        shift-left: dbl[][] [] -> [w1109]
        shift-right: [w1102] -> _
        shift-left: w1077 -> [w1106]
        shift-right: [w1101] -> _
        shift-left: dbl[] [] -> [w1104]
        tunnel: w1077 -> [w1103]
        tunnel: w1076 -> [w1100]
        tunnel: w1075 -> [w1099]
        tunnel: w1074 -> [w1098]
        tunnel: w1073 -> [w1097]
        stop <- w1147 stop-if-true
        # "Coil"
        n406 = First Call?() -> (First Call?: T/F=w1129:bool)
        n407 = case shown="True" w1129 {
          tunnel: w1128 -> [w1148 w1153]
          tunnel: w1127 -> [w1149 w1152]
          tunnel: [w1148 w1151] -> w1126
          tunnel: [w1149 w1150] -> w1125
          frame False {
          }
          frame True {
            n408 = call <vilib>:"DAQmx Start Task.vi"("task/channels in"=w1153, "error in"=w1152) -> ("task out"=w1151:refnum<k21>, "error out"=w1150:errorcluster)  [unwired: 12 in]
          }
        }
        n409 = local read "Pulser Cycles"() -> (w1130:i32)
        n410 = call-poly <vilib>:"DAQmx Read.vi"("task/channels in"=w1126, "number of samples per channel"=w1120, "error in"=w1125) -> ("task out"=w1146:refnum<k21>, "data"=w1115:waveform(dbl)[], "error out"=w1145:errorcluster)  [unwired: 10 in]
        n411 = Quotient & Remainder(x=w1131, y=w1130) -> (x-y*floor(x/y)=w1143:i32)  [unwired: 1 out]
        n412 = Index Array(array=w1115, index #1=2 ("index"), index #2=0 ("index (row)")) -> (element #1=w1093:waveform(dbl), element #2=w1094:waveform(dbl))
        n413 = Unbundle By Name(w1093) -> ("Y"=w1107:dbl[])
        n414 = Unbundle By Name(w1094) -> ("Y"=w1110:dbl[])
        n415 = Add(x=w1107, y=w1106) -> (x+y=w1105:dbl[])
        n416 = Equal To 0?(x=w1143) -> (x = 0?=w1121:bool)
        n417 = Add(x=w1110, y=w1142) -> (x+y=w1139:dbl[])
        n418 = case shown="True" w1121 {
          tunnel: w1130 -> [_ w1166]
          tunnel: w1094 -> [_ w1227]
          tunnel: w1139 -> [w1165 w1234]
          tunnel: [w1165 w1233] -> w1141
          tunnel: w1140 -> [_ w1233]
          tunnel: [w1164 w1183] -> w1138
          tunnel: w1137 -> [w1164 w1232]
          tunnel: w1136 -> [_ w1171]
          tunnel: [w1163 w1230] -> w1135
          tunnel: w1134 -> [w1163 w1231]
          tunnel: [w1161 1 ("Average")] -> w1132
          tunnel: w1131 -> [w1162 _]
          tunnel: w1124 -> [_ w1172]
          tunnel: w1123 -> [_ w1174]
          tunnel: w1122 -> [_ w1173]
          tunnel: [w1160 w1222] -> w1118
          tunnel: w1119 -> [w1160 w1221]
          tunnel: [w1159 w1217] -> w1117
          tunnel: w1116 -> [w1159 w1216]
          tunnel: w1093 -> [_ w1208]
          tunnel: w1114 -> [w1157 w1206]
          tunnel: [w1157 w1205] -> w1113
          tunnel: w1112 -> [w1158 w1203]
          tunnel: [w1158 w1182] -> w1111
          tunnel: w1109 -> [w1154 w1196]
          tunnel: [w1154 w1195] -> w1108
          tunnel: w1105 -> [w1155 w1194]
          tunnel: w1104 -> [w1156 w1189]
          tunnel: w1103 -> [_ w1188]
          tunnel: [w1155 w1188] -> w1102
          tunnel: [w1156 w1187] -> w1101
          tunnel: w1100 -> [_ w1170]
          tunnel: w1099 -> [_ w1169]
          tunnel: w1098 -> [_ w1167]
          tunnel: w1097 -> [_ w1168]
          frame False {
            n419 = Increment(x=w1162) -> (x+1=w1161:i32)
          }
          frame True {
            n420 = Divide(x=w1194, y=w1166) -> (x/y=w1186:dbl[])
            n421 = Divide(x=w1234, y=w1166) -> (x/y=w1215:dbl[])
            n422 = local read "Offset"() -> (w1175:bool)
            n423 = call "PECT_Feature extraction.vi"("Length T/2"=w1168, "Offset"=w1175, "Length"=w1167, "Start 2"=w1169, "Start 1"=w1170, "Pulse signal in"=w1186) -> ("Feature extraction out"=→"Feature Extraction Coil":dbl)  [unwired: 5 in]
            n424 = call "PECT_Feature extraction.vi"("Length T/2"=w1171, "Offset"="Offset", "Length"=w1172, "Start 2"=w1173, "Start 1"=w1174, "Pulse signal in"=w1215) -> ("Feature extraction out"=→"Feature Extraction Hall":dbl)  [unwired: 5 in]
            n425 = case shown="True" "Backdata" {
              tunnel: w1215 -> [w1259 w1262]
              tunnel: [w1259 w1260] -> w1217
              tunnel: w1216 -> [_ w1260]
              tunnel: [w1259 w1261] -> w1212
              frame False {
              }
              frame True {
                n426 = Subtract(x=w1262, y=w1260) -> (x-y=w1261:dbl[])
              }
            }
            n427 = case shown="True" "Backdata 3" {
              tunnel: w1186 -> [w1241 w1244]
              tunnel: [w1241 w1242] -> w1187
              tunnel: w1189 -> [_ w1242]
              tunnel: [w1241 w1243] -> w1193
              frame False {
              }
              frame True {
                n428 = Subtract(x=w1244, y=w1242) -> (x-y=w1243:dbl[])
              }
            }
            n429 = call "Filter_Lowpass.vi"("Filter"="Filter 2", "Pulse signal in"=w1212, "low cutoff freq: fl"="low cutoff freq: fl 2") -> ("Signal out"=w1211:dbl[])  [unwired: 6 in]
            n430 = Bundle By Name(cluster=w1227, "Y"=w1211) -> (w1220:waveform(dbl))
            n431 = call-poly <vilib>:"FFT Power Spectrum and PSD.vi"("time signal"=w1220) -> ("Power Spectrum / PSD"=w1219:cluster{"f0":dbl, "df":dbl, "magnitude":dbl[]})  [unwired: 7 in, 3 out]
            n432 = case shown="True" "2 Plots" {
              tunnel: [w1270 w1276] -> w1179
              tunnel: w1232 -> [_ w1275]
              tunnel: [w1267 w1275] -> w1183
              tunnel: w1220 -> [w1267 w1271]
              tunnel: w1219 -> [w1268 w1273]
              tunnel: [w1269 w1274] -> w1228
              tunnel: w1231 -> [_ w1272]
              tunnel: [w1268 w1272] -> w1230
              frame False {
                n433 = Build Array(w1268, w1268) -> (w1269:cluster{"f0":dbl, "df":dbl, "magnitude":dbl[]}[])
                n434 = Build Array(w1267, w1267) -> (w1270:waveform(dbl)[])
              }
              frame True {
                n435 = Build Array(w1272, w1273) -> (w1274:cluster{"f0":dbl, "df":dbl, "magnitude":dbl[]}[])
                n436 = Build Array(w1275, w1271) -> (w1276:waveform(dbl)[])
              }
            }
            "Power spectral density Hall" <- w1228
            n437 = case shown="True" "Add LF" {
              tunnel: w1211 -> [_ w1266]
              tunnel: [w1263 w1264] -> w1222
              tunnel: w1221 -> [w1263 w1265]
              frame False {
              }
              frame True {
                n438 = Build Array (concatenate)(w1265, w1266) -> (w1264:dbl[][])
              }
            }
            n439 = call "Filter_Lowpass.vi"("Filter"="Filter 4", "Pulse signal in"=w1193, "low cutoff freq: fl"="low cutoff freq: fl 4") -> ("Signal out"=w1184:dbl[])  [unwired: 6 in]
            n440 = Bundle By Name(cluster=w1208, "Y"=w1184) -> (w1202:waveform(dbl))
            n441 = call-poly <vilib>:"FFT Power Spectrum and PSD.vi"("time signal"=w1202) -> ("Power Spectrum / PSD"=w1207:cluster{"f0":dbl, "df":dbl, "magnitude":dbl[]})  [unwired: 7 in, 3 out]
            n442 = case shown="True" "Add LF" {
              tunnel: w1184 -> [_ w1248]
              tunnel: [w1245 w1246] -> w1195
              tunnel: w1196 -> [w1245 w1247]
              frame False {
              }
              frame True {
                n443 = Build Array (concatenate)(w1247, w1248) -> (w1246:dbl[][])
              }
            }
            n444 = case shown="True" "2 Plots" {
              tunnel: [w1252 w1258] -> w1177
              tunnel: w1203 -> [_ w1254]
              tunnel: [w1249 w1254] -> w1182
              tunnel: w1202 -> [w1249 w1253]
              tunnel: w1207 -> [w1250 w1256]
              tunnel: [w1251 w1257] -> w1204
              tunnel: w1206 -> [_ w1255]
              tunnel: [w1250 w1255] -> w1205
              frame False {
                n445 = Build Array(w1250, w1250) -> (w1251:cluster{"f0":dbl, "df":dbl, "magnitude":dbl[]}[])
                n446 = Build Array(w1249, w1249) -> (w1252:waveform(dbl)[])
              }
              frame True {
                n447 = Build Array(w1255, w1256) -> (w1257:cluster{"f0":dbl, "df":dbl, "magnitude":dbl[]}[])
                n448 = Build Array(w1254, w1253) -> (w1258:waveform(dbl)[])
              }
            }
            "Power spectral density Coil" <- w1204
            n449 = local read "Tab plot"() -> (w1176:enum32{"Raw Signal Plot", "Phase Plot"})
            n450 = call "CSV Save.vi"("Array"=w1195, "Save Button"="Save LF") -> ("Save Status"=→"Save Status 2":bool)  [unwired: 9 in]
            n451 = call "CSV Save.vi"("Array"=w1222, "Save Button"="Save LF") -> ("Save Status"=→"Save Status":bool)  [unwired: 9 in]
            n452 = case shown="\"Phase Plot\"" "Tab plot" {
              tunnel: w1183 -> [_ w1240]
              tunnel: w1179 -> [w1238 _]
              frame "Raw Signal Plot", Default {
                "Hall sensors signal" <- w1238
              }
              frame "Phase Plot" {
                n453 = call "Phase Function.vi"("waveform"=w1240) -> ("Single Hall Phase"=→"Phase - Single Hall (0)":cluster{dbl[], "Signal out":dbl[]}[])  [unwired: 9 in, 1 out]
              }
            }
            n454 = case shown="\"Phase Plot\"" w1176 {
              tunnel: w1182 -> [_ w1237]
              tunnel: w1177 -> [w1235 _]
              frame "Raw Signal Plot", Default {
                "Coil signal" <- w1235
              }
              frame "Phase Plot" {
                n455 = call "Phase Function.vi"("waveform"=w1237) -> ("Single Hall Phase"=→"Phase - Differential Hall (2)":cluster{dbl[], "Signal out":dbl[]}[])  [unwired: 9 in, 1 out]
              }
            }
            n456 = Delete From Array(array=w1195, index (col)=0 ("disabled index (col)")) -> (array with subset deleted=w1199:dbl[][])  [unwired: 2 in, 1 out]
            n457 = Delete From Array(array=w1222, index (col)=0 ("disabled index (col)")) -> (array with subset deleted=w1223:dbl[][])  [unwired: 2 in, 1 out]
            n458 = Subtract(x=w1199, y=w1195) -> (x-y=→"dy 2":dbl[][])
            n459 = Subtract(x=w1223, y=w1222) -> (x-y=→"dy":dbl[][])
          }
        }
        n460 = local read "Exit"() -> (w1133:bool)
        n461 = Unbundle By Name(w1145) -> ("status"=w1144:bool)
        n462 = Or(x=w1144, y=w1133) -> (x .or. y?=w1147:bool)
      }
    }
  }
  n463 = call <vilib>:"DAQmx Clear Task.vi"("task in"=w93, "error in"=w92) -> ("error out"=w99:errorcluster)  [unwired: 13 in]
  n464 = call <vilib>:"Simple Error Handler.vi"("error in (no error)"=w99) -> ()  [unwired: 4 in, 5 out]
  n465 = call <vilib>:"Simple Error Handler.vi"() -> ()  [unwired: 5 in, 5 out]
  "Init pulses" <- 0 ("Init pulses")
